vi "Doppler.vi"(0 "Choose Directory":path=path "F:/VectorFlowMice") -> ()   [LabVIEW 2022 SP3]
uses:
  <vilib>/Math Plots/3D Math Plots/3D Surface/3D Surface XCtrl/3D Surface.xctl
  -planewaveSubs/DopplerParams.ctl
  -planewaveSubs/DopThresholds.ctl
  ViewData/-ReadEye/Header.ctl
  <vilib>/Analysis/baseanly.llb/Mean (DBL).vi
  <vilib>/Analysis/baseanly.llb/Quick Scale 1D.vi
  <vilib>/Analysis/2dsp.llb/2D Cross Correlation (DBL).vi
  <vilib>/Analysis/2dsp.llb/FFT.vi
  <vilib>/Analysis/2dsp.llb/Complex FFT.vi
  <vilib>/Analysis/8numeric.llb/Numeric Integration.vi
  <vilib>/Analysis/8numeric.llb/1D Numeric Integration.vi
  <vilib>/Analysis/4window.llb/Hamming Window.vi
  <vilib>/Analysis/4window.llb/Hamming Window (CDB).vi
  -planewaveSubs/LagOneAutoCorr.vi
  <vilib>/Analysis/4window.llb/AllCosWindow (CDB).vi
  <vilib>/Analysis/1siggen.llb/Ramp Pattern by Delta.vi
  <vilib>/Analysis/3filter.llb/Butterworth Filter.vi
  <vilib>/Analysis/3filter.llb/Butterworth Filter (CDB).vi
  <vilib>/Analysis/3filter.llb/Equi-Ripple HighPass.vi
  <vilib>/Analysis/3filter.llb/Equi-Ripple HighPass (CDB).vi
  <vilib>/picture/picture.llb/Draw True-Color Pixmap.vi
  <vilib>/Utility/file.llb/Write Delimited Spreadsheet (DBL).vi
  <vilib>/Utility/file.llb/Write Delimited Spreadsheet (string).vi
  <vilib>/Math Plots/3D Math Plots/3D Surface/3D Surface Datatype/Public/Plot Helper (Matrix).vi
  <vilib>/Analysis/NI_AALBase.lvlib
  <vilib>/Analysis/NI_AALPro.lvlib
  <vilib>/Analysis/NI_AAL_SigProc.lvlib
  <vilib>/Math Plots/3D Math Plots/3D Surface/3D Surface Datatype/3D Surface Datatype.lvclass
panel:
  out "PowerRaw":sgl[][](array[numeric])
  out "Original Fc":sgl
  in  "True Center Freq":dbl=15.5
  in  "file ext search":string="*_HeaderInfoRcv.txt"
  in  "Header Out":T1={"header info"={"Header"="", "Head length"=0}, "A/D info"={"# rf points per line"=0, "# lines per scan"=0, "sample rate MHz"=0, "# A/D bits"=0, "# bytes per A/D"=0, "TGC Flag"=0, "A/D Type"=""}, "Tranducer Info"={"bandwidth"=0.0, "center freq"=0.0, "start freq"=0.0, "ID"=0}, "Scan Info"={"delay"=0.0, "pivot distance"=0.0, "sector scan angle"=0.0, "operator"="", "Scan Mode"="", "location"=""}, "Time/Date Info"={"date"="", "time"=""}, "RF Info"={"RF file name"="", "RF file att"="", "RF cal file name"="", "RF cal file att"=""}, "Patient Info"={"ID"="", "extended ID"="", "age"=0, "sex"="", "previously\nscanned"="", "PSA"=0.0, "LOS"=1, "Ethnicty 2"=3, "Race"=3}, "Tissue Type"={"organ"=0, "disease type"=0, "disease location"=0, "IQ_pts"=0, "RcvBuffer"=0, "RcvFrame"=0, "IQBuff"=0, "IQFrame"=0, "IQPage"=0}, "Votage scaling"={"Digitizer (dB)"=0.0, "Gain (dB)"=0.0, "Atten (dB)"=0.0}, "Comment"="", "Misc Info"={"avg num"=0, "c speed"=0, "Div By or SF zones"=0, "XMIT CHS"=0, "RCV CHS"=0, "Xmit angle"=0.0}, "Therapy Parameters"={"Theraputic Freq (MHz)"=0.0, "Time on (s)"=0.0, "Therapy amplitude (mV)"=0.0, "Lines Before"=0, "Lines After"=0}, "Scan Settings"={"Energy (uJ or V)"=0, "Damp (Ohm) or Fc"=0, "HP Filt (KHz)"=0, "LP Filt (MHz)"=0, "Gain (db)"=0, "prf (kHz)"=0.0, "Distance between\nscan lines (um)"=0, "Distance between\nscan planes (um)"=0, "Scan line gap (um)"=0.0, "Scan plane gap (um)"=0.0}, "Compression Parameters"={"F1 (MHz)"=0.0, "F2 (MHz)"=0.0, "% taper"=0.0, "duration"=0.0}, "Patient Info Xtra"={"First Name"="", "Last Name"="", "Notes"=""}, "ROI Box"=[0, 0, 0, 0]} {"Compression Parameters"."% taper" min=50 max=1000 format="%.2f"; "Compression Parameters"."F2 (MHz)" format="%.3f"; "Compression Parameters"."F1 (MHz)" format="%.3f"; "Scan Settings"."prf (kHz)" format="%.2f"; "Therapy Parameters"."Therapy amplitude (mV)" min=50 max=1000 format="%.2f"; "Therapy Parameters"."Time on (s)" format="%.3f"; "Therapy Parameters"."Theraputic Freq (MHz)" format="%.3f"; "Patient Info"."Race" items=["Am Ind or Alaska", "Asian", "Hawaiian, Pac Isl", "Black or Afr Amer", "White", "more than one race", "unknown"]; "Patient Info"."Ethnicty 2" items=["Hispanic", "Non-Hispanic", "unknown"]; "Patient Info"."LOS" items=["1", "2", "3", "4", "5"]; "Patient Info"."PSA" format="%.1f"; "Scan Info"."delay" format="%.2f"; "Scan Info"."pivot distance" format="%.2f"; "Scan Info"."sector scan angle" format="%.2f"; "Tranducer Info"."bandwidth" format="%.2f"; "Tranducer Info"."center freq" format="%.2f"; "Tranducer Info"."start freq" format="%.2f"}
  in  "Use Selected Files":bool
  in  "File Select":i32[](listbox)
  out "max value":sgl
  in  "RF Average Window":i32=3
  out "max doppler\nV cm/s":dbl
  out "Slow time\nsampling":sgl
  in  "image to display":i32
  in  "start":i32
  in  "Doppler Params":T2={"Dopp Filter Order"=133, "Window length"=64, "Window Increment"=8, "Start f"=0.05, "lDoppler cutouff"=0.1, "FFT Length"=128, "SlowTime (Hz)"=100.0} {"Start f" format="%0.3f"; "SlowTime (Hz)" format="%0.1f"; "lDoppler cutouff" format="%0.3f"}
  out "Total Files":i32
  in  "# of files":i32=1000
  out "Raw data":dbl[][](graph)
  in  "Tab Control":T3(tab)
  in  "Alias Correct":bool
  in  "Save Vels":bool
  in  "SaveSpectrogram":bool
  in  "phase scale":dbl=1.0
  out "phase":dbl[][](graph)
  out "Spectrum":dbl[](graph)
  out "Velocity":dbl[](graph)
  in  "Thresholds":T4={"Spec Ratio Threshold"=0.2999999999999998, "V Threshold"=-25.0, "Power Threshold"=0.0, "RF Threshold"=25000.0}
  out "Total Power":sgl[](graph)
  out "Spec ratio":sgl[](graph)
  out "Row Cropped data":dbl[][](graph)
  out "Slow time of red line":dbl[][](graph)
  out "Doppler Signal":dbl[][](graph)
  out "Dop Spec":dbl[][](graph)
  in  "SVD zeros":i32
  in  "SVD?":bool
  in  "maxPRF?":bool
  in  "Log RF?":bool=TRUE
  out "bandwidths":sgl[](graph)
  out "error":i32
  in  "Clip":i32
  out "Vel Mean":dbl format="%0.2f"
  out "Sum Power":sgl
  in  "Lag Overlay off?":bool
  out "BPM":i32
  in  "Cycles":i32=1
  in  "width":i32=25 min=3
  in  "threshold":dbl=0.35 format="%0.2f"
  in  "Batch BPM":bool
  out "# found":i32[](array[numeric])
  out "BPM auto":i32[](array[numeric])
  in  "Freeze BPM":bool
  out "BPS":sgl
  in  "Note":string
  out "LagOne":dbl
  in  "Save Single SpGram":bool
  in  "Save Animation":bool
  out "Slow time mean":dbl[](graph)
  out "Spectrogram at marker":sgl[][](graph)
  out "Slow Time V values at Red cursor":dbl[](graph)
  in  "Scale Type":enum32{"Max/Min", "Max/Zero", "Min/Zero"}(radio)
  out "Peak V":dbl[][](graph)
  in  "animate":bool
  in  "ms between frames":u32=10
  in  "Calc Spec Peaks":bool
  out "AVG of all windows":dbl[][](graph)
  in  "Doppler Angle":dbl
  in  "AVG Thresh":dbl=20.0
  out "V mean":dbl format="%0.2f"
  out "V SD":dbl format="%0.2f"
  in  "Z Scale":dbl(slide) scale=0.0..50.0
  in  "Queue processing":bool
  out "Overlay":i16[][](graph)
  in  "dB Max":dbl=50.0
  in  "Med Size":i32=3
  in  "Spectrogram average":i32=3
  out "Dop Spectrum":sgl[](graph)
  in  "dB width pt":dbl
  in  "ST AV depth":i32=10
  out "Sets":i32
  out "Current":i32
  out "Raw uncropped image":dbl[][](graph)
  out "Waveform Graph":i32[](graph)
  out "2D corr":dbl[][](graph)
  out "Mean Power":sgl[][](graph)
  out "Slow Time V values at Red cursor Mean Power":dbl[](graph)
  out "Simple Motion Tracker":cluster{"2D Corr":dbl[], "2D Corr":dbl[]}(graph)
  in  "#x lines":i32=10
  in  "#y rf":i32=25
  in  "Ref Place for 2S":i32
  in  "2D threshold":sgl
  in  "Save Motion":bool
  out "M-mode x":dbl[][](graph)
  in  "Save M-mode":bool
  in  "Divide down":i32=50 min=1
  out "Avergae V Profile All":dbl[](graph)
  out "Avergae V Profile (Tube)":dbl[](graph)
  in  "index":i32
  in  "length":i32
  out "3D Surface":refnum<class "3D Plot Datatype.lvclass">[](xcontrol)
  out "High pass Filtered log":sgl[][](graph)
  in  "CFiltered data":bool
  in  "C Corr":bool
  out "Cross Correlate":sgl[][](graph)
  out "Cross Correlate":sgl[][][](array[numeric])
  out "HIgh pass Filtered X":sgl[][][](array[numeric])
  out "Raw High pass filtered":sgl[][](graph)
  out "Row Cropped data save":dbl[][](graph)
  out "Doppler Spec For Save":dbl[][](graph)
  out "Smoothed Data":dbl[][][](array[numeric])
  out "Raw Complex output array":csg[][][](array[numeric])
  out "Overlay 3D":i16[][][](array[numeric])
  out "AVG Vel":dbl[][][](array[numeric])
  in  "save spectorgrams":bool
  out "Paths to process":path[](array[path])=[path "\\\\Vantage-n-wk\\h/process bundle/VectorFlow Mouse Day 1 2017-07-14/2017-07-14 9412_WT/sTx7_41_0C_9412_WT_Lx_HV_07A_10D_04286Hz_16MHz_0933mS_00_EYE", path "\\\\Vantage-n-wk\\h/process bundle/VectorFlow Mouse Day 1 2017-07-14/2017-07-14 9415_KO/sTX3_37C_9415_KO_Lx_03A_10D_10000Hz_16MHz_1000mS_00_EYE", path "\\\\Vantage-n-wk\\h/process bundle/VectorFlow Mouse Day 1 2017-07-14/2017-07-14 9415_KO/sTX3_37C_9415_KO_Lx_HV_03A_10D_10000Hz_16MHz_1000mS_00_EYE", path "\\\\Vantage-n-wk\\h/process bundle/VectorFlow Mouse Day 1 2017-07-14/2017-07-14 9415_KO/sTX3_37C_9415_KO_Lx_HV_2_03A_10D_10000Hz_16MHz_0520mS_00_EYE", path "\\\\Vantage-n-wk\\h/process bundle/VectorFlow Mouse Day 1 2017-07-14/2017-07-14 9415_KO/sTX3_37C_9415_KO_Lx_HV_2_03A_10D_10000Hz_16MHz_1000mS_00_EYE", path "\\\\Vantage-n-wk\\h/process bundle/VectorFlow Mouse Day 1 2017-07-14/2017-07-14 9415_KO/sTx3_41_7C_9415_KO_Lx_HV_03A_10D_10000Hz_16MHz_1000mS_00_EYE", path "\\\\Vantage-n-wk\\h/process bundle/VectorFlow Mouse Day 1 2017-07-14/2017-07-14 9415_KO/sTX7_37C_9415_KO_Lx_HV_07A_10D_04286Hz_16MHz_0933mS_00_EYE", path "\\\\Vantage-n-wk\\h/process bundle/VectorFlow Mouse Day 1 2017-07-14/2017-07-14 9415_KO/sTx7_37C_9415_KO_Lx_HV_2_07A_10D_04286Hz_16MHz_0933mS_00_EYE", path "\\\\Vantage-n-wk\\h/process bundle/VectorFlow Mouse Day 1 2017-07-14/2017-07-14 9415_KO/sTx7_39_5C_9415_KO_Lx_HV_07A_10D_04286Hz_16MHz_0933mS_00_EYE", path "\\\\Vantage-n-wk\\h/process bundle/VectorFlow Mouse Day 1 2017-07-14/2017-07-14 9415_KO/sTx7_40_5C_9415_KO_Lx_HV_07A_10D_04286Hz_16MHz_0933mS_00_EYE", path "\\\\Vantage-n-wk\\h/process bundle/VectorFlow Mouse Day 1 2017-07-14/2017-07-14 9415_KO/sTx7_41_2C_9415_KO_Lx_HV_07A_10D_04286Hz_16MHz_0933mS_00_EYE", path "\\\\Vantage-n-wk\\h/process bundle/VectorFlow Mouse Day 1 2017-07-14/2017-07-14 9415_KO/sTx7_41_7C_9415_KO_Lx_HV_07A_10D_04286Hz_16MHz_0933mS_00_EYE", path "\\\\Vantage-n-wk\\h/process bundle/VectorFlow Mouse Day 1 2017-07-14/2017-07-14 9415_KO/sTx7_42_0C_9415_KO_Lx_HV_07A_10D_04286Hz_16MHz_0933mS_00_EYE", path "\\\\Vantage-n-wk\\h/process bundle/VectorFlow Mouse Day 1 2017-07-14/2017-07-14 9416_KO/sTx3_37_3C_9416_KO_Lx_HV_03A_10D_10000Hz_16MHz_1000mS_00_EYE", path "\\\\Vantage-n-wk\\h/process bundle/VectorFlow Mouse Day 1 2017-07-14/2017-07-14 9416_KO/sTx3_37_6C_9416_KO_Lx_HV_03A_10D_10000Hz_16MHz_1000mS_00_EYE", path "\\\\Vantage-n-wk\\h/process bundle/VectorFlow Mouse Day 1 2017-07-14/2017-07-14 9416_KO/sTx3_38_1C_9416_KO_Lx_HV_03A_10D_10000Hz_16MHz_1000mS_00_EYE", path "\\\\Vantage-n-wk\\h/process bundle/VectorFlow Mouse Day 1 2017-07-14/2017-07-14 9416_KO/sTx3_39_0C_9416_KO_Lx_HV_03A_10D_10000Hz_16MHz_1000mS_00_EYE", path "\\\\Vantage-n-wk\\h/process bundle/VectorFlow Mouse Day 1 2017-07-14/2017-07-14 9416_KO/sTx3_40_0C_9416_KO_Lx_HV_03A_10D_10000Hz_16MHz_1000mS_00_EYE", path "\\\\Vantage-n-wk\\h/process bundle/VectorFlow Mouse Day 1 2017-07-14/2017-07-14 9416_KO/sTx3_40_5C_9416_KO_Lx_HV_03A_10D_10000Hz_16MHz_1000mS_00_EYE", path "\\\\Vantage-n-wk\\h/process bundle/VectorFlow Mouse Day 1 2017-07-14/2017-07-14 9416_KO/sTx3_41_0C_9416_KO_Lx_HV_03A_10D_10000Hz_16MHz_1000mS_00_EYE", path "\\\\Vantage-n-wk\\h/process bundle/VectorFlow Mouse Day 1 2017-07-14/2017-07-14 9416_KO/sTx3_41_3C_9416_KO_Lx_HV_03A_10D_10000Hz_16MHz_1000mS_00_EYE", path "\\\\Vantage-n-wk\\h/process bundle/VectorFlow Mouse Day 1 2017-07-14/2017-07-14 9416_KO/sTx7_36_6C_9416_KO_Lx_HV_07A_10D_04286Hz_16MHz_0933mS_00_EYE", path "\\\\Vantage-n-wk\\h/process bundle/VectorFlow Mouse Day 1 2017-07-14/2017-07-14 9416_KO/sTx7_37_5C_9416_KO_Lx_HV_07A_10D_04286Hz_16MHz_0933mS_00_EYE", path "\\\\Vantage-n-wk\\h/process bundle/VectorFlow Mouse Day 1 2017-07-14/2017-07-14 9416_KO/sTx7_38_2C_9416_KO_Lx_HV_07A_10D_04286Hz_16MHz_0933mS_00_EYE", path "\\\\Vantage-n-wk\\h/process bundle/VectorFlow Mouse Day 1 2017-07-14/2017-07-14 9416_KO/sTx7_41_0C_9416_KO_Lx_HV_07A_10D_04286Hz_16MHz_0933mS_00_EYE", path "\\\\Vantage-n-wk\\h/process bundle/VectorFlow Mouse Day 2 2018-01-25/2018-01-25 KO 10129/10129_35p5C_KO_Lx_HV_sTx03A_20D_10000Hz_18MHz_1000mS_00_EYE", path "\\\\Vantage-n-wk\\h/process bundle/VectorFlow Mouse Day 2 2018-01-25/2018-01-25 KO 10129/10129_35p7C_KO_Lx_HV_sTx03A_20D_10000Hz_18MHz_1000mS_00_EYE", path "\\\\Vantage-n-wk\\h/process bundle/VectorFlow Mouse Day 2 2018-01-25/2018-01-25 KO 10129/10129_36p5C_KO_Lx_HV_sTx03A_20D_10000Hz_18MHz_1000mS_00_EYE", path "\\\\Vantage-n-wk\\h/process bundle/VectorFlow Mouse Day 2 2018-01-25/2018-01-25 KO 10129/10129_37p0C_KO_Lx_HV_sTx03A_20D_10000Hz_18MHz_1000mS_00_EYE", path "\\\\Vantage-n-wk\\h/process bundle/VectorFlow Mouse Day 2 2018-01-25/2018-01-25 KO 10129/10129_37p0C_KO_Lx_HV_sTx03A_20D_10000Hz_18MHz_1000mS_01_EYE", path "\\\\Vantage-n-wk\\h/process bundle/VectorFlow Mouse Day 2 2018-01-25/2018-01-25 KO 10129/10129_37p5C_KO_Lx_HV_sTx03A_20D_10000Hz_18MHz_1000mS_01_EYE", path "\\\\Vantage-n-wk\\h/process bundle/VectorFlow Mouse Day 2 2018-01-25/2018-01-25 KO 10129/10129_38p0C_KO_Lx_HV_sTx03A_20D_10000Hz_18MHz_1000mS_00_EYE", path "\\\\Vantage-n-wk\\h/process bundle/VectorFlow Mouse Day 2 2018-01-25/2018-01-25 KO 10129/10129_38p5C_KO_Lx_HV_sTx03A_20D_10000Hz_18MHz_1000mS_00_EYE", path "\\\\Vantage-n-wk\\h/process bundle/VectorFlow Mouse Day 2 2018-01-25/2018-01-25 KO 10129/10129_38p5C_KO_Lx_HV_sTx03A_20D_10000Hz_18MHz_1000mS_01_EYE", path "\\\\Vantage-n-wk\\h/process bundle/VectorFlow Mouse Day 2 2018-01-25/2018-01-25 KO 10129/10129_39p5C_KO_Lx_HV_sTx03A_20D_10000Hz_18MHz_1000mS_00_EYE", path "\\\\Vantage-n-wk\\h/process bundle/VectorFlow Mouse Day 2 2018-01-25/2018-01-25 KO 10129/10129_40p0C_KO_Lx_HV_sTx03A_20D_10000Hz_18MHz_1000mS_00_EYE", path "\\\\Vantage-n-wk\\h/process bundle/VectorFlow Mouse Day 2 2018-01-25/2018-01-25 KO 10129/10129_40p0C_KO_Lx_HV_sTx03A_20D_10000Hz_18MHz_1000mS_01_EYE", path "\\\\Vantage-n-wk\\h/process bundle/VectorFlow Mouse Day 2 2018-01-25/2018-01-25 KO 10129/10129_40p5C_KO_Lx_HV_sTx03A_20D_10000Hz_18MHz_1000mS_00_EYE", path "\\\\Vantage-n-wk\\h/process bundle/VectorFlow Mouse Day 2 2018-01-25/2018-01-25 KO 10129/10129_41p0C_KO_Lx_HV_sTx03A_20D_10000Hz_18MHz_1000mS_00_EYE", path "\\\\Vantage-n-wk\\h/process bundle/VectorFlow Mouse Day 2 2018-01-25/2018-01-25 KO 10129/10129_41p0C_KO_Lx_HV_sTx03A_20D_10000Hz_18MHz_1000mS_01_EYE", path "\\\\Vantage-n-wk\\h/process bundle/VectorFlow Mouse Day 2 2018-01-25/2018-01-25 KO 10176/10176_36p5C_KO_Lx_HV_sTx03A_20D_10000Hz_18MHz_1000mS_00_EYE", path "\\\\Vantage-n-wk\\h/process bundle/VectorFlow Mouse Day 2 2018-01-25/2018-01-25 KO 10176/10176_37C_KO_Lx_HV_sTx03A_20D_10000Hz_18MHz_1000mS_00_EYE", path "\\\\Vantage-n-wk\\h/process bundle/VectorFlow Mouse Day 2 2018-01-25/2018-01-25 KO 10176/10176_37C_KO_Lx_HV_sTx03A_20D_10000Hz_18MHz_1000mS_01_EYE", path "\\\\Vantage-n-wk\\h/process bundle/VectorFlow Mouse Day 2 2018-01-25/2018-01-25 KO 10176/10176_37C_KO_Lx_HV_sTx03A_20D_10000Hz_18MHz_1000mS_02_EYE", path "\\\\Vantage-n-wk\\h/process bundle/VectorFlow Mouse Day 2 2018-01-25/2018-01-25 KO 10176/10176_37C_KO_Lx_HV_sTx03A_20D_10000Hz_18MHz_1000mS_03_EYE", path "\\\\Vantage-n-wk\\h/process bundle/VectorFlow Mouse Day 2 2018-01-25/2018-01-25 KO 10176/10176_37C_KO_Lx_HV_sTx03A_20D_10000Hz_18MHz_1000mS_04_EYE", path "\\\\Vantage-n-wk\\h/process bundle/VectorFlow Mouse Day 2 2018-01-25/2018-01-25 KO 10176/10176_37p0C_KO_Lx_HV_sTx03A_20D_10000Hz_18MHz_1000mS_00_EYE", path "\\\\Vantage-n-wk\\h/process bundle/VectorFlow Mouse Day 2 2018-01-25/2018-01-25 KO 10176/10176_37p5C_KO_Lx_HV_sTx03A_20D_10000Hz_18MHz_1000mS_00_EYE", path "\\\\Vantage-n-wk\\h/process bundle/VectorFlow Mouse Day 2 2018-01-25/2018-01-25 KO 10176/10176_38C_KO_Lx_HV_sTx03A_20D_10000Hz_18MHz_1000mS_00_EYE", path "\\\\Vantage-n-wk\\h/process bundle/VectorFlow Mouse Day 2 2018-01-25/2018-01-25 KO 10176/10176_38p0C_KO_Lx_HV_sTx03A_20D_10000Hz_18MHz_1000mS_00_EYE", path "\\\\Vantage-n-wk\\h/process bundle/VectorFlow Mouse Day 2 2018-01-25/2018-01-25 KO 10176/10176_38p5C_KO_Lx_HV_sTx03A_20D_10000Hz_18MHz_1000mS_00_EYE", path "\\\\Vantage-n-wk\\h/process bundle/VectorFlow Mouse Day 2 2018-01-25/2018-01-25 KO 10176/10176_39C_KO_Lx_HV_sTx03A_20D_10000Hz_18MHz_1000mS_00_EYE", path "\\\\Vantage-n-wk\\h/process bundle/VectorFlow Mouse Day 2 2018-01-25/2018-01-25 KO 10176/10176_39C_KO_Lx_HV_sTx03A_20D_10000Hz_18MHz_1000mS_01_EYE", path "\\\\Vantage-n-wk\\h/process bundle/VectorFlow Mouse Day 2 2018-01-25/2018-01-25 KO 10176/10176_39C_KO_Lx_HV_sTx03A_20D_10000Hz_18MHz_1000mS_02_EYE", path "\\\\Vantage-n-wk\\h/process bundle/VectorFlow Mouse Day 2 2018-01-25/2018-01-25 KO 10176/10176_39p0C_KO_Lx_HV_sTx03A_20D_10000Hz_18MHz_1000mS_00_EYE", path "\\\\Vantage-n-wk\\h/process bundle/VectorFlow Mouse Day 2 2018-01-25/2018-01-25 KO 10176/10176_39p5C_KO_Lx_HV_sTx03A_20D_10000Hz_18MHz_1000mS_00_EYE", path "\\\\Vantage-n-wk\\h/process bundle/VectorFlow Mouse Day 2 2018-01-25/2018-01-25 KO 10176/10176_39p5C_KO_Lx_HV_sTx03A_20D_10000Hz_18MHz_1000mS_01_EYE", path "\\\\Vantage-n-wk\\h/process bundle/VectorFlow Mouse Day 2 2018-01-25/2018-01-25 KO 10177/10177_35p5C_KO_Lx_HV_sTx03A_20D_20000Hz_18MHz_1000mS_00_EYE", path "\\\\Vantage-n-wk\\h/process bundle/VectorFlow Mouse Day 2 2018-01-25/2018-01-25 KO 10177/10177_35p5C_KO_Lx_HV_sTx03A_20D_20000Hz_18MHz_1000mS_01_EYE", path "\\\\Vantage-n-wk\\h/process bundle/VectorFlow Mouse Day 2 2018-01-25/2018-01-25 KO 10177/10177_35p5C_KO_Lx_HV_sTx03A_20D_20000Hz_18MHz_1000mS_02_EYE", path "\\\\Vantage-n-wk\\h/process bundle/VectorFlow Mouse Day 2 2018-01-25/2018-01-25 KO 10177/10177_35p5C_KO_Lx_HV_sTx03A_20D_20000Hz_18MHz_1000mS_03_EYE", path "\\\\Vantage-n-wk\\h/process bundle/VectorFlow Mouse Day 2 2018-01-25/2018-01-25 KO 10177/10177_36p0C_KO_Lx_HV_sTx03A_20D_20000Hz_18MHz_1000mS_00_EYE", path "\\\\Vantage-n-wk\\h/process bundle/VectorFlow Mouse Day 2 2018-01-25/2018-01-25 KO 10177/10177_36p5C_KO_Lx_HV_sTx03A_20D_20000Hz_18MHz_1000mS_00_EYE", path "\\\\Vantage-n-wk\\h/process bundle/VectorFlow Mouse Day 2 2018-01-25/2018-01-25 KO 10177/10177_37p0C_KO_Lx_HV_sTx03A_20D_20000Hz_18MHz_1000mS_00_EYE", path "\\\\Vantage-n-wk\\h/process bundle/VectorFlow Mouse Day 2 2018-01-25/2018-01-25 KO 10177/10177_37p0C_KO_Lx_HV_sTx03A_20D_20000Hz_18MHz_1000mS_01_EYE", path "\\\\Vantage-n-wk\\h/process bundle/VectorFlow Mouse Day 2 2018-01-25/2018-01-25 KO 10177/10177_37p5C_KO_Lx_HV_sTx03A_20D_20000Hz_18MHz_1000mS_00_EYE", path "\\\\Vantage-n-wk\\h/process bundle/VectorFlow Mouse Day 2 2018-01-25/2018-01-25 KO 10177/10177_38p0C_KO_Lx_HV_sTx03A_20D_20000Hz_18MHz_1000mS_00_EYE", path "\\\\Vantage-n-wk\\h/process bundle/VectorFlow Mouse Day 2 2018-01-25/2018-01-25 KO 10177/10177_38p0C_KO_Lx_HV_sTx03A_20D_20000Hz_18MHz_1000mS_01_EYE", path "\\\\Vantage-n-wk\\h/process bundle/VectorFlow Mouse Day 2 2018-01-25/2018-01-25 KO 10177/10177_38p5C_KO_Lx_HV_sTx03A_20D_20000Hz_18MHz_1000mS_00_EYE", path "\\\\Vantage-n-wk\\h/process bundle/VectorFlow Mouse Day 2 2018-01-25/2018-01-25 KO 10177/10177_39p0C_KO_Lx_HV_sTx03A_20D_20000Hz_18MHz_1000mS_00_EYE", path "\\\\Vantage-n-wk\\h/process bundle/VectorFlow Mouse Day 2 2018-01-25/2018-01-25 KO 10177/10177_39p0C_KO_Lx_HV_sTx03A_20D_20000Hz_18MHz_1000mS_01_EYE", path "\\\\Vantage-n-wk\\h/process bundle/VectorFlow Mouse Day 2 2018-01-25/2018-01-25 KO 10177/10177_39p5C_KO_Lx_HV_sTx03A_20D_20000Hz_18MHz_1000mS_00_EYE", path "\\\\Vantage-n-wk\\h/process bundle/VectorFlow Mouse Day 2 2018-01-25/2018-01-25 KO 10177/10177_39p5C_KO_Lx_HV_sTx03A_20D_20000Hz_18MHz_1000mS_01_EYE", path "\\\\Vantage-n-wk\\h/process bundle/VectorFlow Mouse Day 2 2018-01-25/2018-01-25 KO 10177/10177_40p0C_KO_Lx_HV_sTx03A_20D_20000Hz_18MHz_1000mS_00_EYE", path "\\\\Vantage-n-wk\\h/process bundle/VectorFlow Mouse Day 2 2018-01-25/2018-01-25 KO 10177/10177_40p0C_KO_Lx_HV_sTx03A_20D_20000Hz_18MHz_1000mS_01_EYE", path "\\\\Vantage-n-wk\\h/process bundle/VectorFlow Mouse Day 2 2018-01-25/2018-01-25 KO 10177/10177_40p5C_KO_Lx_HV_sTx03A_20D_20000Hz_18MHz_1000mS_00_EYE", path "\\\\Vantage-n-wk\\h/process bundle/VectorFlow Mouse Day 2 2018-01-25/2018-01-25 KO 10177/10177_40p5C_KO_Lx_HV_sTx03A_20D_20000Hz_18MHz_1000mS_01_EYE", path "\\\\Vantage-n-wk\\h/process bundle/VectorFlow Mouse Day 2 2018-01-25/2018-01-25 KO 10177/10177_41p0C_KO_Lx_HV_sTx03A_20D_20000Hz_18MHz_1000mS_00_EYE", path "\\\\Vantage-n-wk\\h/process bundle/VectorFlow Mouse Day 2 2018-01-25/2018-01-25 KO 10177/10177_41p0C_KO_Lx_HV_sTx03A_20D_20000Hz_18MHz_1000mS_01_EYE", path "\\\\Vantage-n-wk\\h/process bundle/VectorFlow Mouse Day 2 2018-01-25/2018-01-25 KO 10177/10177_41p0C_KO_Lx_HV_sTx03A_20D_20000Hz_18MHz_1000mS_02_EYE", path "\\\\Vantage-n-wk\\h/process bundle/VectorFlow Mouse Day 2 2018-01-25/2018-01-25 KO 10177/10177_41p0C_KO_Lx_HV_sTx03A_20D_20000Hz_18MHz_1000mS_03_EYE", path "\\\\Vantage-n-wk\\h/process bundle/VectorFlow Mouse Day 2 2018-01-25/2018-01-25 KO 10178/10178_34p0C_KO_Lx_HV_sTx03A_20D_20000Hz_18MHz_1000mS_00_EYE", path "\\\\Vantage-n-wk\\h/process bundle/VectorFlow Mouse Day 2 2018-01-25/2018-01-25 KO 10178/10178_34p5C_KO_Lx_HV_sTx03A_20D_20000Hz_18MHz_1000mS_00_EYE", path "\\\\Vantage-n-wk\\h/process bundle/VectorFlow Mouse Day 2 2018-01-25/2018-01-25 KO 10178/10178_35p0C_KO_Lx_HV_sTx03A_20D_20000Hz_18MHz_1000mS_00_EYE", path "\\\\Vantage-n-wk\\h/process bundle/VectorFlow Mouse Day 2 2018-01-25/2018-01-25 KO 10178/10178_35p5C_KO_Lx_HV_sTx03A_20D_20000Hz_18MHz_1000mS_00_EYE", path "\\\\Vantage-n-wk\\h/process bundle/VectorFlow Mouse Day 2 2018-01-25/2018-01-25 KO 10178/10178_35p5C_KO_Lx_HV_sTx03A_20D_20000Hz_18MHz_1000mS_01_EYE", path "\\\\Vantage-n-wk\\h/process bundle/VectorFlow Mouse Day 2 2018-01-25/2018-01-25 KO 10178/10178_36p0C_KO_Lx_HV_sTx03A_20D_20000Hz_18MHz_1000mS_00_EYE", path "\\\\Vantage-n-wk\\h/process bundle/VectorFlow Mouse Day 2 2018-01-25/2018-01-25 KO 10178/10178_36p5C_KO_Lx_HV_sTx03A_20D_20000Hz_18MHz_1000mS_00_EYE", path "\\\\Vantage-n-wk\\h/process bundle/VectorFlow Mouse Day 2 2018-01-25/2018-01-25 KO 10178/10178_37p0C_KO_Lx_HV_sTx03A_20D_20000Hz_18MHz_1000mS_00_EYE", path "\\\\Vantage-n-wk\\h/process bundle/VectorFlow Mouse Day 2 2018-01-25/2018-01-25 KO 10178/10178_37p5C_KO_Lx_HV_sTx03A_20D_20000Hz_18MHz_1000mS_00_EYE", path "\\\\Vantage-n-wk\\h/process bundle/VectorFlow Mouse Day 2 2018-01-25/2018-01-25 KO 10178/10178_37p5C_KO_Lx_HV_sTx03A_20D_20000Hz_18MHz_1000mS_01_EYE", path "\\\\Vantage-n-wk\\h/process bundle/VectorFlow Mouse Day 2 2018-01-25/2018-01-25 KO 10178/10178_37p5C_KO_Lx_HV_sTx03A_20D_20000Hz_18MHz_1000mS_02_EYE", path "\\\\Vantage-n-wk\\h/process bundle/VectorFlow Mouse Day 2 2018-01-25/2018-01-25 KO 10178/10178_37p5C_KO_Lx_HV_sTx03A_20D_20000Hz_18MHz_1000mS_03_EYE", path "\\\\Vantage-n-wk\\h/process bundle/VectorFlow Mouse Day 2 2018-01-25/2018-01-25 KO 10178/10178_38p0C_KO_Lx_HV_sTx03A_20D_20000Hz_18MHz_1000mS_00_EYE", path "\\\\Vantage-n-wk\\h/process bundle/VectorFlow Mouse Day 2 2018-01-25/2018-01-25 KO 10178/10178_39p0C_KO_Lx_HV_sTx03A_20D_20000Hz_18MHz_1000mS_00_EYE", path "\\\\Vantage-n-wk\\h/process bundle/VectorFlow Mouse Day 2 2018-01-25/2018-01-25 KO 10178/10178_39p5C_KO_Lx_HV_sTx03A_20D_20000Hz_18MHz_1000mS_00_EYE", path "\\\\Vantage-n-wk\\h/process bundle/VectorFlow Mouse Day 2 2018-01-25/2018-01-25 KO 10178/10178_39p5C_KO_Lx_HV_sTx03A_20D_20000Hz_18MHz_1000mS_01_EYE", path "\\\\Vantage-n-wk\\h/process bundle/VectorFlow Mouse Day 2 2018-01-25/2018-01-25 KO 10178/10178_40p0C_KO_Lx_HV_sTx03A_20D_20000Hz_18MHz_1000mS_00_EYE", path "\\\\Vantage-n-wk\\h/process bundle/VectorFlow Mouse Day 2 2018-01-25/2018-01-25 KO 10178/10178_40p5C_KO_Lx_HV_sTx03A_20D_20000Hz_18MHz_1000mS_00_EYE", path "\\\\Vantage-n-wk\\h/process bundle/VectorFlow Mouse Day 2 2018-01-25/2018-01-25 WT 10130/10130_36p5C_WT_Lx_HV_sTx03A_20D_10000Hz_18MHz_1000mS_00_EYE", path "\\\\Vantage-n-wk\\h/process bundle/VectorFlow Mouse Day 2 2018-01-25/2018-01-25 WT 10130/10130_36p5C_WT_Lx_HV_sTx03A_20D_10000Hz_18MHz_1000mS_01_EYE", path "\\\\Vantage-n-wk\\h/process bundle/VectorFlow Mouse Day 2 2018-01-25/2018-01-25 WT 10130/10130_36p5C_WT_Lx_HV_sTx03A_20D_10000Hz_18MHz_1000mS_02_EYE", path "\\\\Vantage-n-wk\\h/process bundle/VectorFlow Mouse Day 2 2018-01-25/2018-01-25 WT 10130/10130_37p0C_WT_Lx_HV_sTx03A_20D_10000Hz_18MHz_1000mS_00_EYE", path "\\\\Vantage-n-wk\\h/process bundle/VectorFlow Mouse Day 2 2018-01-25/2018-01-25 WT 10130/10130_37p5C_WT_Lx_HV_sTx03A_20D_10000Hz_18MHz_1000mS_00_EYE", path "\\\\Vantage-n-wk\\h/process bundle/VectorFlow Mouse Day 2 2018-01-25/2018-01-25 WT 10130/10130_38p0C_WT_Lx_HV_sTx03A_20D_10000Hz_18MHz_1000mS_00_EYE", path "\\\\Vantage-n-wk\\h/process bundle/VectorFlow Mouse Day 2 2018-01-25/2018-01-25 WT 10130/10130_38p0C_WT_Lx_HV_sTx03A_20D_10000Hz_18MHz_1000mS_01_EYE", path "\\\\Vantage-n-wk\\h/process bundle/VectorFlow Mouse Day 2 2018-01-25/2018-01-25 WT 10130/10130_39p0C_WT_Lx_HV_sTx03A_20D_10000Hz_18MHz_1000mS_00_EYE", path "\\\\Vantage-n-wk\\h/process bundle/VectorFlow Mouse Day 2 2018-01-25/2018-01-25 WT 10130/10130_40p0C_WT_Lx_HV_sTx03A_20D_10000Hz_18MHz_1000mS_00_EYE", path "\\\\Vantage-n-wk\\h/process bundle/VectorFlow Mouse Day 2 2018-01-25/2018-01-25 WT 10130/10130_40p5C_WT_Lx_HV_sTx03A_20D_10000Hz_18MHz_1000mS_00_EYE", path "\\\\Vantage-n-wk\\h/process bundle/VectorFlow Mouse Day 2 2018-01-25/2018-01-25 WT 10130/10130_40p5C_WT_Lx_HV_sTx03A_20D_10000Hz_18MHz_1000mS_01_EYE", path "\\\\Vantage-n-wk\\h/process bundle/VectorFlow Mouse Day 2 2018-01-25/2018-01-25 WT 10130/10130_40p5C_WT_Lx_HV_sTx03A_20D_10000Hz_18MHz_1000mS_02_EYE", path "\\\\Vantage-n-wk\\h/process bundle/VectorFlow Mouse Day 2 2018-01-25/2018-01-25 WT 10130/10130_41p0C_WT_Lx_HV_sTx03A_20D_10000Hz_18MHz_1000mS_00_EYE", path "\\\\Vantage-n-wk\\h/process bundle/VectorFlow Mouse Day 3 2018-02-09/2018-02-09 KO 10129/10129_37p0C_NO_sTx03A_20D_10000Hz_18MHz_0500mS_01_EYE", path "\\\\Vantage-n-wk\\h/process bundle/VectorFlow Mouse Day 3 2018-02-09/2018-02-09 KO 10129/10129_38p5C_NO_sTx03A_20D_10000Hz_18MHz_0500mS_00_EYE", path "\\\\Vantage-n-wk\\h/process bundle/VectorFlow Mouse Day 3 2018-02-09/2018-02-09 KO 10129/10129_39p0C_NO_sTx03A_20D_10000Hz_18MHz_0500mS_00_EYE", path "\\\\Vantage-n-wk\\h/process bundle/VectorFlow Mouse Day 3 2018-02-09/2018-02-09 KO 10129/10129_39p5C_NO_sTx03A_20D_10000Hz_18MHz_0500mS_00_EYE", path "\\\\Vantage-n-wk\\h/process bundle/VectorFlow Mouse Day 3 2018-02-09/2018-02-09 KO 10129/10129_40p0C_NO_sTx03A_20D_10000Hz_18MHz_0500mS_00_EYE", path "\\\\Vantage-n-wk\\h/process bundle/VectorFlow Mouse Day 3 2018-02-09/2018-02-09 KO 10129/10129_40p0C_NO_sTx03A_20D_10000Hz_18MHz_0500mS_01_EYE", path "\\\\Vantage-n-wk\\h/process bundle/VectorFlow Mouse Day 3 2018-02-09/2018-02-09 KO 10129/10129_40p5C_NO_sTx03A_20D_10000Hz_18MHz_0500mS_00_EYE", path "\\\\Vantage-n-wk\\h/process bundle/VectorFlow Mouse Day 3 2018-02-09/2018-02-09 KO 10129/10129_41p0C_NO_sTx03A_20D_10000Hz_18MHz_0500mS_00_EYE", path "\\\\Vantage-n-wk\\h/process bundle/VectorFlow Mouse Day 3 2018-02-09/2018-02-09 KO 10129/10129_41p2C_NO_USD_sTx03A_20D_10000Hz_18MHz_0500mS_00_EYE", path "\\\\Vantage-n-wk\\h/process bundle/VectorFlow Mouse Day 3 2018-02-09/2018-02-09 KOPF 10135/10135_34p0C_KOPF_sTx03A_10D_10000Hz_18MHz_1000mS_00_EYE", path "\\\\Vantage-n-wk\\h/process bundle/VectorFlow Mouse Day 3 2018-02-09/2018-02-09 KOPF 10135/10135_34p0C_KOPF_sTx03A_20D_10000Hz_18MHz_1000mS_00_EYE", path "\\\\Vantage-n-wk\\h/process bundle/VectorFlow Mouse Day 3 2018-02-09/2018-02-09 KOPF 10135/10135_34p0C_KOPF_sTx03A_20D_10000Hz_18MHz_1000mS_01_EYE", path "\\\\Vantage-n-wk\\h/process bundle/VectorFlow Mouse Day 3 2018-02-09/2018-02-09 KOPF 10135/10135_34p0C_KOPF_sTx03A_20D_10000Hz_18MHz_1000mS_02_EYE", path "\\\\Vantage-n-wk\\h/process bundle/VectorFlow Mouse Day 3 2018-02-09/2018-02-09 KOPF 10135/10135_34p0C_KOPF_sTx05A_10D_06000Hz_18MHz_1000mS_00_EYE", path "\\\\Vantage-n-wk\\h/process bundle/VectorFlow Mouse Day 3 2018-02-09/2018-02-09 KOPF 10135/10135_34p0C_KOPF_sTx05A_10D_06000Hz_18MHz_1000mS_01_EYE", path "\\\\Vantage-n-wk\\h/process bundle/VectorFlow Mouse Day 3 2018-02-09/2018-02-09 KOPF 10135/10135_34p0C_KOPF_sTx05A_20D_06000Hz_18MHz_1000mS_00_EYE", path "\\\\Vantage-n-wk\\h/process bundle/VectorFlow Mouse Day 3 2018-02-09/2018-02-09 KOPF 10135/10135_37p0C_KOPF_sTx03A_10D_10000Hz_18MHz_1000mS_00_EYE", path "\\\\Vantage-n-wk\\h/process bundle/VectorFlow Mouse Day 3 2018-02-09/2018-02-09 KOPF 10135/10135_37p5C_KOPF_sTx03A_10D_10000Hz_18MHz_1000mS_00_EYE", path "\\\\Vantage-n-wk\\h/process bundle/VectorFlow Mouse Day 3 2018-02-09/2018-02-09 KOPF 10135/10135_37p5C_KOPF_sTx03A_10D_10000Hz_18MHz_1000mS_01_EYE", path "\\\\Vantage-n-wk\\h/process bundle/VectorFlow Mouse Day 3 2018-02-09/2018-02-09 WT 10128/10128_37p0C_WT_sTx03A_20D_10000Hz_18MHz_0500mS_00_EYE", path "\\\\Vantage-n-wk\\h/process bundle/VectorFlow Mouse Day 3 2018-02-09/2018-02-09 WT 10128/10128_38p0C_WT_sTx03A_20D_10000Hz_18MHz_0500mS_00_EYE", path "\\\\Vantage-n-wk\\h/process bundle/VectorFlow Mouse Day 3 2018-02-09/2018-02-09 WT 10128/10128_38p0C_WT_sTx03A_20D_10000Hz_18MHz_0500mS_01_EYE", path "\\\\Vantage-n-wk\\h/process bundle/VectorFlow Mouse Day 3 2018-02-09/2018-02-09 WT 10128/10128_39p0C_WT_sTx03A_20D_10000Hz_18MHz_0500mS_00_EYE", path "\\\\Vantage-n-wk\\h/process bundle/VectorFlow Mouse Day 3 2018-02-09/2018-02-09 WT 10128/10128_39p5C_WT_sTx03A_20D_10000Hz_18MHz_0500mS_00_EYE", path "\\\\Vantage-n-wk\\h/process bundle/VectorFlow Mouse Day 3 2018-02-09/2018-02-09 WT 10128/10128_40p0C_WT_sTx03A_20D_10000Hz_18MHz_0500mS_00_EYE", path "\\\\Vantage-n-wk\\h/process bundle/VectorFlow Mouse Day 3 2018-02-09/2018-02-09 WT 10128/10128_40p0C_WT_sTx03A_20D_10000Hz_18MHz_0500mS_01_EYE", path "\\\\Vantage-n-wk\\h/process bundle/VectorFlow Mouse Day 3 2018-02-09/2018-02-09 WT 10128/10128_40p5C_WT_sTx03A_20D_10000Hz_18MHz_0500mS_00_EYE", path "\\\\Vantage-n-wk\\h/process bundle/VectorFlow Mouse Day 3 2018-02-09/2018-02-09 WT 10130/10130_35p0C_WT_sTx03A_20D_10000Hz_18MHz_0500mS_00_EYE", path "\\\\Vantage-n-wk\\h/process bundle/VectorFlow Mouse Day 3 2018-02-09/2018-02-09 WT 10130/10130_35p5C_WT_sTx03A_20D_10000Hz_25MHz_0500mS_00_EYE", path "\\\\Vantage-n-wk\\h/process bundle/VectorFlow Mouse Day 3 2018-02-09/2018-02-09 WT 10130/10130_36p0C_WT_sTx03A_20D_10000Hz_21MHz_0500mS_00_EYE", path "\\\\Vantage-n-wk\\h/process bundle/VectorFlow Mouse Day 3 2018-02-09/2018-02-09 WT 10130/10130_36p5C_WT_sTx03A_20D_10000Hz_18MHz_0500mS_00_EYE", path "\\\\Vantage-n-wk\\h/process bundle/VectorFlow Mouse Day 3 2018-02-09/2018-02-09 WT 10130/10130_36p5C_WT_sTx03A_20D_10000Hz_18MHz_0500mS_01_EYE", path "\\\\Vantage-n-wk\\h/process bundle/VectorFlow Mouse Day 3 2018-02-09/2018-02-09 WT 10130/10130_37p0C_WT_sTx03A_20D_10000Hz_18MHz_0500mS_00_EYE", path "\\\\Vantage-n-wk\\h/process bundle/VectorFlow Mouse Day 3 2018-02-09/2018-02-09 WT 10130/10130_37p5C_WT_sTx03A_20D_10000Hz_18MHz_0500mS_00_EYE", path "\\\\Vantage-n-wk\\h/process bundle/VectorFlow Mouse Day 3 2018-02-09/2018-02-09 WT 10130/10130_38p0C_WT_sTx03A_20D_10000Hz_18MHz_0500mS_00_EYE", path "\\\\Vantage-n-wk\\h/process bundle/VectorFlow Mouse Day 3 2018-02-09/2018-02-09 WT 10130/10130_39p0C_WT_sTx03A_20D_10000Hz_18MHz_0500mS_00_EYE", path "\\\\Vantage-n-wk\\h/process bundle/VectorFlow Mouse Day 3 2018-02-09/2018-02-09 WT 10130/10130_39p0C_WT_sTx03A_20D_10000Hz_18MHz_0500mS_01_EYE", path "\\\\Vantage-n-wk\\h/process bundle/VectorFlow Mouse Day 3 2018-02-09/2018-02-09 WT 10130/10130_40p0C_WT_sTx03A_20D_10000Hz_18MHz_0500mS_00_EYE", path "\\\\Vantage-n-wk\\h/process bundle/VectorFlow Mouse Day 3 2018-02-09/2018-02-09 WT 10130/10130_40p0C_WT_sTx03A_20D_10000Hz_18MHz_0500mS_01_EYE", path "\\\\Vantage-n-wk\\h/process bundle/VectorFlow Mouse Day 3 2018-02-09/2018-02-09 WT 10130/10130_41p0C_WT_sTx03A_20D_10000Hz_18MHz_0500mS_00_EYE", path "\\\\Vantage-n-wk\\h/process bundle/VectorFlow Mouse Day 3 2018-02-09/2018-02-09 WT 10132/10132_37p5C_WT_sTx03A_20D_10000Hz_18MHz_0500mS_00_EYE", path "\\\\Vantage-n-wk\\h/process bundle/VectorFlow Mouse Day 3 2018-02-09/2018-02-09 WT 10132/10132_38p0C_WT_sTx03A_20D_10000Hz_18MHz_0500mS_00_EYE", path "\\\\Vantage-n-wk\\h/process bundle/VectorFlow Mouse Day 3 2018-02-09/2018-02-09 WT 10132/10132_38p0C_WT_sTx03A_20D_10000Hz_18MHz_0500mS_01_EYE", path "\\\\Vantage-n-wk\\h/process bundle/VectorFlow Mouse Day 3 2018-02-09/2018-02-09 WT 10132/10132_38p0C_WT_sTx03A_20D_10000Hz_18MHz_0500mS_02_EYE", path "\\\\Vantage-n-wk\\h/process bundle/VectorFlow Mouse Day 3 2018-02-09/2018-02-09 WT 10132/10132_38p0C_WT_sTx03A_20D_10000Hz_18MHz_0500mS_03_EYE", path "\\\\Vantage-n-wk\\h/process bundle/VectorFlow Mouse Day 3 2018-02-09/2018-02-09 WT 10132/10132_38p0C_WT_sTx03A_20D_10000Hz_18MHz_0500mS_04_EYE", path "\\\\Vantage-n-wk\\h/process bundle/VectorFlow Mouse Day 3 2018-02-09/2018-02-09 WT 10132/10132_38p5C_WT_sTx03A_20D_10000Hz_18MHz_0500mS_00_EYE", path "\\\\Vantage-n-wk\\h/process bundle/VectorFlow Mouse Day 3 2018-02-09/2018-02-09 WT 10132/10132_39p0C_WT_sTx03A_20D_10000Hz_18MHz_0500mS_00_EYE", path "\\\\Vantage-n-wk\\h/process bundle/VectorFlow Mouse Day 3 2018-02-09/2018-02-09 WT 10132/10132_39p0C_WT_sTx03A_20D_10000Hz_18MHz_0500mS_01_EYE", path "\\\\Vantage-n-wk\\h/process bundle/VectorFlow Mouse Day 3 2018-02-09/2018-02-09 WT 10132/10132_39p5C_WT_sTx03A_20D_10000Hz_18MHz_0500mS_00_EYE", path "\\\\Vantage-n-wk\\h/process bundle/VectorFlow Mouse Day 3 2018-02-09/2018-02-09 WT 10132/10132_40p0C_WT_sTx03A_20D_10000Hz_18MHz_0500mS_00_EYE", path "\\\\Vantage-n-wk\\h/process bundle/VectorFlow Mouse Day 3 2018-02-09/2018-02-09 WT 10132/10132_40p5C_WT_sTx03A_20D_10000Hz_18MHz_0500mS_00_EYE", path "\\\\Vantage-n-wk\\h/process bundle/VectorFlow Mouse Day 3 2018-02-09/2018-02-09 WT 10132/10132_41p0C_WT_sTx03A_20D_10000Hz_18MHz_0500mS_00_EYE", path "\\\\Vantage-n-wk\\h/process bundle/VectorFlow Mouse Day 3 2018-02-09/2018-02-09 WT 10132/10132_41p0C_WT_sTx03A_20D_10000Hz_18MHz_0500mS_01_EYE"]
  in  "Choose Top level folder":path=path "\\\\Vantage-n-wk\\h/process bundle"
  in  "Batch Spectorgram":bool
  in  "Save Tiled":bool
  in  "Skip X":i32=5
  in  "Skip Y":i32=5
  in  "Use VPI crop?":bool
  in  "Split files?":bool=TRUE
  in  "Only Real of Sum?":bool
  in  "Choose Crop File?":bool
  in  "Crop file":path
  in  "Type of Read 2":T5(ring)=enum."Save IQSum"
  in  "Lock scale":bool
  in  "Only Buff 3?":bool
  in  "read?":bool=TRUE
  in  "stop":bool
  # "old search extension."
  # "*_HeaderInfoIQSum*"
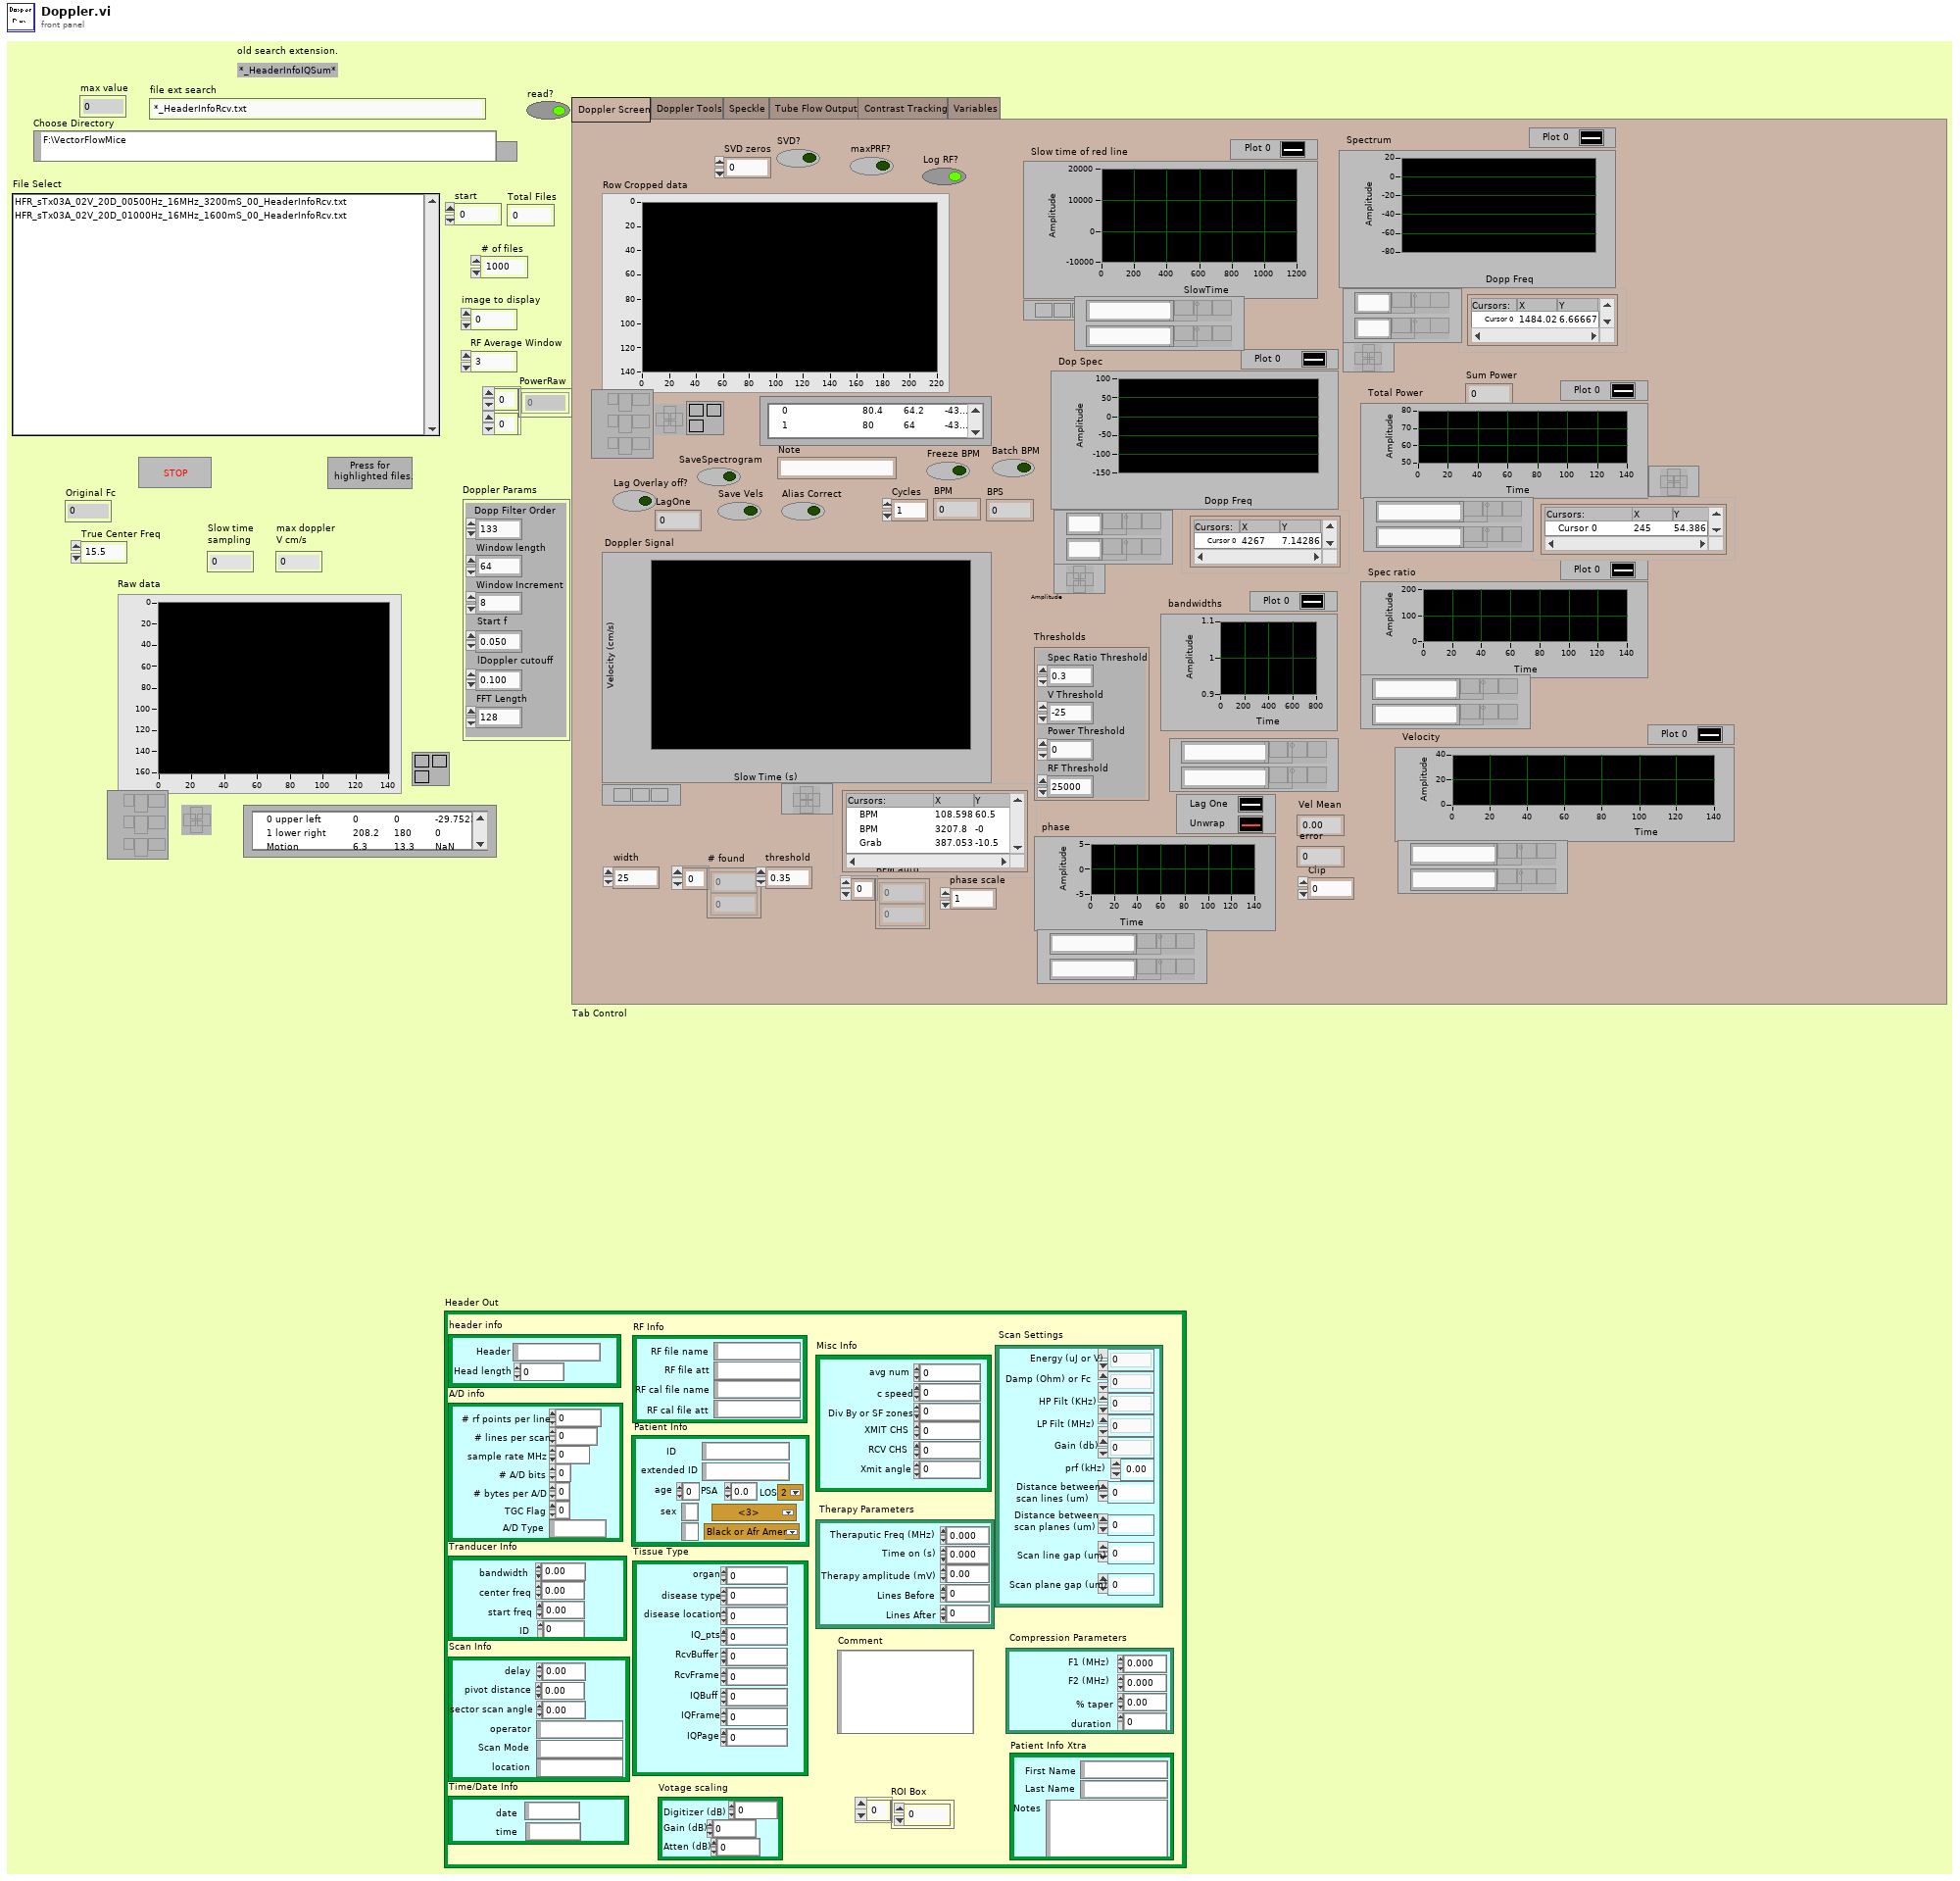
[diagram p1: front panel]
types:
  T1 = typedef "Header.ctl" = cluster{"header info":cluster{"Header":string, "Head length":i16}, "A/D info":cluster{"# rf points per line":u16, "# lines per scan":u16, "sample rate MHz":u16, "# A/D bits":i16, "# bytes per A/D":u16, "TGC Flag":u16, "A/D Type":string}, "Tranducer Info":cluster{"bandwidth":sgl, "center freq":sgl, "start freq":sgl, "ID":i32}, "Scan Info":cluster{"delay":sgl, "pivot distance":sgl, "sector scan angle":sgl, "operator":string, "Scan Mode":string, "location":string}, "Time/Date Info":cluster{"date":string, "time":string}, "RF Info":cluster{"RF file name":string, "RF file att":string, "RF cal file name":string, "RF cal file att":string}, "Patient Info":cluster{"ID":string, "extended ID":string, "age":u16, "sex":string, "previously\nscanned":string, "PSA":sgl, "LOS":u8, "Ethnicty 2":u8, "Race":u8}, "Tissue Type":cluster{"organ":i16, "disease type":i16, "disease location":i16, "IQ_pts":u16, "RcvBuffer":u8, "RcvFrame":u16, "IQBuff":u8, "IQFrame":u16, "IQPage":u8}, "Votage scaling":cluster{"Digitizer (dB)":sgl, "Gain (dB)":sgl, "Atten (dB)":sgl}, "Comment":string, "Misc Info":cluster{"avg num":u16, "c speed":i16, "Div By or SF zones":i16, "XMIT CHS":u8, "RCV CHS":u8, "Xmit angle":sgl}, "Therapy Parameters":cluster{"Theraputic Freq (MHz)":sgl, "Time on (s)":sgl, "Therapy amplitude (mV)":sgl, "Lines Before":u16, "Lines After":u16}, "Scan Settings":cluster{"Energy (uJ or V)":u8, "Damp (Ohm) or Fc":u8, "HP Filt (KHz)":u8, "LP Filt (MHz)":u8, "Gain (db)":u8, "prf (kHz)":sgl, "Distance between\nscan lines (um)":u16, "Distance between\nscan planes (um)":u16, "Scan line gap (um)":sgl, "Scan plane gap (um)":sgl}, "Compression Parameters":cluster{"F1 (MHz)":sgl, "F2 (MHz)":sgl, "% taper":sgl, "duration":sgl}, "Patient Info Xtra":cluster{"First Name":string, "Last Name":string, "Notes":string}, "ROI Box":u16[]}
  T2 = typedef "DopplerParams.ctl" = cluster{"Dopp Filter Order":i32, "Window length":i32, "Window Increment":i32, "Start f":dbl, "lDoppler cutouff":dbl, "FFT Length":i32, "SlowTime (Hz)":dbl}
  T3 = enum32{"Doppler Screen", "Doppler Tools", "Speckle", "Tube Flow Output", "Contrast Tracking", "Variables"}
  T4 = typedef "DopThresholds.ctl" = cluster{"Spec Ratio Threshold":dbl, "V Threshold":dbl, "Power Threshold":dbl, "RF Threshold":dbl}
  T5 = enum16{"None", "Raw RF + time stamp", "Save IQAll", "Save IQSum", "Save IQSumReal", "Save Img", "Time Stamps", "unused"}
  T6 = cluster{"subarray":i8[][][], "Slow Time Pt":i32, "Line#":i32}
  T7 = cluster{"Line start":dbl, "# of lines":dbl, "RF start":dbl, "# pts":dbl}
  T8 = cluster{"Line start":dbl, dbl, "RF start":dbl, dbl}
  T9 = cluster{cluster{dbl, u16}, dbl, dbl, "delay":sgl, "delay":sgl, dbl, dbl}
  T10 = cluster{"Y Scale Mult":dbl, "Y Scale offset":dbl, "X Scale Mult":dbl, "Dop F offset":dbl, "Dop interval":dbl}
  T11 = typedef "imagedata.ctl" = cluster{"image type":i32, "image depth":i32, "image":u8[], "mask":u8[], "colors":u32[], "Rectangle":cluster{"left":i16, "top":i16, "right":i16, "bottom":i16}}
  T12 = enum16{"User-specified Font", "Application Font", "System Font", "Dialog Font"}
  T13 = cluster{"Font Name:":string, "Size":i16, "Strikeout?":bool, "Italic?":bool, "Underline?":bool, "Outline?":bool, "Shadow?":bool, "Bold?":bool}
  T14 = typedef "LVPointDoubleTypeDef.ctl" = cluster{"Cursor X":dbl, "Cursor Y":dbl}
  T15 = cluster{i8[][][], "max queue size (-1, unlimited)":i32, i32}
  T16 = enum16{"big-endian, network order", "native, host order", "little-endian"}
  T17 = cluster{"max f":sgl, "max freq (dB)":sgl, "center freq":sgl, "lower band freq":sgl, "upper band freq":sgl, "bandwidth":sgl, "% BW":dbl}
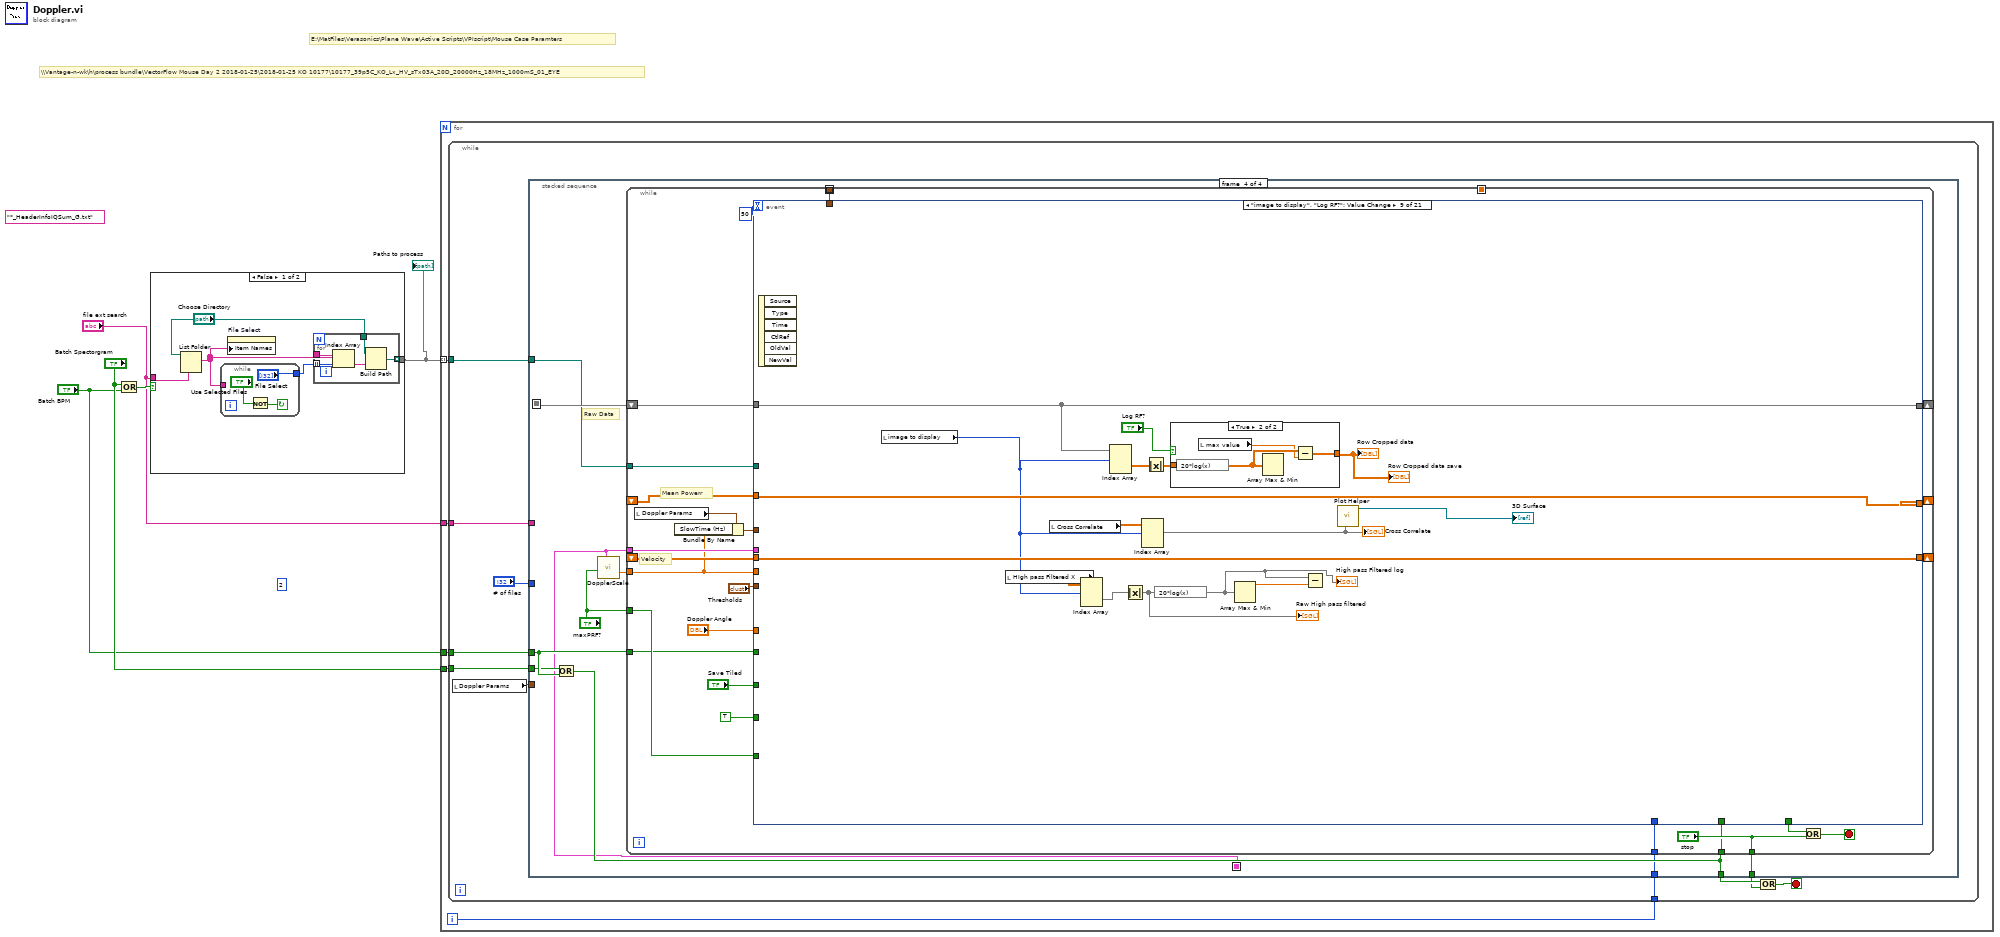
[diagram p0: block diagram]
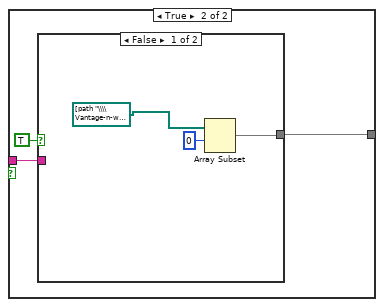
[diagram p2: hidden frame]
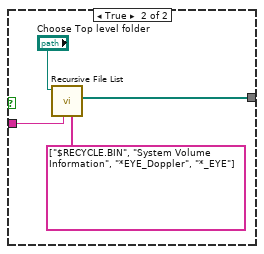
[diagram p3: hidden frame]
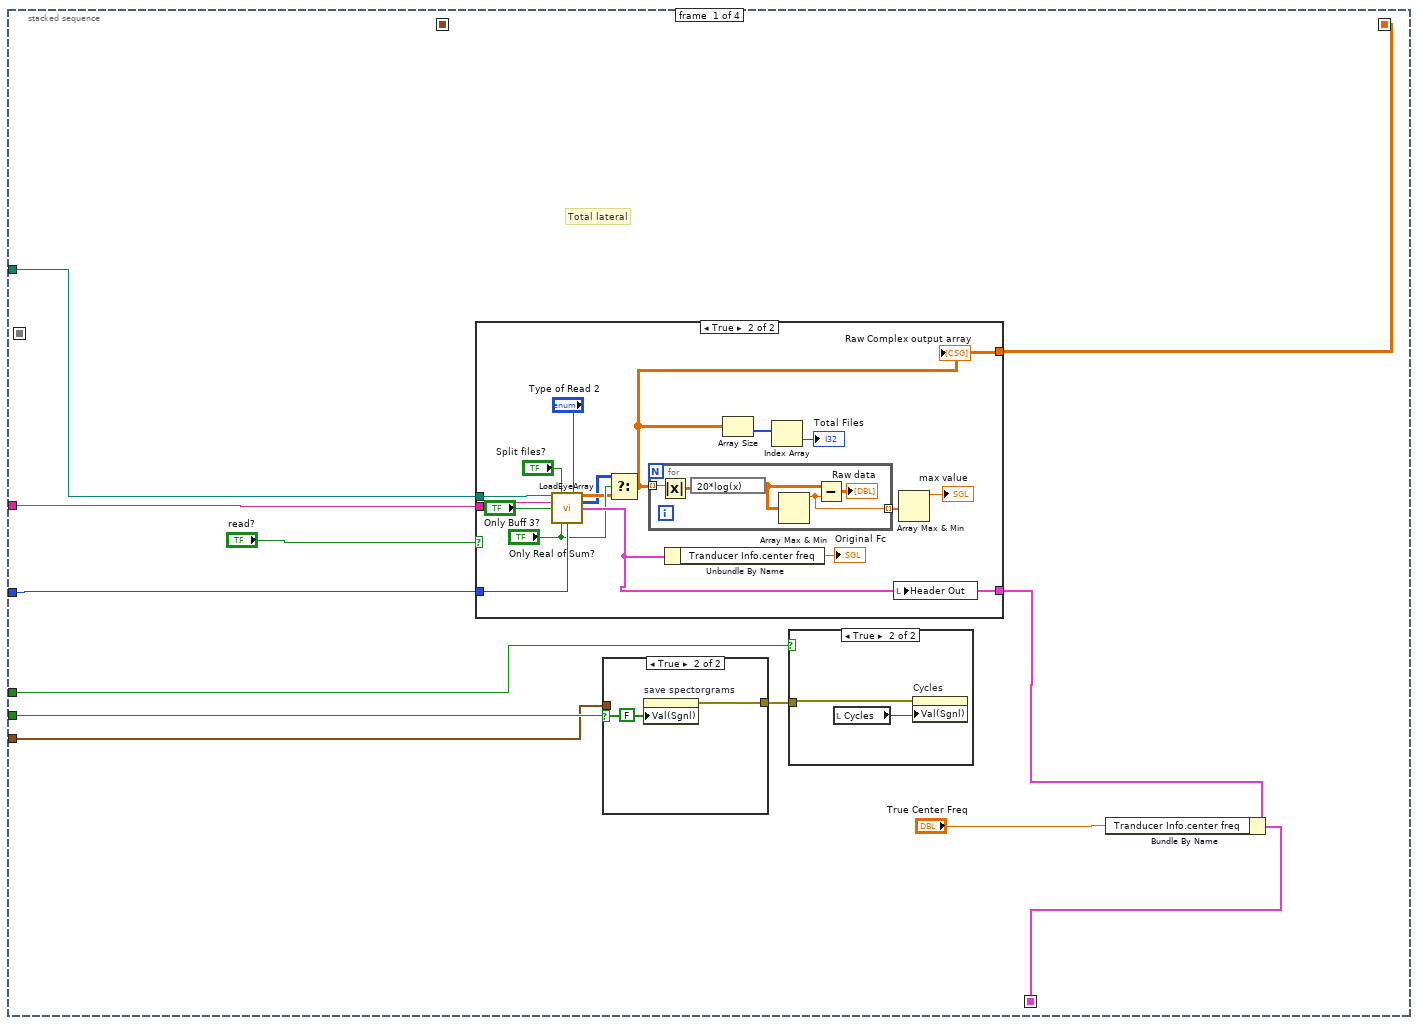
[diagram p4: hidden frame]
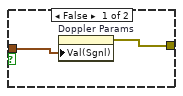
[diagram p6: hidden frame]
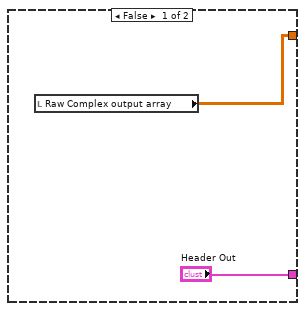
[diagram p7: hidden frame]
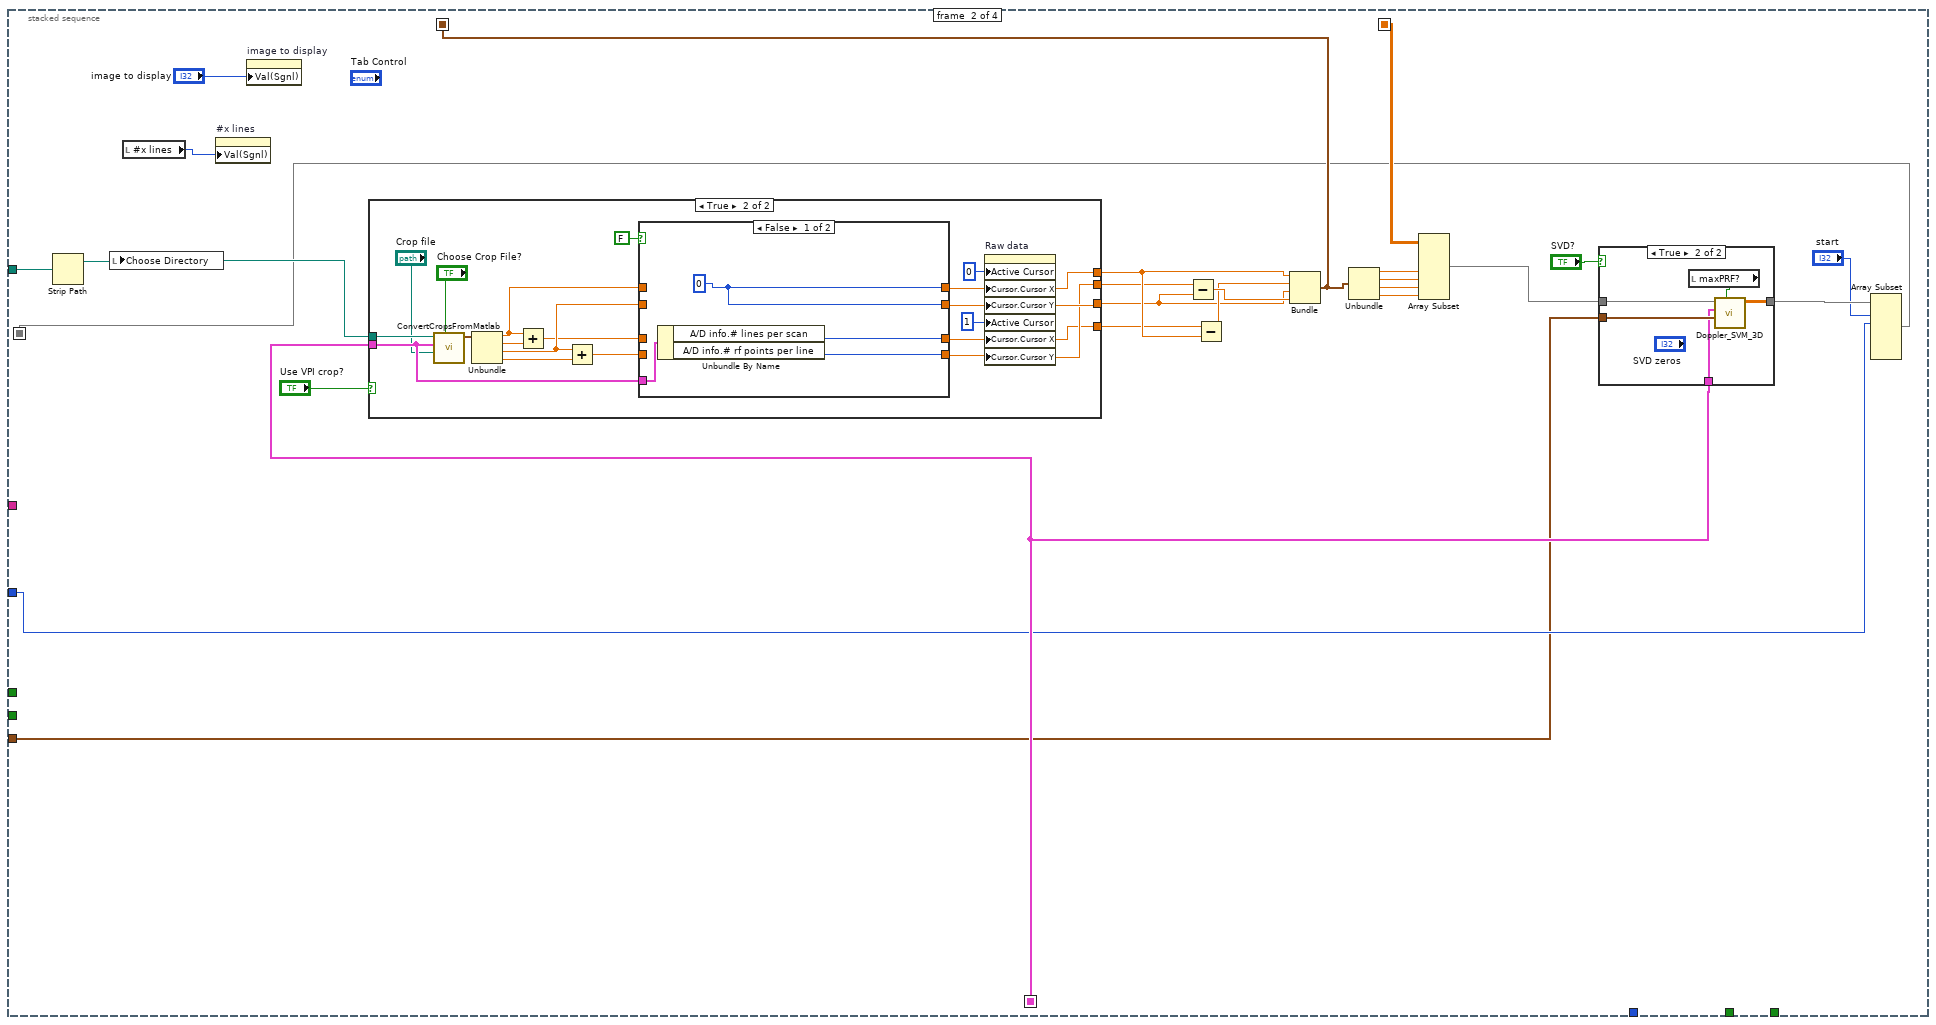
[diagram p8: hidden frame]
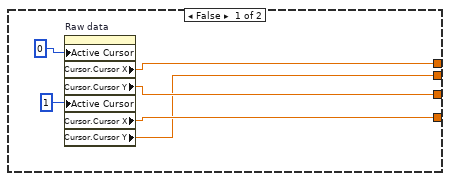
[diagram p10: hidden frame]
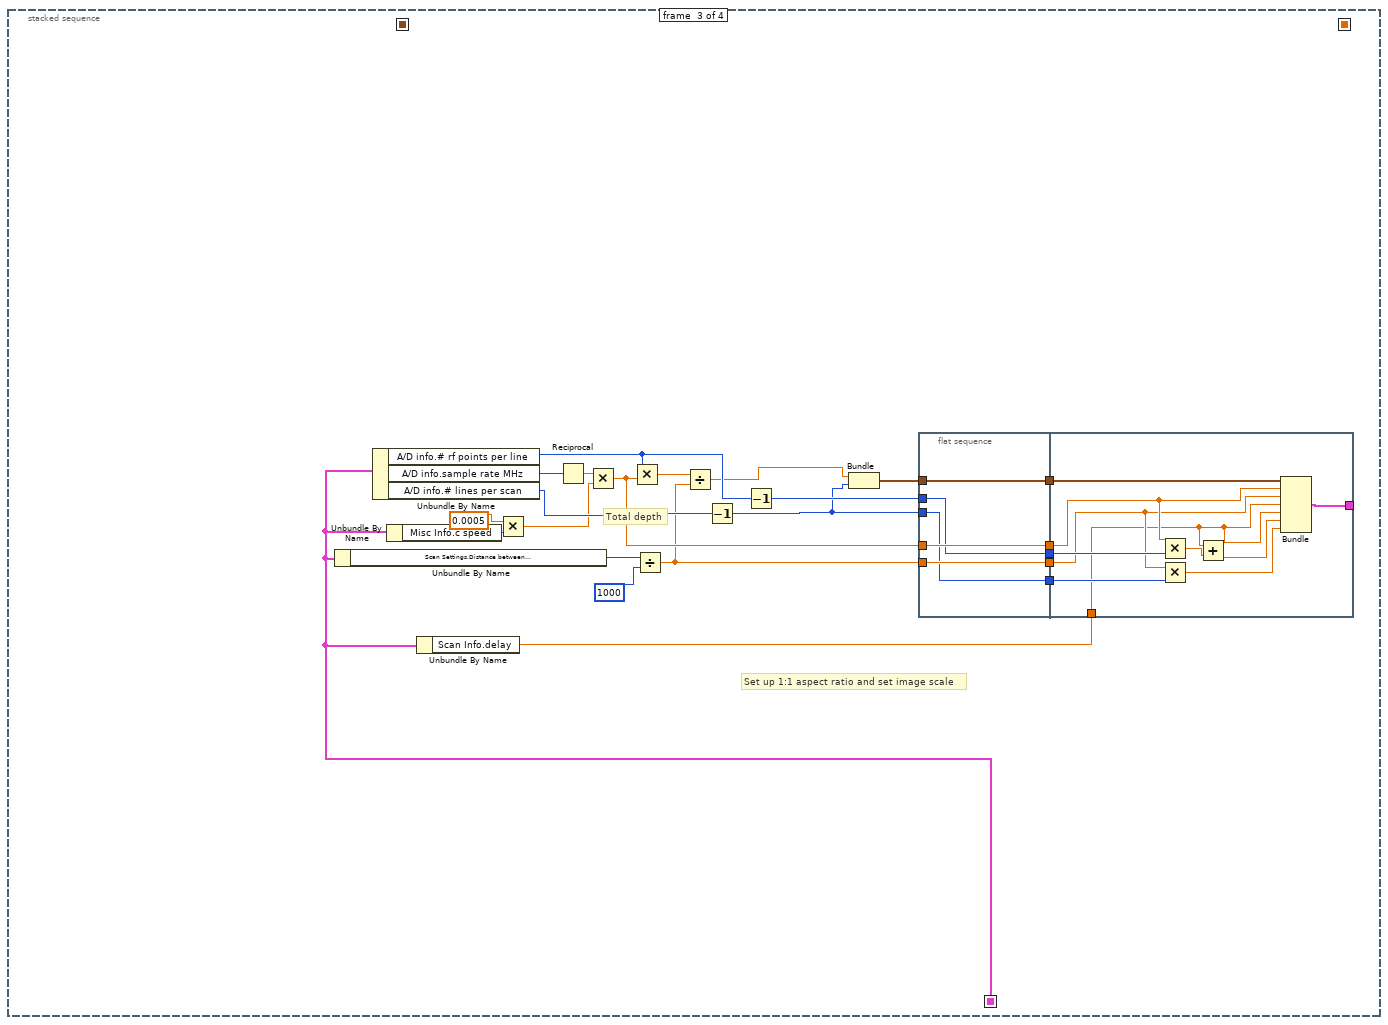
[diagram p12: hidden frame]
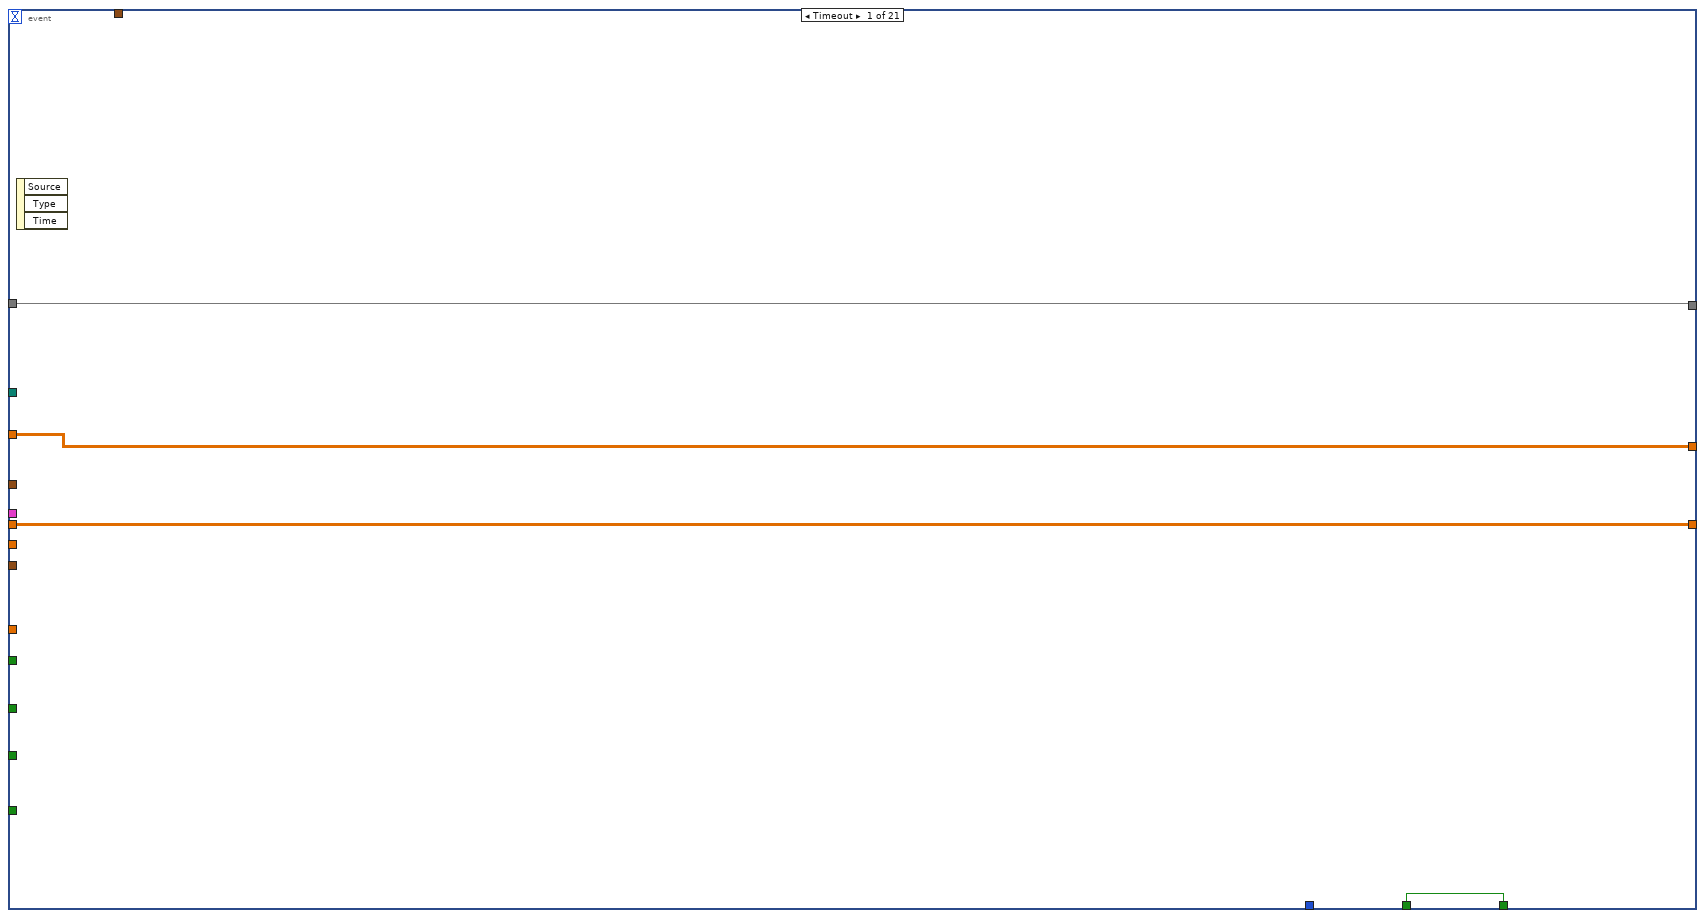
[diagram p13: hidden frame]
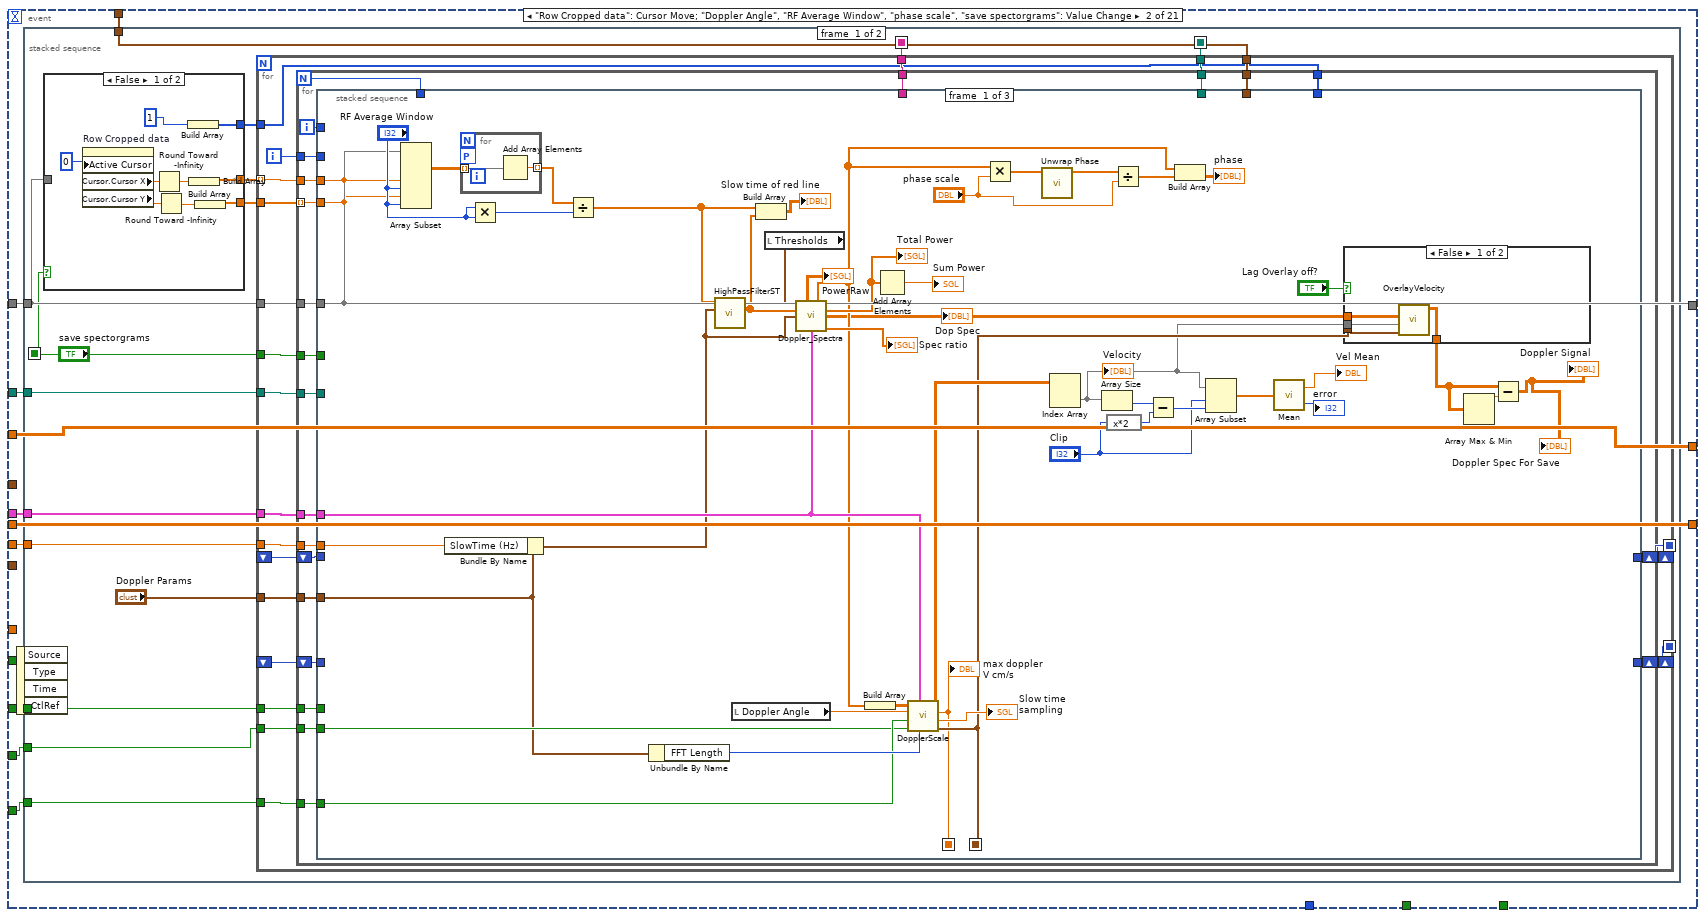
[diagram p14: hidden frame]
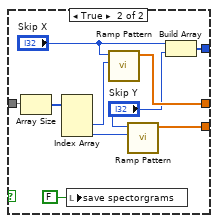
[diagram p15: hidden frame]
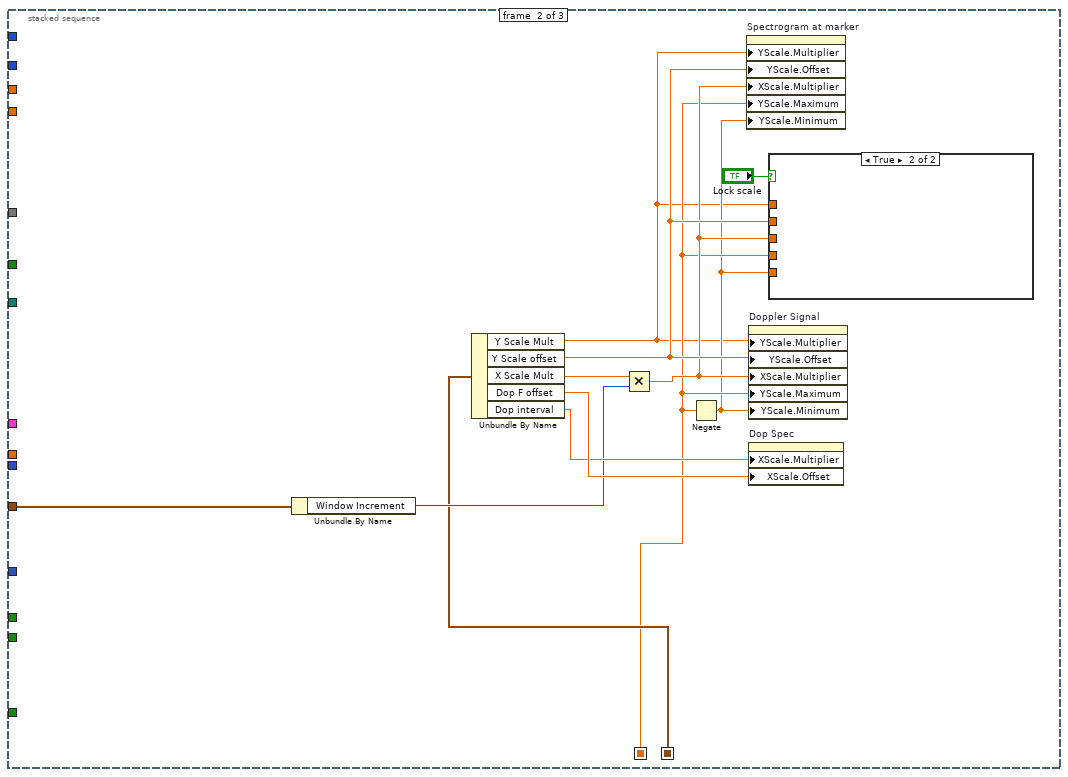
[diagram p17: hidden frame]
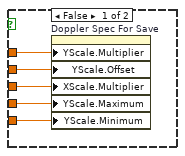
[diagram p18: hidden frame]
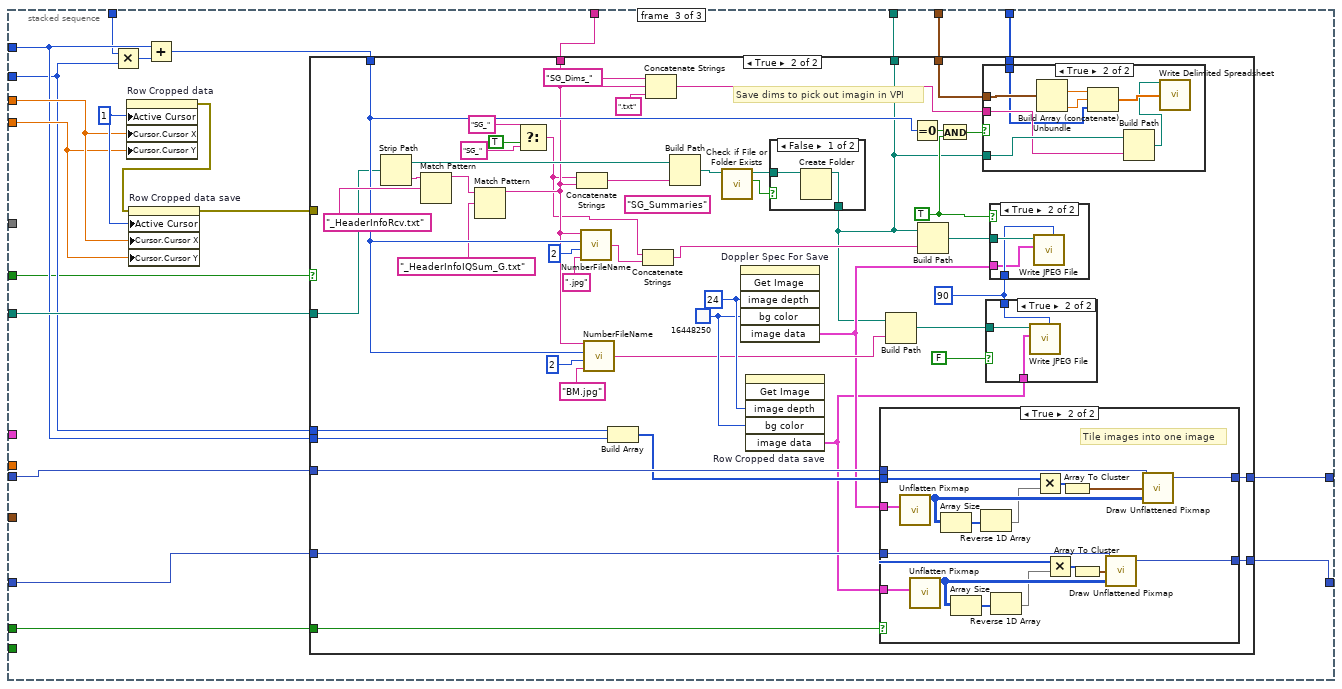
[diagram p19: hidden frame]
diagram:
  (unwired) u32 2 ("Active Cursor")
  (unwired) "*_HeaderInfoIQSum_G.txt" ("String")
  # "E:\\MatFiles\\Verasonics\\Plane Wave\\Active Scripts\\VPIscript\\Mouse Case Paramters"
  # "\\\\Vantage-n-wk\\h\\process bundle\\VectorFlow Mouse Day 2 2018-01-25\\2018-01-25 KO 10177\\10177_39p5C_KO_Lx_HV_sTx03A_20D_20000Hz_18MHz_1000mS_01_EYE"
  n1 = Or(x="Batch Spectorgram", y="Batch BPM") -> (x .or. y?=w5:bool)
  n2 = case shown="False" w5 {
    tunnel: [w7 w21] -> w2
    tunnel: "file ext search" -> [w6 w19]
    frame False {
      n3 = List Folder(path="Choose Directory", pattern=w6) -> (filenames=w9:string[])  [unwired: 1 in, 4 out]
      n4 = while {
        tunnel: ["File Select"] -> w10
        tunnel: w9 -> [_]
        stop <- w18 continue-if-true
        n5 = Not(x="Use Selected Files") -> (.not. x?=w18:bool)
      }
      n6 = property on="File Select" class="LstBox (strict)"("Item Names"=w9) -> ()  [unwired: 2 in, 2 out]
      n7 = for {
        tunnel: w10 -> [w14] mode=indexing
        tunnel: w9 -> [w15]
        tunnel: "Choose Directory" -> [w12]
        tunnel: [w11] -> w7 mode=indexing
        n8 = Index Array(array=w15, index=w14) -> (element=w13:string)
        n9 = Build Path(base path=w12, name or relative path=w13) -> (appended path=w11:path)
      }
    }
    frame True {
      n10 = case shown="False" TRUE {
        tunnel: [w22 w26] -> w21
        tunnel: w19 -> [_ w25]
        frame False {
          n11 = Array Subset(array=path[] [path "\\\\Vantage-n-wk\\h/process bundle/VectorFlow Mouse Day 1 2017-07-14/2017-07-14 9412_WT/sTx3_37_0C_9412_WT_Lx_HV_03A_10D_10000Hz_16MHz_1000mS_00_EYE", path "\\\\Vantage-n-wk\\h/process bundle/VectorFlow Mouse Day 1 2017-07-14/2017-07-14 9412_WT/sTx3_38_0C_9412_WT_Lx_HV_03A_10D_10000Hz_16MHz_1000mS_00_EYE", path "\\\\Vantage-n-wk\\h/process bundle/VectorFlow Mouse Day 1 2017-07-14/2017-07-14 9412_WT/sTx3_39_0C_9412_WT_Lx_HV_03A_10D_10000Hz_16MHz_1000mS_00_EYE", path "\\\\Vantage-n-wk\\h/process bundle/VectorFlow Mouse Day 1 2017-07-14/2017-07-14 9412_WT/sTx3_40_0C_9412_WT_Lx_HV_03A_10D_10000Hz_16MHz_1000mS_00_EYE", path "\\\\Vantage-n-wk\\h/process bundle/VectorFlow Mouse Day 1 2017-07-14/2017-07-14 9412_WT/sTx3_40_5C_9412_WT_Lx_HV_03A_10D_10000Hz_16MHz_1000mS_00_EYE", path "\\\\Vantage-n-wk\\h/process bundle/VectorFlow Mouse Day 1 2017-07-14/2017-07-14 9412_WT/sTx3_41_0C_9412_WT_Lx_HV_03A_10D_10000Hz_16MHz_1000mS_00_EYE", path "\\\\Vantage-n-wk\\h/process bundle/VectorFlow Mouse Day 1 2017-07-14/2017-07-14 9412_WT/sTx6_37_0C_9412_WT_Lx_HV_06A_10D_05000Hz_16MHz_1040mS_00_EYE", path "\\\\Vantage-n-wk\\h/process bundle/VectorFlow Mouse Day 1 2017-07-14/2017-07-14 9412_WT/sTx7_36_5C_9412_WT_Lx_HV_07A_10D_04286Hz_16MHz_0933mS_00_EYE", path "\\\\Vantage-n-wk\\h/process bundle/VectorFlow Mouse Day 1 2017-07-14/2017-07-14 9412_WT/sTx7_37_0C_9412_WT_Lx_HV_07A_10D_04286Hz_16MHz_0933mS_00_EYE", path "\\\\Vantage-n-wk\\h/process bundle/VectorFlow Mouse Day 1 2017-07-14/2017-07-14 9412_WT/sTx7_41_0C_9412_WT_Lx_HV_07A_10D_04286Hz_16MHz_0933mS_00_EYE", path "\\\\Vantage-n-wk\\h/process bundle/VectorFlow Mouse Day 1 2017-07-14/2017-07-14 9415_KO/sTX3_37C_9415_KO_Lx_03A_10D_10000Hz_16MHz_1000mS_00_EYE", path "\\\\Vantage-n-wk\\h/process bundle/VectorFlow Mouse Day 1 2017-07-14/2017-07-14 9415_KO/sTX3_37C_9415_KO_Lx_HV_03A_10D_10000Hz_16MHz_1000mS_00_EYE", path "\\\\Vantage-n-wk\\h/process bundle/VectorFlow Mouse Day 1 2017-07-14/2017-07-14 9415_KO/sTX3_37C_9415_KO_Lx_HV_2_03A_10D_10000Hz_16MHz_0520mS_00_EYE", path "\\\\Vantage-n-wk\\h/process bundle/VectorFlow Mouse Day 1 2017-07-14/2017-07-14 9415_KO/sTX3_37C_9415_KO_Lx_HV_2_03A_10D_10000Hz_16MHz_1000mS_00_EYE", path "\\\\Vantage-n-wk\\h/process bundle/VectorFlow Mouse Day 1 2017-07-14/2017-07-14 9415_KO/sTx3_41_7C_9415_KO_Lx_HV_03A_10D_10000Hz_16MHz_1000mS_00_EYE", path "\\\\Vantage-n-wk\\h/process bundle/VectorFlow Mouse Day 1 2017-07-14/2017-07-14 9415_KO/sTX7_37C_9415_KO_Lx_HV_07A_10D_04286Hz_16MHz_0933mS_00_EYE", path "\\\\Vantage-n-wk\\h/process bundle/VectorFlow Mouse Day 1 2017-07-14/2017-07-14 9415_KO/sTx7_37C_9415_KO_Lx_HV_2_07A_10D_04286Hz_16MHz_0933mS_00_EYE", path "\\\\Vantage-n-wk\\h/process bundle/VectorFlow Mouse Day 1 2017-07-14/2017-07-14 9415_KO/sTx7_39_5C_9415_KO_Lx_HV_07A_10D_04286Hz_16MHz_0933mS_00_EYE", path "\\\\Vantage-n-wk\\h/process bundle/VectorFlow Mouse Day 1 2017-07-14/2017-07-14 9415_KO/sTx7_40_5C_9415_KO_Lx_HV_07A_10D_04286Hz_16MHz_0933mS_00_EYE", path "\\\\Vantage-n-wk\\h/process bundle/VectorFlow Mouse Day 1 2017-07-14/2017-07-14 9415_KO/sTx7_41_2C_9415_KO_Lx_HV_07A_10D_04286Hz_16MHz_0933mS_00_EYE", path "\\\\Vantage-n-wk\\h/process bundle/VectorFlow Mouse Day 1 2017-07-14/2017-07-14 9415_KO/sTx7_41_7C_9415_KO_Lx_HV_07A_10D_04286Hz_16MHz_0933mS_00_EYE", path "\\\\Vantage-n-wk\\h/process bundle/VectorFlow Mouse Day 1 2017-07-14/2017-07-14 9415_KO/sTx7_42_0C_9415_KO_Lx_HV_07A_10D_04286Hz_16MHz_0933mS_00_EYE", path "\\\\Vantage-n-wk\\h/process bundle/VectorFlow Mouse Day 1 2017-07-14/2017-07-14 9416_KO/sTx3_37_3C_9416_KO_Lx_HV_03A_10D_10000Hz_16MHz_1000mS_00_EYE", path "\\\\Vantage-n-wk\\h/process bundle/VectorFlow Mouse Day 1 2017-07-14/2017-07-14 9416_KO/sTx3_37_6C_9416_KO_Lx_HV_03A_10D_10000Hz_16MHz_1000mS_00_EYE", path "\\\\Vantage-n-wk\\h/process bundle/VectorFlow Mouse Day 1 2017-07-14/2017-07-14 9416_KO/sTx3_38_1C_9416_KO_Lx_HV_03A_10D_10000Hz_16MHz_1000mS_00_EYE", path "\\\\Vantage-n-wk\\h/process bundle/VectorFlow Mouse Day 1 2017-07-14/2017-07-14 9416_KO/sTx3_39_0C_9416_KO_Lx_HV_03A_10D_10000Hz_16MHz_1000mS_00_EYE", path "\\\\Vantage-n-wk\\h/process bundle/VectorFlow Mouse Day 1 2017-07-14/2017-07-14 9416_KO/sTx3_40_0C_9416_KO_Lx_HV_03A_10D_10000Hz_16MHz_1000mS_00_EYE", path "\\\\Vantage-n-wk\\h/process bundle/VectorFlow Mouse Day 1 2017-07-14/2017-07-14 9416_KO/sTx3_40_5C_9416_KO_Lx_HV_03A_10D_10000Hz_16MHz_1000mS_00_EYE", path "\\\\Vantage-n-wk\\h/process bundle/VectorFlow Mouse Day 1 2017-07-14/2017-07-14 9416_KO/sTx3_41_0C_9416_KO_Lx_HV_03A_10D_10000Hz_16MHz_1000mS_00_EYE", path "\\\\Vantage-n-wk\\h/process bundle/VectorFlow Mouse Day 1 2017-07-14/2017-07-14 9416_KO/sTx3_41_3C_9416_KO_Lx_HV_03A_10D_10000Hz_16MHz_1000mS_00_EYE", path "\\\\Vantage-n-wk\\h/process bundle/VectorFlow Mouse Day 1 2017-07-14/2017-07-14 9416_KO/sTx7_36_6C_9416_KO_Lx_HV_07A_10D_04286Hz_16MHz_0933mS_00_EYE", path "\\\\Vantage-n-wk\\h/process bundle/VectorFlow Mouse Day 1 2017-07-14/2017-07-14 9416_KO/sTx7_37_5C_9416_KO_Lx_HV_07A_10D_04286Hz_16MHz_0933mS_00_EYE", path "\\\\Vantage-n-wk\\h/process bundle/VectorFlow Mouse Day 1 2017-07-14/2017-07-14 9416_KO/sTx7_38_2C_9416_KO_Lx_HV_07A_10D_04286Hz_16MHz_0933mS_00_EYE", path "\\\\Vantage-n-wk\\h/process bundle/VectorFlow Mouse Day 1 2017-07-14/2017-07-14 9416_KO/sTx7_41_0C_9416_KO_Lx_HV_07A_10D_04286Hz_16MHz_0933mS_00_EYE", path "\\\\Vantage-n-wk\\h/process bundle/VectorFlow Mouse Day 2 2018-01-25/2018-01-25 KO 10129/10129_35p5C_KO_Lx_HV_sTx03A_20D_10000Hz_18MHz_1000mS_00_EYE", path "\\\\Vantage-n-wk\\h/process bundle/VectorFlow Mouse Day 2 2018-01-25/2018-01-25 KO 10129/10129_35p7C_KO_Lx_HV_sTx03A_20D_10000Hz_18MHz_1000mS_00_EYE", path "\\\\Vantage-n-wk\\h/process bundle/VectorFlow Mouse Day 2 2018-01-25/2018-01-25 KO 10129/10129_36p5C_KO_Lx_HV_sTx03A_20D_10000Hz_18MHz_1000mS_00_EYE", path "\\\\Vantage-n-wk\\h/process bundle/VectorFlow Mouse Day 2 2018-01-25/2018-01-25 KO 10129/10129_37p0C_KO_Lx_HV_sTx03A_20D_10000Hz_18MHz_1000mS_00_EYE", path "\\\\Vantage-n-wk\\h/process bundle/VectorFlow Mouse Day 2 2018-01-25/2018-01-25 KO 10129/10129_37p0C_KO_Lx_HV_sTx03A_20D_10000Hz_18MHz_1000mS_01_EYE", path "\\\\Vantage-n-wk\\h/process bundle/VectorFlow Mouse Day 2 2018-01-25/2018-01-25 KO 10129/10129_37p5C_KO_Lx_HV_sTx03A_20D_10000Hz_18MHz_1000mS_01_EYE", path "\\\\Vantage-n-wk\\h/process bundle/VectorFlow Mouse Day 2 2018-01-25/2018-01-25 KO 10129/10129_38p0C_KO_Lx_HV_sTx03A_20D_10000Hz_18MHz_1000mS_00_EYE", path "\\\\Vantage-n-wk\\h/process bundle/VectorFlow Mouse Day 2 2018-01-25/2018-01-25 KO 10129/10129_38p5C_KO_Lx_HV_sTx03A_20D_10000Hz_18MHz_1000mS_00_EYE", path "\\\\Vantage-n-wk\\h/process bundle/VectorFlow Mouse Day 2 2018-01-25/2018-01-25 KO 10129/10129_38p5C_KO_Lx_HV_sTx03A_20D_10000Hz_18MHz_1000mS_01_EYE", path "\\\\Vantage-n-wk\\h/process bundle/VectorFlow Mouse Day 2 2018-01-25/2018-01-25 KO 10129/10129_39p5C_KO_Lx_HV_sTx03A_20D_10000Hz_18MHz_1000mS_00_EYE", path "\\\\Vantage-n-wk\\h/process bundle/VectorFlow Mouse Day 2 2018-01-25/2018-01-25 KO 10129/10129_40p0C_KO_Lx_HV_sTx03A_20D_10000Hz_18MHz_1000mS_00_EYE", path "\\\\Vantage-n-wk\\h/process bundle/VectorFlow Mouse Day 2 2018-01-25/2018-01-25 KO 10129/10129_40p0C_KO_Lx_HV_sTx03A_20D_10000Hz_18MHz_1000mS_01_EYE", path "\\\\Vantage-n-wk\\h/process bundle/VectorFlow Mouse Day 2 2018-01-25/2018-01-25 KO 10129/10129_40p5C_KO_Lx_HV_sTx03A_20D_10000Hz_18MHz_1000mS_00_EYE", path "\\\\Vantage-n-wk\\h/process bundle/VectorFlow Mouse Day 2 2018-01-25/2018-01-25 KO 10129/10129_41p0C_KO_Lx_HV_sTx03A_20D_10000Hz_18MHz_1000mS_00_EYE", path "\\\\Vantage-n-wk\\h/process bundle/VectorFlow Mouse Day 2 2018-01-25/2018-01-25 KO 10129/10129_41p0C_KO_Lx_HV_sTx03A_20D_10000Hz_18MHz_1000mS_01_EYE", path "\\\\Vantage-n-wk\\h/process bundle/VectorFlow Mouse Day 2 2018-01-25/2018-01-25 KO 10176/10176_36p5C_KO_Lx_HV_sTx03A_20D_10000Hz_18MHz_1000mS_00_EYE", path "\\\\Vantage-n-wk\\h/process bundle/VectorFlow Mouse Day 2 2018-01-25/2018-01-25 KO 10176/10176_37C_KO_Lx_HV_sTx03A_20D_10000Hz_18MHz_1000mS_00_EYE", path "\\\\Vantage-n-wk\\h/process bundle/VectorFlow Mouse Day 2 2018-01-25/2018-01-25 KO 10176/10176_37C_KO_Lx_HV_sTx03A_20D_10000Hz_18MHz_1000mS_01_EYE", path "\\\\Vantage-n-wk\\h/process bundle/VectorFlow Mouse Day 2 2018-01-25/2018-01-25 KO 10176/10176_37C_KO_Lx_HV_sTx03A_20D_10000Hz_18MHz_1000mS_02_EYE", path "\\\\Vantage-n-wk\\h/process bundle/VectorFlow Mouse Day 2 2018-01-25/2018-01-25 KO 10176/10176_37C_KO_Lx_HV_sTx03A_20D_10000Hz_18MHz_1000mS_03_EYE", path "\\\\Vantage-n-wk\\h/process bundle/VectorFlow Mouse Day 2 2018-01-25/2018-01-25 KO 10176/10176_37C_KO_Lx_HV_sTx03A_20D_10000Hz_18MHz_1000mS_04_EYE", path "\\\\Vantage-n-wk\\h/process bundle/VectorFlow Mouse Day 2 2018-01-25/2018-01-25 KO 10176/10176_37p0C_KO_Lx_HV_sTx03A_20D_10000Hz_18MHz_1000mS_00_EYE", path "\\\\Vantage-n-wk\\h/process bundle/VectorFlow Mouse Day 2 2018-01-25/2018-01-25 KO 10176/10176_37p5C_KO_Lx_HV_sTx03A_20D_10000Hz_18MHz_1000mS_00_EYE", path "\\\\Vantage-n-wk\\h/process bundle/VectorFlow Mouse Day 2 2018-01-25/2018-01-25 KO 10176/10176_38C_KO_Lx_HV_sTx03A_20D_10000Hz_18MHz_1000mS_00_EYE", path "\\\\Vantage-n-wk\\h/process bundle/VectorFlow Mouse Day 2 2018-01-25/2018-01-25 KO 10176/10176_38p0C_KO_Lx_HV_sTx03A_20D_10000Hz_18MHz_1000mS_00_EYE", path "\\\\Vantage-n-wk\\h/process bundle/VectorFlow Mouse Day 2 2018-01-25/2018-01-25 KO 10176/10176_38p5C_KO_Lx_HV_sTx03A_20D_10000Hz_18MHz_1000mS_00_EYE", path "\\\\Vantage-n-wk\\h/process bundle/VectorFlow Mouse Day 2 2018-01-25/2018-01-25 KO 10176/10176_39C_KO_Lx_HV_sTx03A_20D_10000Hz_18MHz_1000mS_00_EYE", path "\\\\Vantage-n-wk\\h/process bundle/VectorFlow Mouse Day 2 2018-01-25/2018-01-25 KO 10176/10176_39C_KO_Lx_HV_sTx03A_20D_10000Hz_18MHz_1000mS_01_EYE", path "\\\\Vantage-n-wk\\h/process bundle/VectorFlow Mouse Day 2 2018-01-25/2018-01-25 KO 10176/10176_39C_KO_Lx_HV_sTx03A_20D_10000Hz_18MHz_1000mS_02_EYE", path "\\\\Vantage-n-wk\\h/process bundle/VectorFlow Mouse Day 2 2018-01-25/2018-01-25 KO 10176/10176_39p0C_KO_Lx_HV_sTx03A_20D_10000Hz_18MHz_1000mS_00_EYE", path "\\\\Vantage-n-wk\\h/process bundle/VectorFlow Mouse Day 2 2018-01-25/2018-01-25 KO 10176/10176_39p5C_KO_Lx_HV_sTx03A_20D_10000Hz_18MHz_1000mS_00_EYE", path "\\\\Vantage-n-wk\\h/process bundle/VectorFlow Mouse Day 2 2018-01-25/2018-01-25 KO 10176/10176_39p5C_KO_Lx_HV_sTx03A_20D_10000Hz_18MHz_1000mS_01_EYE", path "\\\\Vantage-n-wk\\h/process bundle/VectorFlow Mouse Day 2 2018-01-25/2018-01-25 KO 10177/10177_35p5C_KO_Lx_HV_sTx03A_20D_20000Hz_18MHz_1000mS_00_EYE", path "\\\\Vantage-n-wk\\h/process bundle/VectorFlow Mouse Day 2 2018-01-25/2018-01-25 KO 10177/10177_35p5C_KO_Lx_HV_sTx03A_20D_20000Hz_18MHz_1000mS_01_EYE", path "\\\\Vantage-n-wk\\h/process bundle/VectorFlow Mouse Day 2 2018-01-25/2018-01-25 KO 10177/10177_35p5C_KO_Lx_HV_sTx03A_20D_20000Hz_18MHz_1000mS_02_EYE", path "\\\\Vantage-n-wk\\h/process bundle/VectorFlow Mouse Day 2 2018-01-25/2018-01-25 KO 10177/10177_35p5C_KO_Lx_HV_sTx03A_20D_20000Hz_18MHz_1000mS_03_EYE", path "\\\\Vantage-n-wk\\h/process bundle/VectorFlow Mouse Day 2 2018-01-25/2018-01-25 KO 10177/10177_36p0C_KO_Lx_HV_sTx03A_20D_20000Hz_18MHz_1000mS_00_EYE", path "\\\\Vantage-n-wk\\h/process bundle/VectorFlow Mouse Day 2 2018-01-25/2018-01-25 KO 10177/10177_36p5C_KO_Lx_HV_sTx03A_20D_20000Hz_18MHz_1000mS_00_EYE", path "\\\\Vantage-n-wk\\h/process bundle/VectorFlow Mouse Day 2 2018-01-25/2018-01-25 KO 10177/10177_37p0C_KO_Lx_HV_sTx03A_20D_20000Hz_18MHz_1000mS_00_EYE", path "\\\\Vantage-n-wk\\h/process bundle/VectorFlow Mouse Day 2 2018-01-25/2018-01-25 KO 10177/10177_37p0C_KO_Lx_HV_sTx03A_20D_20000Hz_18MHz_1000mS_01_EYE", path "\\\\Vantage-n-wk\\h/process bundle/VectorFlow Mouse Day 2 2018-01-25/2018-01-25 KO 10177/10177_37p5C_KO_Lx_HV_sTx03A_20D_20000Hz_18MHz_1000mS_00_EYE", path "\\\\Vantage-n-wk\\h/process bundle/VectorFlow Mouse Day 2 2018-01-25/2018-01-25 KO 10177/10177_38p0C_KO_Lx_HV_sTx03A_20D_20000Hz_18MHz_1000mS_00_EYE", path "\\\\Vantage-n-wk\\h/process bundle/VectorFlow Mouse Day 2 2018-01-25/2018-01-25 KO 10177/10177_38p0C_KO_Lx_HV_sTx03A_20D_20000Hz_18MHz_1000mS_01_EYE", path "\\\\Vantage-n-wk\\h/process bundle/VectorFlow Mouse Day 2 2018-01-25/2018-01-25 KO 10177/10177_38p5C_KO_Lx_HV_sTx03A_20D_20000Hz_18MHz_1000mS_00_EYE", path "\\\\Vantage-n-wk\\h/process bundle/VectorFlow Mouse Day 2 2018-01-25/2018-01-25 KO 10177/10177_39p0C_KO_Lx_HV_sTx03A_20D_20000Hz_18MHz_1000mS_00_EYE", path "\\\\Vantage-n-wk\\h/process bundle/VectorFlow Mouse Day 2 2018-01-25/2018-01-25 KO 10177/10177_39p0C_KO_Lx_HV_sTx03A_20D_20000Hz_18MHz_1000mS_01_EYE", path "\\\\Vantage-n-wk\\h/process bundle/VectorFlow Mouse Day 2 2018-01-25/2018-01-25 KO 10177/10177_39p5C_KO_Lx_HV_sTx03A_20D_20000Hz_18MHz_1000mS_00_EYE", path "\\\\Vantage-n-wk\\h/process bundle/VectorFlow Mouse Day 2 2018-01-25/2018-01-25 KO 10177/10177_39p5C_KO_Lx_HV_sTx03A_20D_20000Hz_18MHz_1000mS_01_EYE", path "\\\\Vantage-n-wk\\h/process bundle/VectorFlow Mouse Day 2 2018-01-25/2018-01-25 KO 10177/10177_40p0C_KO_Lx_HV_sTx03A_20D_20000Hz_18MHz_1000mS_00_EYE", path "\\\\Vantage-n-wk\\h/process bundle/VectorFlow Mouse Day 2 2018-01-25/2018-01-25 KO 10177/10177_40p0C_KO_Lx_HV_sTx03A_20D_20000Hz_18MHz_1000mS_01_EYE", path "\\\\Vantage-n-wk\\h/process bundle/VectorFlow Mouse Day 2 2018-01-25/2018-01-25 KO 10177/10177_40p5C_KO_Lx_HV_sTx03A_20D_20000Hz_18MHz_1000mS_00_EYE", path "\\\\Vantage-n-wk\\h/process bundle/VectorFlow Mouse Day 2 2018-01-25/2018-01-25 KO 10177/10177_40p5C_KO_Lx_HV_sTx03A_20D_20000Hz_18MHz_1000mS_01_EYE", path "\\\\Vantage-n-wk\\h/process bundle/VectorFlow Mouse Day 2 2018-01-25/2018-01-25 KO 10177/10177_41p0C_KO_Lx_HV_sTx03A_20D_20000Hz_18MHz_1000mS_00_EYE", path "\\\\Vantage-n-wk\\h/process bundle/VectorFlow Mouse Day 2 2018-01-25/2018-01-25 KO 10177/10177_41p0C_KO_Lx_HV_sTx03A_20D_20000Hz_18MHz_1000mS_01_EYE", path "\\\\Vantage-n-wk\\h/process bundle/VectorFlow Mouse Day 2 2018-01-25/2018-01-25 KO 10177/10177_41p0C_KO_Lx_HV_sTx03A_20D_20000Hz_18MHz_1000mS_02_EYE", path "\\\\Vantage-n-wk\\h/process bundle/VectorFlow Mouse Day 2 2018-01-25/2018-01-25 KO 10177/10177_41p0C_KO_Lx_HV_sTx03A_20D_20000Hz_18MHz_1000mS_03_EYE", path "\\\\Vantage-n-wk\\h/process bundle/VectorFlow Mouse Day 2 2018-01-25/2018-01-25 KO 10178/10178_34p0C_KO_Lx_HV_sTx03A_20D_20000Hz_18MHz_1000mS_00_EYE", path "\\\\Vantage-n-wk\\h/process bundle/VectorFlow Mouse Day 2 2018-01-25/2018-01-25 KO 10178/10178_34p5C_KO_Lx_HV_sTx03A_20D_20000Hz_18MHz_1000mS_00_EYE", path "\\\\Vantage-n-wk\\h/process bundle/VectorFlow Mouse Day 2 2018-01-25/2018-01-25 KO 10178/10178_35p0C_KO_Lx_HV_sTx03A_20D_20000Hz_18MHz_1000mS_00_EYE", path "\\\\Vantage-n-wk\\h/process bundle/VectorFlow Mouse Day 2 2018-01-25/2018-01-25 KO 10178/10178_35p5C_KO_Lx_HV_sTx03A_20D_20000Hz_18MHz_1000mS_00_EYE", path "\\\\Vantage-n-wk\\h/process bundle/VectorFlow Mouse Day 2 2018-01-25/2018-01-25 KO 10178/10178_35p5C_KO_Lx_HV_sTx03A_20D_20000Hz_18MHz_1000mS_01_EYE", path "\\\\Vantage-n-wk\\h/process bundle/VectorFlow Mouse Day 2 2018-01-25/2018-01-25 KO 10178/10178_36p0C_KO_Lx_HV_sTx03A_20D_20000Hz_18MHz_1000mS_00_EYE", path "\\\\Vantage-n-wk\\h/process bundle/VectorFlow Mouse Day 2 2018-01-25/2018-01-25 KO 10178/10178_36p5C_KO_Lx_HV_sTx03A_20D_20000Hz_18MHz_1000mS_00_EYE", path "\\\\Vantage-n-wk\\h/process bundle/VectorFlow Mouse Day 2 2018-01-25/2018-01-25 KO 10178/10178_37p0C_KO_Lx_HV_sTx03A_20D_20000Hz_18MHz_1000mS_00_EYE", path "\\\\Vantage-n-wk\\h/process bundle/VectorFlow Mouse Day 2 2018-01-25/2018-01-25 KO 10178/10178_37p5C_KO_Lx_HV_sTx03A_20D_20000Hz_18MHz_1000mS_00_EYE", path "\\\\Vantage-n-wk\\h/process bundle/VectorFlow Mouse Day 2 2018-01-25/2018-01-25 KO 10178/10178_37p5C_KO_Lx_HV_sTx03A_20D_20000Hz_18MHz_1000mS_01_EYE", path "\\\\Vantage-n-wk\\h/process bundle/VectorFlow Mouse Day 2 2018-01-25/2018-01-25 KO 10178/10178_37p5C_KO_Lx_HV_sTx03A_20D_20000Hz_18MHz_1000mS_02_EYE", path "\\\\Vantage-n-wk\\h/process bundle/VectorFlow Mouse Day 2 2018-01-25/2018-01-25 KO 10178/10178_37p5C_KO_Lx_HV_sTx03A_20D_20000Hz_18MHz_1000mS_03_EYE", path "\\\\Vantage-n-wk\\h/process bundle/VectorFlow Mouse Day 2 2018-01-25/2018-01-25 KO 10178/10178_38p0C_KO_Lx_HV_sTx03A_20D_20000Hz_18MHz_1000mS_00_EYE", path "\\\\Vantage-n-wk\\h/process bundle/VectorFlow Mouse Day 2 2018-01-25/2018-01-25 KO 10178/10178_39p0C_KO_Lx_HV_sTx03A_20D_20000Hz_18MHz_1000mS_00_EYE", path "\\\\Vantage-n-wk\\h/process bundle/VectorFlow Mouse Day 2 2018-01-25/2018-01-25 KO 10178/10178_39p5C_KO_Lx_HV_sTx03A_20D_20000Hz_18MHz_1000mS_00_EYE", path "\\\\Vantage-n-wk\\h/process bundle/VectorFlow Mouse Day 2 2018-01-25/2018-01-25 KO 10178/10178_39p5C_KO_Lx_HV_sTx03A_20D_20000Hz_18MHz_1000mS_01_EYE", path "\\\\Vantage-n-wk\\h/process bundle/VectorFlow Mouse Day 2 2018-01-25/2018-01-25 KO 10178/10178_40p0C_KO_Lx_HV_sTx03A_20D_20000Hz_18MHz_1000mS_00_EYE", path "\\\\Vantage-n-wk\\h/process bundle/VectorFlow Mouse Day 2 2018-01-25/2018-01-25 KO 10178/10178_40p5C_KO_Lx_HV_sTx03A_20D_20000Hz_18MHz_1000mS_00_EYE", path "\\\\Vantage-n-wk\\h/process bundle/VectorFlow Mouse Day 2 2018-01-25/2018-01-25 WT 10130/10130_36p5C_WT_Lx_HV_sTx03A_20D_10000Hz_18MHz_1000mS_00_EYE", path "\\\\Vantage-n-wk\\h/process bundle/VectorFlow Mouse Day 2 2018-01-25/2018-01-25 WT 10130/10130_36p5C_WT_Lx_HV_sTx03A_20D_10000Hz_18MHz_1000mS_01_EYE", path "\\\\Vantage-n-wk\\h/process bundle/VectorFlow Mouse Day 2 2018-01-25/2018-01-25 WT 10130/10130_36p5C_WT_Lx_HV_sTx03A_20D_10000Hz_18MHz_1000mS_02_EYE", path "\\\\Vantage-n-wk\\h/process bundle/VectorFlow Mouse Day 2 2018-01-25/2018-01-25 WT 10130/10130_37p0C_WT_Lx_HV_sTx03A_20D_10000Hz_18MHz_1000mS_00_EYE", path "\\\\Vantage-n-wk\\h/process bundle/VectorFlow Mouse Day 2 2018-01-25/2018-01-25 WT 10130/10130_37p5C_WT_Lx_HV_sTx03A_20D_10000Hz_18MHz_1000mS_00_EYE", path "\\\\Vantage-n-wk\\h/process bundle/VectorFlow Mouse Day 2 2018-01-25/2018-01-25 WT 10130/10130_38p0C_WT_Lx_HV_sTx03A_20D_10000Hz_18MHz_1000mS_00_EYE", path "\\\\Vantage-n-wk\\h/process bundle/VectorFlow Mouse Day 2 2018-01-25/2018-01-25 WT 10130/10130_38p0C_WT_Lx_HV_sTx03A_20D_10000Hz_18MHz_1000mS_01_EYE", path "\\\\Vantage-n-wk\\h/process bundle/VectorFlow Mouse Day 2 2018-01-25/2018-01-25 WT 10130/10130_39p0C_WT_Lx_HV_sTx03A_20D_10000Hz_18MHz_1000mS_00_EYE", path "\\\\Vantage-n-wk\\h/process bundle/VectorFlow Mouse Day 2 2018-01-25/2018-01-25 WT 10130/10130_40p0C_WT_Lx_HV_sTx03A_20D_10000Hz_18MHz_1000mS_00_EYE", path "\\\\Vantage-n-wk\\h/process bundle/VectorFlow Mouse Day 2 2018-01-25/2018-01-25 WT 10130/10130_40p5C_WT_Lx_HV_sTx03A_20D_10000Hz_18MHz_1000mS_00_EYE", path "\\\\Vantage-n-wk\\h/process bundle/VectorFlow Mouse Day 2 2018-01-25/2018-01-25 WT 10130/10130_40p5C_WT_Lx_HV_sTx03A_20D_10000Hz_18MHz_1000mS_01_EYE", path "\\\\Vantage-n-wk\\h/process bundle/VectorFlow Mouse Day 2 2018-01-25/2018-01-25 WT 10130/10130_40p5C_WT_Lx_HV_sTx03A_20D_10000Hz_18MHz_1000mS_02_EYE", path "\\\\Vantage-n-wk\\h/process bundle/VectorFlow Mouse Day 2 2018-01-25/2018-01-25 WT 10130/10130_41p0C_WT_Lx_HV_sTx03A_20D_10000Hz_18MHz_1000mS_00_EYE", path "\\\\Vantage-n-wk\\h/process bundle/VectorFlow Mouse Day 3 2018-02-09/2018-02-09 KO 10129/10129_37p0C_NO_sTx03A_20D_10000Hz_18MHz_0500mS_01_EYE", path "\\\\Vantage-n-wk\\h/process bundle/VectorFlow Mouse Day 3 2018-02-09/2018-02-09 KO 10129/10129_38p5C_NO_sTx03A_20D_10000Hz_18MHz_0500mS_00_EYE", path "\\\\Vantage-n-wk\\h/process bundle/VectorFlow Mouse Day 3 2018-02-09/2018-02-09 KO 10129/10129_39p0C_NO_sTx03A_20D_10000Hz_18MHz_0500mS_00_EYE", path "\\\\Vantage-n-wk\\h/process bundle/VectorFlow Mouse Day 3 2018-02-09/2018-02-09 KO 10129/10129_39p5C_NO_sTx03A_20D_10000Hz_18MHz_0500mS_00_EYE", path "\\\\Vantage-n-wk\\h/process bundle/VectorFlow Mouse Day 3 2018-02-09/2018-02-09 KO 10129/10129_40p0C_NO_sTx03A_20D_10000Hz_18MHz_0500mS_00_EYE", path "\\\\Vantage-n-wk\\h/process bundle/VectorFlow Mouse Day 3 2018-02-09/2018-02-09 KO 10129/10129_40p0C_NO_sTx03A_20D_10000Hz_18MHz_0500mS_01_EYE", path "\\\\Vantage-n-wk\\h/process bundle/VectorFlow Mouse Day 3 2018-02-09/2018-02-09 KO 10129/10129_40p5C_NO_sTx03A_20D_10000Hz_18MHz_0500mS_00_EYE", path "\\\\Vantage-n-wk\\h/process bundle/VectorFlow Mouse Day 3 2018-02-09/2018-02-09 KO 10129/10129_41p0C_NO_sTx03A_20D_10000Hz_18MHz_0500mS_00_EYE", path "\\\\Vantage-n-wk\\h/process bundle/VectorFlow Mouse Day 3 2018-02-09/2018-02-09 KO 10129/10129_41p2C_NO_USD_sTx03A_20D_10000Hz_18MHz_0500mS_00_EYE", path "\\\\Vantage-n-wk\\h/process bundle/VectorFlow Mouse Day 3 2018-02-09/2018-02-09 KOPF 10135/10135_34p0C_KOPF_sTx03A_10D_10000Hz_18MHz_1000mS_00_EYE", path "\\\\Vantage-n-wk\\h/process bundle/VectorFlow Mouse Day 3 2018-02-09/2018-02-09 KOPF 10135/10135_34p0C_KOPF_sTx03A_20D_10000Hz_18MHz_1000mS_00_EYE", path "\\\\Vantage-n-wk\\h/process bundle/VectorFlow Mouse Day 3 2018-02-09/2018-02-09 KOPF 10135/10135_34p0C_KOPF_sTx03A_20D_10000Hz_18MHz_1000mS_01_EYE", path "\\\\Vantage-n-wk\\h/process bundle/VectorFlow Mouse Day 3 2018-02-09/2018-02-09 KOPF 10135/10135_34p0C_KOPF_sTx03A_20D_10000Hz_18MHz_1000mS_02_EYE", path "\\\\Vantage-n-wk\\h/process bundle/VectorFlow Mouse Day 3 2018-02-09/2018-02-09 KOPF 10135/10135_34p0C_KOPF_sTx05A_10D_06000Hz_18MHz_1000mS_00_EYE", path "\\\\Vantage-n-wk\\h/process bundle/VectorFlow Mouse Day 3 2018-02-09/2018-02-09 KOPF 10135/10135_34p0C_KOPF_sTx05A_10D_06000Hz_18MHz_1000mS_01_EYE", path "\\\\Vantage-n-wk\\h/process bundle/VectorFlow Mouse Day 3 2018-02-09/2018-02-09 KOPF 10135/10135_34p0C_KOPF_sTx05A_20D_06000Hz_18MHz_1000mS_00_EYE", path "\\\\Vantage-n-wk\\h/process bundle/VectorFlow Mouse Day 3 2018-02-09/2018-02-09 KOPF 10135/10135_37p0C_KOPF_sTx03A_10D_10000Hz_18MHz_1000mS_00_EYE", path "\\\\Vantage-n-wk\\h/process bundle/VectorFlow Mouse Day 3 2018-02-09/2018-02-09 KOPF 10135/10135_37p5C_KOPF_sTx03A_10D_10000Hz_18MHz_1000mS_00_EYE", path "\\\\Vantage-n-wk\\h/process bundle/VectorFlow Mouse Day 3 2018-02-09/2018-02-09 KOPF 10135/10135_37p5C_KOPF_sTx03A_10D_10000Hz_18MHz_1000mS_01_EYE", path "\\\\Vantage-n-wk\\h/process bundle/VectorFlow Mouse Day 3 2018-02-09/2018-02-09 WT 10128/10128_37p0C_WT_sTx03A_20D_10000Hz_18MHz_0500mS_00_EYE", path "\\\\Vantage-n-wk\\h/process bundle/VectorFlow Mouse Day 3 2018-02-09/2018-02-09 WT 10128/10128_38p0C_WT_sTx03A_20D_10000Hz_18MHz_0500mS_00_EYE", path "\\\\Vantage-n-wk\\h/process bundle/VectorFlow Mouse Day 3 2018-02-09/2018-02-09 WT 10128/10128_38p0C_WT_sTx03A_20D_10000Hz_18MHz_0500mS_01_EYE", path "\\\\Vantage-n-wk\\h/process bundle/VectorFlow Mouse Day 3 2018-02-09/2018-02-09 WT 10128/10128_39p0C_WT_sTx03A_20D_10000Hz_18MHz_0500mS_00_EYE", path "\\\\Vantage-n-wk\\h/process bundle/VectorFlow Mouse Day 3 2018-02-09/2018-02-09 WT 10128/10128_39p5C_WT_sTx03A_20D_10000Hz_18MHz_0500mS_00_EYE", path "\\\\Vantage-n-wk\\h/process bundle/VectorFlow Mouse Day 3 2018-02-09/2018-02-09 WT 10128/10128_40p0C_WT_sTx03A_20D_10000Hz_18MHz_0500mS_00_EYE", path "\\\\Vantage-n-wk\\h/process bundle/VectorFlow Mouse Day 3 2018-02-09/2018-02-09 WT 10128/10128_40p0C_WT_sTx03A_20D_10000Hz_18MHz_0500mS_01_EYE", path "\\\\Vantage-n-wk\\h/process bundle/VectorFlow Mouse Day 3 2018-02-09/2018-02-09 WT 10128/10128_40p5C_WT_sTx03A_20D_10000Hz_18MHz_0500mS_00_EYE", path "\\\\Vantage-n-wk\\h/process bundle/VectorFlow Mouse Day 3 2018-02-09/2018-02-09 WT 10130/10130_35p0C_WT_sTx03A_20D_10000Hz_18MHz_0500mS_00_EYE", path "\\\\Vantage-n-wk\\h/process bundle/VectorFlow Mouse Day 3 2018-02-09/2018-02-09 WT 10130/10130_35p5C_WT_sTx03A_20D_10000Hz_25MHz_0500mS_00_EYE", path "\\\\Vantage-n-wk\\h/process bundle/VectorFlow Mouse Day 3 2018-02-09/2018-02-09 WT 10130/10130_36p0C_WT_sTx03A_20D_10000Hz_21MHz_0500mS_00_EYE", path "\\\\Vantage-n-wk\\h/process bundle/VectorFlow Mouse Day 3 2018-02-09/2018-02-09 WT 10130/10130_36p5C_WT_sTx03A_20D_10000Hz_18MHz_0500mS_00_EYE", path "\\\\Vantage-n-wk\\h/process bundle/VectorFlow Mouse Day 3 2018-02-09/2018-02-09 WT 10130/10130_36p5C_WT_sTx03A_20D_10000Hz_18MHz_0500mS_01_EYE", path "\\\\Vantage-n-wk\\h/process bundle/VectorFlow Mouse Day 3 2018-02-09/2018-02-09 WT 10130/10130_37p0C_WT_sTx03A_20D_10000Hz_18MHz_0500mS_00_EYE", path "\\\\Vantage-n-wk\\h/process bundle/VectorFlow Mouse Day 3 2018-02-09/2018-02-09 WT 10130/10130_37p5C_WT_sTx03A_20D_10000Hz_18MHz_0500mS_00_EYE", path "\\\\Vantage-n-wk\\h/process bundle/VectorFlow Mouse Day 3 2018-02-09/2018-02-09 WT 10130/10130_38p0C_WT_sTx03A_20D_10000Hz_18MHz_0500mS_00_EYE", path "\\\\Vantage-n-wk\\h/process bundle/VectorFlow Mouse Day 3 2018-02-09/2018-02-09 WT 10130/10130_39p0C_WT_sTx03A_20D_10000Hz_18MHz_0500mS_00_EYE", path "\\\\Vantage-n-wk\\h/process bundle/VectorFlow Mouse Day 3 2018-02-09/2018-02-09 WT 10130/10130_39p0C_WT_sTx03A_20D_10000Hz_18MHz_0500mS_01_EYE", path "\\\\Vantage-n-wk\\h/process bundle/VectorFlow Mouse Day 3 2018-02-09/2018-02-09 WT 10130/10130_40p0C_WT_sTx03A_20D_10000Hz_18MHz_0500mS_00_EYE", path "\\\\Vantage-n-wk\\h/process bundle/VectorFlow Mouse Day 3 2018-02-09/2018-02-09 WT 10130/10130_40p0C_WT_sTx03A_20D_10000Hz_18MHz_0500mS_01_EYE", path "\\\\Vantage-n-wk\\h/process bundle/VectorFlow Mouse Day 3 2018-02-09/2018-02-09 WT 10130/10130_41p0C_WT_sTx03A_20D_10000Hz_18MHz_0500mS_00_EYE", path "\\\\Vantage-n-wk\\h/process bundle/VectorFlow Mouse Day 3 2018-02-09/2018-02-09 WT 10132/10132_37p5C_WT_sTx03A_20D_10000Hz_18MHz_0500mS_00_EYE", path "\\\\Vantage-n-wk\\h/process bundle/VectorFlow Mouse Day 3 2018-02-09/2018-02-09 WT 10132/10132_38p0C_WT_sTx03A_20D_10000Hz_18MHz_0500mS_00_EYE", path "\\\\Vantage-n-wk\\h/process bundle/VectorFlow Mouse Day 3 2018-02-09/2018-02-09 WT 10132/10132_38p0C_WT_sTx03A_20D_10000Hz_18MHz_0500mS_01_EYE", path "\\\\Vantage-n-wk\\h/process bundle/VectorFlow Mouse Day 3 2018-02-09/2018-02-09 WT 10132/10132_38p0C_WT_sTx03A_20D_10000Hz_18MHz_0500mS_02_EYE", path "\\\\Vantage-n-wk\\h/process bundle/VectorFlow Mouse Day 3 2018-02-09/2018-02-09 WT 10132/10132_38p0C_WT_sTx03A_20D_10000Hz_18MHz_0500mS_03_EYE", path "\\\\Vantage-n-wk\\h/process bundle/VectorFlow Mouse Day 3 2018-02-09/2018-02-09 WT 10132/10132_38p0C_WT_sTx03A_20D_10000Hz_18MHz_0500mS_04_EYE", path "\\\\Vantage-n-wk\\h/process bundle/VectorFlow Mouse Day 3 2018-02-09/2018-02-09 WT 10132/10132_38p5C_WT_sTx03A_20D_10000Hz_18MHz_0500mS_00_EYE", path "\\\\Vantage-n-wk\\h/process bundle/VectorFlow Mouse Day 3 2018-02-09/2018-02-09 WT 10132/10132_39p0C_WT_sTx03A_20D_10000Hz_18MHz_0500mS_00_EYE", path "\\\\Vantage-n-wk\\h/process bundle/VectorFlow Mouse Day 3 2018-02-09/2018-02-09 WT 10132/10132_39p0C_WT_sTx03A_20D_10000Hz_18MHz_0500mS_01_EYE", path "\\\\Vantage-n-wk\\h/process bundle/VectorFlow Mouse Day 3 2018-02-09/2018-02-09 WT 10132/10132_39p5C_WT_sTx03A_20D_10000Hz_18MHz_0500mS_00_EYE", path "\\\\Vantage-n-wk\\h/process bundle/VectorFlow Mouse Day 3 2018-02-09/2018-02-09 WT 10132/10132_40p0C_WT_sTx03A_20D_10000Hz_18MHz_0500mS_00_EYE", path "\\\\Vantage-n-wk\\h/process bundle/VectorFlow Mouse Day 3 2018-02-09/2018-02-09 WT 10132/10132_40p5C_WT_sTx03A_20D_10000Hz_18MHz_0500mS_00_EYE", path "\\\\Vantage-n-wk\\h/process bundle/VectorFlow Mouse Day 3 2018-02-09/2018-02-09 WT 10132/10132_41p0C_WT_sTx03A_20D_10000Hz_18MHz_0500mS_00_EYE", path "\\\\Vantage-n-wk\\h/process bundle/VectorFlow Mouse Day 3 2018-02-09/2018-02-09 WT 10132/10132_41p0C_WT_sTx03A_20D_10000Hz_18MHz_0500mS_01_EYE"] ("Paths to process"), index=0) -> (w22:path[])  [unwired: 1 in]
        }
        frame True {
          n12 = call <vilib>:"Recursive File List.vi"("Folders to Exclude"=string[] ["$RECYCLE.BIN", "System Volume Information", "*EYE_Doppler", "*_EYE"], "pattern"=w25, "Folder Path"="Choose Top level folder") -> ("All Files in Dir"=w26:path[])  [unwired: 4 in, 4 out]
        }
      }
    }
  }
  "Paths to process" <- w2
  n13 = for {
    tunnel: w2 -> [w33] mode=indexing
    tunnel: "Batch Spectorgram" -> [w32]
    tunnel: "Batch BPM" -> [w31]
    tunnel: "file ext search" -> [w30]
    i -> [w29]
    n14 = while {
      tunnel: w33 -> [w38]
      tunnel: w32 -> [w40]
      tunnel: w31 -> [w39]
      tunnel: w30 -> [w37]
      tunnel: w29 -> [w34]
      stop <- w41 stop-if-true
      n15 = local read "Doppler Params"() -> (w36:T2)
      n16 = stacked-sequence {
        seq-local: [_ w87 _ _] -> [_ _ _ w195]
        seq-local: [_ w95 _ _] -> [_ _ _ w194]
        seq-local: [w45 _ _ _] -> [_ w91 w148 w187]
        seq-local: [w49 _ _ _] -> [_ w96 _ _]
        tunnel: [_ _ _ w196] -> w42
        tunnel: [_ _ _ w189] -> w43
        tunnel: w40 -> [w54 _ _ w190]
        tunnel: w39 -> [w53 _ _ w191]
        tunnel: w38 -> [w51 w107 _ w188]
        tunnel: w37 -> [w50 _ _ _]
        tunnel: w36 -> [w48 w88 _ _]
        tunnel: "# of files" -> [w47 w90 _ _]
        tunnel: w34 -> [_ _ _ w186]
        frame #0 {
          # "Total lateral"
          n17 = case shown="True" "read?" {
            tunnel: w51 -> [_ w76]
            tunnel: ["Header Out" w70] -> w44
            tunnel: w47 -> [_ w73]
            tunnel: w50 -> [_ w72]
            tunnel: [w62 w65] -> w49
            frame False {
              n18 = local read "Raw Complex output array"() -> (w62:csg[][][])
            }
            frame True {
              n19 = call "LoadEyeArray.vi"("directory path of data and header file"=w76, "Split files?"="Split files?", "Type of Read"="Type of Read 2", "String"=w72, "Only Buff 3?"="Only Buff 3?", "Only Real of Sum?"="Only Real of Sum?", "Cut off"=w73) -> ("RcvBuff 3"=w67:cdb[][][], "output array"=w66:i32[][][], "Header Out"=w70:T1)  [unwired: 4 in, 2 out]
              n20 = Select(t=w66, s="Only Real of Sum?", f=w67) -> (s? t:f=w65:cdb[][][])
              "Raw Complex output array" <- w65
              n21 = for {
                tunnel: w65 -> [w82] mode=indexing
                tunnel: [w81] -> w78 mode=indexing
                n22 = Absolute Value(x=w82) -> (abs(x)=w83:dbl[][])
                n23 = expression code="20*log(x)"(w83) -> (w84:dbl[][])
                n24 = Array Max & Min(array=w84) -> (max value=w81:dbl)  [unwired: 3 out]
                n25 = Subtract(x=w84, y=w81) -> (x-y=→"Raw data":dbl[][])
              }
              n26 = Unbundle By Name(w70) -> ("Tranducer Info.center freq"=→"Original Fc":sgl)
              n27 = Array Size(array=w65) -> (size(s)=w75:i32[])
              n28 = Index Array(array=w75) -> (element=→"Total Files":i32)  [unwired: 1 in]
              n29 = local write "Header Out"(w70) -> ()
              n30 = Array Max & Min(array=w78) -> (max value=→"max value":dbl)  [unwired: 3 out]
            }
          }
          n31 = case shown="True" w54 {
            tunnel: w48 -> [w59 _]
            tunnel: [w58 w61] -> w52
            frame False {
              n32 = property on="Doppler Params" class="Clust (strict)"("Val(Sgnl)"=w59) -> (error out=w58:errorcluster)  [unwired: 2 in, 1 out]
            }
            frame True {
              n33 = property on="save spectorgrams" class="Bool (strict)"("Val(Sgnl)"=FALSE ("Value (Signaling)")) -> (error out=w61:errorcluster)  [unwired: 2 in, 1 out]
            }
          }
          n34 = case shown="True" w53 {
            tunnel: w52 -> [_ w56]
            frame False {
            }
            frame True {
              n35 = local read "Cycles"() -> (w57:i32)
              n36 = property on="Cycles" class="DigNum (strict)"(error in=w56, "Val(Sgnl)"=w57) -> ()  [unwired: 1 in, 2 out]
            }
          }
          n37 = Bundle By Name(cluster=w44, "Tranducer Info.center freq"="True Center Freq") -> (w45:T1)
        }
        frame #1 {
          n38 = Strip Path(path=w107) -> (stripped path=w109:path)  [unwired: 1 out]
          n39 = local write "Choose Directory"(w109) -> ()
          n40 = local read "#x lines"() -> (w85:i32)
          n41 = property on="#x lines" class="DigNum (strict)"("Val(Sgnl)"=w85) -> ()  [unwired: 2 in, 2 out]
          n42 = property on="image to display" class="DigNum (strict)"("Val(Sgnl)"="image to display") -> ()  [unwired: 2 in, 2 out]
          n43 = case shown="True" "Use VPI crop?" {
            tunnel: w91 -> [_ w129]
            tunnel: w109 -> [_ w128]
            tunnel: [w119 w125] -> w104
            tunnel: [w118 w124] -> w102
            tunnel: [w117 w122] -> w103
            tunnel: [w116 w123] -> w101
            frame False {
              n44 = property on="Raw data" class="IntGraph (strict)"("Active Cursor"=u32 0, "Active Cursor"=u32 1) -> ("Cursor.Cursor X"=w119:dbl, "Cursor.Cursor Y"=w118:dbl, "Cursor.Cursor X"=w117:dbl, "Cursor.Cursor Y"=w116:dbl)  [unwired: 2 in, 2 out]
            }
            frame True {
              n45 = call "ConvertCropsFromMatlab.vi"("Choose Crop File?"="Choose Crop File?", "Crop file"="Crop file", "Header In"=w129, "Directory"=w128) -> ("crop marks"=w137:T7)  [unwired: 7 in]
              n46 = Unbundle(w137) -> ("Line start"=w134:dbl, "# of lines"=w136:dbl, "RF start"=w133:dbl, "# pts"=w135:dbl)
              n47 = Add(x=w134, y=w136) -> (x+y=w132:dbl)
              n48 = Add(x=w133, y=w135) -> (x+y=w131:dbl)
              n49 = case shown="False" FALSE {
                tunnel: w134 -> [_ w147]
                tunnel: w133 -> [_ w146]
                tunnel: w132 -> [_ w145]
                tunnel: w131 -> [_ w144]
                tunnel: [w143 w147] -> w125
                tunnel: [w143 w146] -> w124
                tunnel: [w140 w145] -> w122
                tunnel: [w141 w144] -> w123
                tunnel: w129 -> [w142 _]
                frame False {
                  w143 = u32 0 ("Active Cursor")
                  n50 = Unbundle By Name(w142) -> ("A/D info.# lines per scan"=w140:u16, "A/D info.# rf points per line"=w141:u16)
                }
                frame True {
                }
              }
              n51 = property on="Raw data" class="IntGraph (strict)"("Active Cursor"=u32 0, "Cursor.Cursor X"=w125, "Cursor.Cursor Y"=w124, "Active Cursor"=u32 1, "Cursor.Cursor X"=w122, "Cursor.Cursor Y"=w123) -> ()  [unwired: 2 in, 2 out]
            }
          }
          n52 = Subtract(x=w101, y=w102) -> (x-y=w106:dbl)
          n53 = Subtract(x=w103, y=w104) -> (x-y=w105:dbl)
          n54 = Bundle("Line start"=w104, w105, "RF start"=w102, w106) -> (w95:T8)  [unwired: 1 in]
          n55 = Unbundle(w95) -> ("Line start"=w100:dbl, w99:dbl, "RF start"=w98:dbl, w97:dbl)
          n56 = Array Subset(array=w96, index (dim 1)=w100, length (dim 1)=w99, index (dim 2)=w98, length (dim 2)=w97) -> (w89:cdb[][][])  [unwired: 2 in]
          n57 = case shown="True" "SVD?" {
            tunnel: [w110 w115] -> w93
            tunnel: w89 -> [w110 w114]
            tunnel: w88 -> [_ w113]
            tunnel: w91 -> [_ w111]
            frame False {
            }
            frame True {
              n58 = local read "maxPRF?"() -> (w112:bool)
              n59 = call "Doppler_SVM_3D.vi"("PRF1/2"=w112, "Doppler Params"=w113, "Header In"=w111, "Complex output array"=w114) -> ("Filtered Out"=w115:csg[][][])  [unwired: 7 in]
            }
          }
          n60 = Array Subset(array=w93, index (dim 0)="start", length (dim 0)=w90) -> (w87:cdb[][][])  [unwired: 4 in]
        }
        frame #2 {
          # "Set up 1:1 aspect ratio and set image scale"
          # "Total depth"
          n61 = Unbundle By Name(w148) -> ("Scan Settings.Distance between\nscan lines (um)"=w158:u16)
          n62 = Unbundle By Name(w148) -> ("A/D info.# rf points per line"=w161:u16, "A/D info.sample rate MHz"=w163:u16, "A/D info.# lines per scan"=w160:u16)
          n63 = Unbundle By Name(w148) -> ("Misc Info.c speed"=w157:i16)
          n64 = Unbundle By Name(w148) -> ("Scan Info.delay"=w153:sgl)
          n65 = Multiply(x=0.0005, y=w157) -> (x*y=w155:dbl)
          n66 = Reciprocal(x=w163) -> (1/x=w164:dbl)
          n67 = Multiply(x=w164, y=w155) -> (x*y=w154:dbl)
          n68 = Multiply(x=w161, y=w154) -> (x*y=w162:dbl)
          n69 = Divide(x=w158, y=1000) -> (x/y=w152:dbl)
          n70 = Divide(x=w162, y=w152) -> (x/y=w150:dbl)
          n71 = Decrement(x=w160) -> (x-1=w149:u16)
          n72 = Decrement(x=w161) -> (x-1=w159:u16)
          n73 = Bundle(w150, w149) -> (w151:cluster{dbl, u16})  [unwired: 1 out]
          n74 = flat-sequence {
            tunnel: w159 -> [w172]
            tunnel: w149 -> [w173]
            tunnel: w151 -> [w171]
            tunnel: [w175] -> w170
            tunnel: w154 -> [w175]
            tunnel: [w174] -> w169
            tunnel: w152 -> [w174]
            tunnel: [w173] -> w168
            tunnel: [w172] -> w167
            tunnel: [w171] -> w166
            tunnel: w170 -> [w181]
            tunnel: w153 -> [w179]
            tunnel: w169 -> [w180]
            tunnel: w168 -> [w185]
            tunnel: w167 -> [w184]
            tunnel: w166 -> [w182]
            tunnel: [w176] -> _
            frame #0 {
            }
            frame #1 {
              n75 = Multiply(x=w181, y=w184) -> (x*y=w183:dbl)
              n76 = Multiply(x=w180, y=w185) -> (x*y=w177:dbl)
              n77 = Add(x=w179, y=w183) -> (x+y=w178:dbl)
              n78 = Bundle(w182, w181, w180, "delay"=w179, "delay"=w179, w178, w177) -> (w176:T9)  [unwired: 1 out]
            }
          }
        }
        frame #3 {
          # "Raw Data"
          n79 = Or(x=w190, y=w191) -> (x .or. y?=w189:bool)
          n80 = call "DopplerScale.vi"("Header In"=w187, "PRF1/2"="maxPRF?") -> ("slow-time sampling"=w192:dbl)  [unwired: 6 in, 3 out]
          n81 = while {
            tunnel: w187 -> [w207]
            shift-right: [w219] -> _
            shift-left: w195 -> [w218]
            shift-right: [w217] -> _
            shift-left: _ -> [w216]
            tunnel: ["stop"] -> w196
            tunnel: w194 -> [w210]
            shift-right: [w209] -> _
            shift-left: _ -> [w208]
            tunnel: "maxPRF?" -> [w205]
            tunnel: w192 -> [w203]
            tunnel: w188 -> [w201]
            tunnel: w189 -> [w200]
            tunnel: w191 -> [w199]
            tunnel: w186 -> [w197]
            stop <- w213 stop-if-true
            # "Velocity"
            # "Mean Powerr"
            n82 = local read "Doppler Params"() -> (w204:T2)
            n83 = Bundle By Name(cluster=w204, "SlowTime (Hz)"=w203) -> (w202:T2)
            n84 = event shown="[8] \"image to display\", \"Log RF?\": Value Change" {
              selector: _ -> [_ _ _ _ _ _ _ _ _ _ _ _ _ _ _ _ _ _ _ _ _]
              dyn-events: _ -> [_ _ _ _ _ _ _ _ _ _ _ _ _ _ _ _ _ _ _ _ _]
              timeout: 50 -> [_ _ _ _ _ _ _ _ _ _ _ _ _ _ _ _ _ _ _ _ _]
              tunnel: w207 -> [_ w231 _ _ w621 _ _ _ _ w808 w1048 w1183 _ _ _ _ _ _ _ _ _]
              tunnel: [w224 w228 w521 w616 w624 w688 w734 w773 w788 w806 w1058 w1174 w1273 w1275 w1304 w1326 w1345 w1374 w1395 w1399 w1412] -> w219
              tunnel: w218 -> [w224 w228 w521 w616 w624 w688 w734 w773 w788 w806 w1058 w1174 w1273 w1275 w1304 w1326 w1345 w1374 w1395 w1399 w1412]
              tunnel: [w223 w234 w570 w615 w645 w687 w733 w772 w789 w809 w1062 w1177 w1272 w1295 w1303 w1319 w1357 w1367 w1390 w1398 w1411] -> w217
              tunnel: w216 -> [w223 w234 w570 w615 w645 w687 w733 w772 w789 _ w1062 w1177 w1272 w1295 w1303 w1319 w1357 w1367 w1390 w1398 w1411]
              tunnel: "Doppler Angle" -> [_ _ _ _ _ _ _ _ _ w805 _ w1179 _ _ _ _ _ _ _ _ _]
              tunnel: [w221 _ _ _ _ _ _ _ _ _ _ _ _ _ _ _ _ _ _ TRUE _] -> w212
              tunnel: TRUE ("timed out?") -> [_ w230 _ _ _ _ _ _ _ w804 w1042 w1181 _ _ _ _ _ _ _ _ _]
              tunnel: w210 -> [_ w225 _ _ _ _ _ _ _ w803 _ _ _ _ _ _ _ _ _ _ _]
              tunnel: [w222 w233 w569 w614 w634 w686 w732 w771 w778 w801 w1064 w1172 w1271 w1294 w1296 w1318 w1344 w1364 w1394 w1396 w1410] -> w209
              tunnel: w208 -> [w222 w233 w569 w614 w634 w686 w732 w771 w778 _ w1064 w1172 w1271 w1294 w1296 w1318 w1344 w1364 w1394 w1396 w1410]
              tunnel: w205 -> [_ w232 _ _ _ _ _ _ _ w800 w1043 w1182 _ _ _ _ _ _ _ _ _]
              tunnel: "Thresholds" -> [_ _ _ _ _ _ _ _ _ w798 w1057 _ _ _ _ _ _ _ _ _ _]
              tunnel: w203 -> [_ w229 _ _ _ _ _ _ _ _ _ _ _ _ _ _ _ _ _ _ _]
              tunnel: w202 -> [_ _ w562 _ _ w667 w706 _ _ w796 w1038 w1171 _ w1276 _ w1312 _ _ _ _ _]
              tunnel: w201 -> [_ w227 w555 w597 w641 w672 w719 _ _ _ _ _ _ _ _ _ _ _ _ _ _]
              tunnel: w200 -> [w221 _ _ _ _ _ _ _ _ _ _ _ _ _ _ _ _ _ _ _ _]
              tunnel: w199 -> [_ _ _ _ _ _ w718 _ _ _ _ _ _ _ _ _ _ _ _ _ _]
              tunnel: "Save Tiled" -> [_ w226 _ _ _ _ _ _ _ _ _ _ _ _ _ _ _ _ _ _ _]
              tunnel: w197 -> [_ _ w544 _ _ _ _ _ _ _ _ _ _ _ _ _ _ _ _ _ _]
              event Timeout {
                n85 = event-data() -> ()  [unwired: 1 in, 3 out]
              }
              event "Row Cropped data": Cursor Move; "Doppler Angle", "RF Average Window", "phase scale", "save spectorgrams": Value Change {
                n86 = event-data() -> ()  [unwired: 1 in, 4 out]
                n87 = stacked-sequence {
                  seq-local: [w243 _] -> [_ w493]
                  seq-local: ["save spectorgrams" _] -> [_ _]
                  seq-local: [w240 _] -> [_ w492]
                  seq-local: [w241 _] -> [_ w491]
                  seq-local: [w238 _] -> [_ w490]
                  tunnel: w232 -> [w251 _]
                  tunnel: w231 -> [w250 _]
                  tunnel: w230 -> [w249 _]
                  tunnel: w229 -> [w246 _]
                  tunnel: w228 -> [w245 _]
                  tunnel: w227 -> [w244 _]
                  tunnel: w226 -> [w237 w489]
                  tunnel: w225 -> [w236 _]
                  frame #0 {
                    n88 = case shown="False" "save spectorgrams" {
                      tunnel: [w254 w268] -> w248
                      tunnel: [w255 w270] -> w247
                      tunnel: w245 -> [_ w266]
                      tunnel: [w252 w264] -> w235
                      frame False {
                        n89 = property on="Row Cropped data" class="IntGraph (strict)"("Active Cursor"=0 ("Cursor.Cursor Index")) -> ("Cursor.Cursor X"=w259:dbl, "Cursor.Cursor Y"=w258:dbl)  [unwired: 2 in, 2 out]
                        n90 = Round Toward -Infinity(1:w259) -> (0:w256:dbl)
                        n91 = Round Toward -Infinity(1:w258) -> (0:w257:dbl)
                        n92 = Build Array(1) -> (w252:i32[])
                        n93 = Build Array(w256) -> (w255:dbl[])
                        n94 = Build Array(w257) -> (w254:dbl[])
                      }
                      frame True {
                        n95 = Array Size(array=w266) -> (size(s)=w265:i32[])
                        n96 = Index Array(array=w265) -> (element #2=w261:i32, element #3=w269:i32)  [unwired: 3 in, 1 out]
                        n97 = local write "save spectorgrams"(FALSE ("save spectorgrams")) -> ()
                        n98 = call-poly <vilib>:"Ramp Pattern.vi"("end"=w261, "delta"="Skip X") -> ("Ramp Pattern"=w270:dbl[])  [unwired: 7 in, 2 out]
                        n99 = call-poly <vilib>:"Ramp Pattern.vi"("end"=w269, "delta"="Skip Y") -> ("Ramp Pattern"=w268:dbl[])  [unwired: 7 in, 2 out]
                        n100 = Build Array("Skip X", "Skip Y") -> (w264:i32[])
                      }
                    }
                    n101 = for {
                      tunnel: w251 -> [w290]
                      tunnel: w250 -> [w289]
                      tunnel: w249 -> [w288]
                      tunnel: w245 -> [w287]
                      tunnel: w248 -> [w286]
                      tunnel: w247 -> [w285] mode=indexing
                      tunnel: w246 -> [w284]
                      tunnel: w244 -> [w282]
                      tunnel: "save spectorgrams" -> [w281]
                      shift-right: [w280] -> w243
                      shift-left: _ -> [w279]
                      tunnel: [w278] -> w241
                      tunnel: [w277] -> w240
                      tunnel: "Doppler Params" -> [w276]
                      shift-right: [w274] -> w238
                      shift-left: _ -> [w275]
                      tunnel: w237 -> [w273]
                      tunnel: w236 -> [w272]
                      tunnel: w235 -> [w271]
                      i -> [w283]
                      n102 = for {
                        N -> [w292]
                        tunnel: w290 -> [w312]
                        tunnel: w289 -> [w311]
                        tunnel: w288 -> [w310]
                        tunnel: w287 -> [w309]
                        tunnel: w286 -> [w308] mode=indexing
                        tunnel: w285 -> [w307]
                        tunnel: w284 -> [w306]
                        tunnel: w283 -> [w305]
                        tunnel: w282 -> [w303]
                        tunnel: w281 -> [w302]
                        shift-right: [w301] -> w280
                        shift-left: w279 -> [w300]
                        tunnel: [w299] -> w278
                        tunnel: [w298] -> w277
                        tunnel: w276 -> [w297]
                        shift-right: [w295] -> w274
                        shift-left: w275 -> [w296]
                        tunnel: w273 -> [w294]
                        tunnel: w272 -> [w293]
                        tunnel: w271 -> [w291]
                        i -> [w304]
                        n103 = stacked-sequence {
                          seq-local: [w323 _ _] -> [_ w373 _]
                          seq-local: [w322 _ _] -> [_ w370 _]
                          tunnel: w312 -> [w354 _ _]
                          tunnel: w311 -> [w353 _ _]
                          tunnel: w310 -> [w349 _ _]
                          tunnel: w309 -> [w315 _ _]
                          tunnel: w308 -> [w313 _ w396]
                          tunnel: w307 -> [w314 _ w397]
                          tunnel: w306 -> [w342 _ _]
                          tunnel: w305 -> [_ _ w394]
                          tunnel: w304 -> [_ _ w395]
                          tunnel: w303 -> [_ _ w403]
                          tunnel: w302 -> [_ _ w387]
                          tunnel: [_ _ w398] -> w301
                          tunnel: w300 -> [_ _ w393]
                          tunnel: [_ _ w392] -> w299
                          tunnel: [_ _ w391] -> w298
                          tunnel: w297 -> [w324 w374 _]
                          tunnel: w296 -> [_ _ w390]
                          tunnel: [_ _ w389] -> w295
                          tunnel: w294 -> [_ _ w388]
                          tunnel: w293 -> [_ _ w386]
                          tunnel: w292 -> [_ _ w385]
                          tunnel: w291 -> [_ _ w384]
                          tunnel: [w315 _ _] -> _
                          tunnel: [w314 _ _] -> _
                          tunnel: [w313 _ _] -> _
                          frame #0 {
                            n104 = Array Subset(array=w315, index (dim 1)=w314, length (dim 1)="RF Average Window", index (dim 2)=w313, length (dim 2)="RF Average Window") -> (w348:cdb[][][])  [unwired: 2 in]
                            n105 = Bundle By Name(cluster=w324, "SlowTime (Hz)"=w342) -> (w341:T2)
                            n106 = for {
                              tunnel: w348 -> [w366] mode=indexing
                              tunnel: [w365] -> w347 mode=indexing
                              workers-P: _ -> [_]
                              n107 = Add Array Elements(numeric array=w366) -> (sum=w365:cdb)
                            }
                            n108 = Multiply(x="RF Average Window", y="RF Average Window") -> (x*y=w346:i32)
                            n109 = Divide(x=w347, y=w346) -> (x/y=w345:cdb[])
                            n110 = Unbundle By Name(w324) -> ("FFT Length"=w356:i32)
                            n111 = call "HighPassFilterST.vi"("Doppler Params"=w341, "slow time"=w345) -> ("Filtered X"=w357:csg[])  [unwired: 7 in, 2 out]
                            n112 = local read "Doppler Angle"() -> (w351:dbl)
                            n113 = Build Array(w345, w357) -> (→"Slow time of red line":cdb[][])
                            n114 = local read "Thresholds"() -> (w343:T4)
                            n115 = call "Doppler_Spectra.vi"("Thresholds"=w343, "slow time"=w357, "Doppler Params"=w341, "Header In"=w353) -> ("PowerRaw"=→"PowerRaw":sgl[][], "phase (old Fd AC)"=w330:sgl[], "Total Power (dB)"=w333:sgl[], "Mag Dop Spec"=w317:dbl[][], "Spec P Ratio"=→"Spec ratio":sgl[])  [unwired: 2 in, 5 out]
                            "Dop Spec" <- w317
                            "Total Power" <- w333
                            n116 = Build Array(w330) -> (w352:sgl[][])
                            n117 = Add Array Elements(numeric array=w333) -> (sum=→"Sum Power":sgl)
                            n118 = call "DopplerScale.vi"("FFT Length"=w356, "Header In"=w353, "Index(F)/Fd"=w349, "PRF1/2"=w354, "Angle"=w351, "Velocity index in"=w352) -> ("output cluster"=w323:T10, "slow-time sampling"=→"Slow time\nsampling":dbl, "max doppler velocity cm/s"=w322:dbl, "Velocity Out"=w350:dbl[][])  [unwired: 2 in]
                            "max doppler\nV cm/s" <- w322
                            n119 = Multiply(x=w330, y="phase scale") -> (x*y=w329:dbl[])
                            n120 = call <vilib>:"Unwrap Phase.vi"("Phase"=w329) -> ("Unwrapped Phase"=w328:dbl[])  [unwired: 9 in, 1 out]
                            n121 = Index Array(array=w350) -> (element=w319:dbl[])  [unwired: 2 in]
                            "Velocity" <- w319
                            n122 = Array Size(array=w319) -> (size(s)=w340:i32)
                            n123 = expression code="x*2"("Clip") -> (w339:i32)
                            n124 = Divide(x=w328, y="phase scale") -> (x/y=w327:dbl[])
                            n125 = Subtract(x=w340, y=w339) -> (x-y=w338:i32)
                            n126 = Build Array(w330, w327) -> (→"phase":dbl[][])
                            n127 = Array Subset(array=w319, index="Clip", length=w338) -> (w337:dbl[])
                            n128 = call-poly <vilib>:"Mean.vi"("X"=w337) -> ("mean"=→"Vel Mean":dbl, "error"=→"error":i32)
                            n129 = case shown="False" "Lag Overlay off?" {
                              tunnel: w317 -> [w363 w364]
                              tunnel: w323 -> [w362 _]
                              tunnel: w319 -> [w361 _]
                              tunnel: [w360 w364] -> w320
                              frame False {
                                n130 = call "OverlayVelocity.vi"("output cluster"=w362, "Velocity Out"=w361, "Mag Dop Spec"=w363) -> ("Array"=w360:sgl[][])  [unwired: 8 in]
                              }
                              frame True {
                              }
                            }
                            n131 = Array Max & Min(array=w320) -> (max value=w321:dbl)  [unwired: 3 out]
                            n132 = Subtract(x=w320, y=w321) -> (x-y=→"Doppler Signal" →"Doppler Spec For Save":dbl[][])
                          }
                          frame #1 {
                            n133 = Unbundle By Name(w374) -> ("Window Increment"=w375:i32)
                            n134 = Unbundle By Name(w373) -> ("Y Scale Mult"=w368:dbl, "Y Scale offset"=w372:dbl, "X Scale Mult"=w376:dbl, "Dop F offset"=w378:dbl, "Dop interval"=w377:dbl)
                            n135 = Multiply(x=w376, y=w375) -> (x*y=w371:dbl)
                            n136 = Negate(x=w370) -> (-x=w369:dbl)
                            n137 = property on="Spectrogram at marker" class="IntGraph (strict)"("YScale.Multiplier"=w368, "YScale.Offset"=w372, "XScale.Multiplier"=w371, "YScale.Maximum"=w370, "YScale.Minimum"=w369) -> ()  [unwired: 2 in, 2 out]
                            n138 = property on="Doppler Signal" class="IntGraph (strict)"("YScale.Multiplier"=w368, "YScale.Offset"=w372, "XScale.Multiplier"=w371, "YScale.Maximum"=w370, "YScale.Minimum"=w369) -> ()  [unwired: 2 in, 2 out]
                            n139 = property on="Dop Spec" class="WFGraph (strict)"("XScale.Multiplier"=w377, "XScale.Offset"=w378) -> ()  [unwired: 2 in, 2 out]
                            n140 = case shown="True" "Lock scale" {
                              tunnel: w372 -> [w383 _]
                              tunnel: w371 -> [w382 _]
                              tunnel: w370 -> [w381 _]
                              tunnel: w369 -> [w380 _]
                              tunnel: w368 -> [w379 _]
                              frame False {
                                n141 = property on="Doppler Spec For Save" class="IntGraph (strict)"("YScale.Multiplier"=w379, "YScale.Offset"=w383, "XScale.Multiplier"=w382, "YScale.Maximum"=w381, "YScale.Minimum"=w380) -> ()  [unwired: 2 in, 2 out]
                              }
                              frame True {
                              }
                            }
                          }
                          frame #2 {
                            w401 = u32 1 ("Active Cursor")
                            n142 = Multiply(x=w385, y=w394) -> (x*y=w404:i32)
                            n143 = property on="Row Cropped data" class="IntGraph (strict)"("Active Cursor"=w401, "Cursor.Cursor X"=w397, "Cursor.Cursor Y"=w396) -> (error out=w400:errorcluster)  [unwired: 2 in, 1 out]
                            n144 = property on="Row Cropped data save" class="IntGraph (strict)"(error in=w400, "Active Cursor"=w401, "Cursor.Cursor X"=w397, "Cursor.Cursor Y"=w396) -> (error out=w399:errorcluster)  [unwired: 1 in, 1 out]
                            n145 = Add(x=w395, y=w404) -> (x+y=w402:i32)
                            n146 = case shown="True" w387 {
                              tunnel: w403 -> [_ w413]
                              tunnel: w402 -> [_ w423]
                              tunnel: w399 -> [_ _]
                              tunnel: [_ w439] -> w398
                              tunnel: w395 -> [_ w435]
                              tunnel: w394 -> [_ w436]
                              tunnel: w393 -> [_ w438]
                              tunnel: [_ w418] -> w391
                              tunnel: [_ w409] -> w392
                              tunnel: w390 -> [_ w433]
                              tunnel: [_ w432] -> w389
                              tunnel: w388 -> [_ w427]
                              tunnel: w386 -> [_ w419]
                              tunnel: w384 -> [_ w414]
                              frame False {
                              }
                              frame True {
                                w420 = TRUE
                                w430 = 90
                                (unwired) "SG_Summaries" ("string")
                                w444 = u32 16448250
                                w445 = 24 ("Image Depth")
                                # "Save dims to pick out imagin in VPI"
                                n147 = Strip Path(path=w413) -> (stripped path=w412:path, name=w452:string)
                                n148 = Match Pattern(string=w452, regular expression="_HeaderInfoRcv.txt" ("search string")) -> (before substring=w411:string)  [unwired: 1 in, 3 out]
                                n149 = Match Pattern(string=w411, regular expression="_HeaderInfoIQSum_G.txt" ("search string")) -> (before substring=w409:string)  [unwired: 1 in, 3 out]
                                n150 = Select(t="SG_" ("string"), s=TRUE, f="SG_" ("string")) -> (s? t:f=w405:string)
                                n151 = Concatenate Strings(w405, w409) -> (w426:string)
                                n152 = call "NumberFileName.vi"("String"=".jpg" ("string"), "Digits"=2, "File number"=w423, "file name"=w409) -> ("Numbered File"=w425:string)
                                n153 = call "NumberFileName.vi"("String"="BM.jpg" ("string"), "Digits"=2, "File number"=w423, "file name"=w409) -> ("Numbered File"=w441:string)
                                n154 = Build Array(w436, w435) -> (w434:i32[])
                                n155 = Concatenate Strings(w405, w425) -> (w424:string)
                                n156 = Concatenate Strings("SG_Dims_" ("string"), w409, ".txt" ("string")) -> (w415:string)
                                n157 = Build Path(base path=w412, name or relative path=w426) -> (appended path=w450:path)
                                n158 = call <vilib>:"Check if File or Folder Exists.vi"("path"=w450) -> ("file or folder exists?"=w446:bool, "dup path"=w449:path)  [unwired: 8 in, 1 out]
                                n159 = invoke on="Doppler Spec For Save" class="IntGraph (strict)" method="Get Image"("image depth"=w445, "bg color"=w444) -> ("image data"=w431:T11)  [unwired: 4 in, 5 out]
                                n160 = invoke on="Row Cropped data save" class="IntGraph (strict)" method="Get Image"("image depth"=w445, "bg color"=w444) -> ("image data"=w428:T11)  [unwired: 4 in, 5 out]
                                n161 = case shown="False" w446 {
                                tunnel: w449 -> [w487 w488]
                                tunnel: [w486 w488] -> w418
                                frame False {
                                n162 = Create Folder(path (use dialog)=w487) -> (created path=w486:path)  [unwired: 2 in, 2 out]
                                }
                                frame True {
                                }
                                }
                                n163 = case shown="True" w427 {
                                tunnel: [w462 w479] -> w439
                                tunnel: w438 -> [w462 w474]
                                tunnel: w434 -> [_ w467]
                                tunnel: w433 -> [w461 w466]
                                tunnel: [w461 w465] -> w432
                                tunnel: w431 -> [_ w464]
                                tunnel: w428 -> [_ w463]
                                frame False {
                                }
                                frame True {
                                # "Tile images into one image"
                                n164 = call <vilib>:"Unflatten Pixmap.vi"("image data"=w464) -> ("24-bit pixmap"=w478:u32[][])  [unwired: 4 in, 6 out]
                                n165 = call <vilib>:"Unflatten Pixmap.vi"("image data"=w463) -> ("24-bit pixmap"=w472:u32[][])  [unwired: 4 in, 6 out]
                                n166 = Array Size(array=w478) -> (size(s)=w477:i32[])
                                n167 = Array Size(array=w472) -> (size(s)=w471:i32[])
                                n168 = Reverse 1D Array(array=w477) -> (reversed array=w473:i32[])
                                n169 = Reverse 1D Array(array=w471) -> (reversed array=w468:i32[])
                                n170 = Multiply(x=w467, y=w473) -> (x*y=w476:i32[])
                                n171 = Multiply(x=w467, y=w468) -> (x*y=w470:i32[])
                                n172 = Array To Cluster(array=w476) -> (cluster=w475:cluster{"[0]":i32, "[1]":i32})
                                n173 = Array To Cluster(array=w470) -> (cluster=w469:cluster{"[0]":i32, "[1]":i32})
                                n174 = call-poly <vilib>:"Draw Unflattened Pixmap.vi"("picture"=w466, "top left point(0, 0)"=w469, "data (RGB format)"=w472) -> ("new picture"=w465:picture)  [unwired: 6 in]
                                n175 = call-poly <vilib>:"Draw Unflattened Pixmap.vi"("picture"=w474, "top left point(0, 0)"=w475, "data (RGB format)"=w478) -> ("new picture"=w479:picture)  [unwired: 6 in]
                                }
                                }
                                n176 = Build Path(base path=w418, name or relative path=w441) -> (appended path=w440:path)
                                n177 = Equal To 0?(x=w423) -> (x = 0?=w422:bool)
                                n178 = Build Path(base path=w418, name or relative path=w424) -> (appended path=w437:path)
                                n179 = And(x=w422, y=w420) -> (x .and. y?=w421:bool)
                                n180 = case shown="True" w421 {
                                tunnel: w419 -> [_ w460]
                                tunnel: w418 -> [_ w456]
                                tunnel: w415 -> [_ w455]
                                tunnel: w414 -> [_ w453]
                                frame False {
                                }
                                frame True {
                                n181 = Unbundle(w460) -> (w459:dbl, w458:dbl)  [unwired: 2 out]
                                n182 = Build Array (concatenate)(w459, w458, w453) -> (w457:dbl[])
                                n183 = Build Path(base path=w456, name or relative path=w455) -> (appended path=w454:path)
                                n184 = call-poly <vilib>:"Write Delimited Spreadsheet.vi"("file path (dialog if empty)"=w454, "1D data"=w457) -> ()  [unwired: 12 in, 2 out]
                                }
                                }
                                n185 = case shown="True" FALSE {
                                tunnel: w440 -> [_ w485]
                                tunnel: w428 -> [_ w484]
                                tunnel: w430 -> [_ w483]
                                frame False {
                                }
                                frame True {
                                n186 = call <vilib>:"Write JPEG File.vi"("quality (80)"=w483, "image data"=w484, "path to JPEG file"=w485) -> ()  [unwired: 7 in, 2 out]
                                }
                                }
                                n187 = case shown="True" w420 {
                                tunnel: w437 -> [_ w482]
                                tunnel: w431 -> [_ w480]
                                tunnel: w430 -> [_ w481]
                                frame False {
                                }
                                frame True {
                                n188 = call <vilib>:"Write JPEG File.vi"("quality (80)"=w481, "image data"=w480, "path to JPEG file"=w482) -> ()  [unwired: 7 in, 2 out]
                                }
                                }
                              }
                            }
                          }
                        }
                      }
                    }
                  }
                  frame #1 {
                    n189 = case shown="True" w489 {
                      tunnel: w493 -> [_ w505]
                      tunnel: w492 -> [_ w507]
                      tunnel: w491 -> [_ w494]
                      tunnel: w490 -> [_ w498]
                      frame False {
                      }
                      frame True {
                        w495 = cluster{"x":i16, "y":i16} {"x"=300, "y"=0} ("origin")
                        w496 = T12."User-specified Font" ("desired font(Application)")
                        w497 = T13 {"Font Name:"="Arial", "Size"=30, "Strikeout?"=FALSE, "Italic?"=FALSE, "Underline?"=FALSE, "Outline?"=FALSE, "Shadow?"=FALSE, "Bold?"=TRUE} ("[user-specified font]")
                        w506 = 90 ("quality (80)")
                        n190 = call <vilib>:"Draw Text at Point.vi"("BG color(transparent)"=u32 16448250, "[user-specified font]"=w497, "text color(black)"=u32 0, "desired font(Application)"=w496, "text"=w494, "origin"=w495, "picture"=w505) -> ("new picture"=w504:picture)  [unwired: 3 in, 1 out]
                        n191 = call <vilib>:"Draw Text at Point.vi"("BG color(transparent)"=u32 16448250, "[user-specified font]"=w497, "text color(black)"=u32 0, "desired font(Application)"=w496, "text"=w494, "origin"=w495, "picture"=w498) -> ("new picture"=w499:picture)  [unwired: 3 in, 1 out]
                        n192 = Concatenate Strings(w494, "SGAll.jpg" ("string")) -> (w515:string)
                        n193 = Concatenate Strings(w494, "BMAll.jpg" ("string")) -> (w509:string)
                        n194 = call <vilib>:"Picture to Pixmap.vi"("Background Color"=u32 16777215, "depth"=24, "picture"=w504) -> ("image data"=w519:T11)  [unwired: 7 in, 1 out]
                        n195 = Build Path(base path=w507, name or relative path=w515) -> (appended path=w514:path)
                        n196 = Build Path(base path=w507, name or relative path=w509) -> (appended path=w508:path)
                        n197 = call <vilib>:"Picture to Pixmap.vi"("Background Color"=u32 16777215, "depth"=24, "picture"=w499) -> ("image data"=w513:T11)  [unwired: 7 in, 1 out]
                        n198 = call <vilib>:"Write JPEG File.vi"("quality (80)"=w506, "image data"=w519, "path to JPEG file"=w514) -> ()  [unwired: 7 in, 2 out]
                        n199 = call <vilib>:"Write JPEG File.vi"("quality (80)"=w506, "image data"=w513, "path to JPEG file"=w508) -> ()  [unwired: 7 in, 2 out]
                      }
                    }
                  }
                }
              }
              event "Raw data": Cursor Release; "#y rf", "#x lines", "2D threshold", "Ref Place for 2S", "Save Motion": Value Change {
                # "This slows things down"
                n200 = event-data() -> ()  [unwired: 1 in, 4 out]
                n201 = property on="Raw data" class="IntGraph (strict)"("Active Cursor"=u32 2) -> ("Cursor.Cursor Position"=w533:T14)  [unwired: 2 in, 2 out]
                n202 = Unbundle By Name(w533) -> ("Cursor X"=w532:dbl, "Cursor Y"=w531:dbl)
                n203 = Unbundle By Name(w562) -> ("SlowTime (Hz)"=w561:dbl)
                n204 = Round Toward -Infinity(1:w532) -> (0:w526:dbl)
                n205 = Round Toward -Infinity(1:w531) -> ()  [unwired: 1 out]
                n206 = expression code="1/x"(w561) -> (w560:dbl)
                n207 = for {
                  tunnel: w521 -> [w573] mode=indexing
                  tunnel: [w571] -> w520 mode=indexing
                  n208 = Absolute Value(x=w573) -> (abs(x)=w572:dbl[][])
                  n209 = Array Max & Min(array=w572) -> (max index (indices)=w574:i32[])  [unwired: 3 out]
                  n210 = Index Array(array=w574) -> (element=w571:i32)  [unwired: 1 in]
                }
                "Waveform Graph" <- w520
                n211 = for {
                  tunnel: [w588] -> w522 mode=indexing if=w583
                  tunnel: w521 -> [w588] mode=indexing
                  tunnel: w560 -> [w586]
                  tunnel: "Divide down" -> [w585]
                  tunnel: [w584] -> w530 mode=indexing if=w583
                  i -> [w587]
                  n212 = Quotient & Remainder(x=w587, y=w585) -> (x-y*floor(x/y)=w589:i32)  [unwired: 1 out]
                  n213 = Compound Arithmetic op=MULTIPLY(w587, w586) -> (w584:dbl)
                  n214 = Equal To 0?(x=w589) -> (x = 0?=w583:bool)
                }
                n215 = Index Array(array=w521, index (dim 1)=w526) -> (element=w527:cdb[][])  [unwired: 2 in]
                n216 = Absolute Value(x=w527) -> (abs(x)=w529:dbl[][])
                n217 = expression code="20*log(x)"(w529) -> (w525:dbl[][])
                n218 = Array Max & Min(array=w525) -> (max value=w524:dbl)  [unwired: 3 out]
                n219 = Subtract(x=w525, y=w524) -> (x-y=→"M-mode x":dbl[][])
                n220 = Strip Path(path=w555) -> (name=w554:string)  [unwired: 1 out]
                n221 = Match Pattern(string=w554, regular expression="_" ("search string")) -> (before substring=w543:string, after substring=w552:string)  [unwired: 1 in, 2 out]
                n222 = Match Pattern(string=w552, regular expression="C" ("search string")) -> (before substring=w550:string, after substring=w538:string)  [unwired: 1 in, 2 out]
                n223 = Match Pattern(string=w538, regular expression="mS_" ("search string")) -> (after substring=w537:string)  [unwired: 1 in, 3 out]
                n224 = Search and Replace String(input string=w550, search string="p", replace string="." ("search string")) -> (result string=w548:string)  [unwired: 5 in, 3 out]
                n225 = Match Pattern(string=w537, regular expression="_He" ("search string")) -> (before substring=w535:string)  [unwired: 1 in, 3 out]
                n226 = Fract/Exp String To Number(string=w543) -> (number=w541:dbl)  [unwired: 3 in, 1 out]
                n227 = call "MotionTracker2DCorr.vi"("Ref frame for 2S"="Ref Place for 2S", "Cursor.Cursor Position"=w533, "#x lines"="#x lines", "#y rf"="#y rf", "RF In"=w522, "2D threshold"="2D threshold") -> ("Mean axial Disp"=w547:dbl[], "2D corr"=→"2D corr":dbl[][])  [unwired: 3 in, 1 out]
                n228 = Fract/Exp String To Number(string=w548) -> (number=w540:dbl)  [unwired: 3 in, 1 out]
                n229 = Fract/Exp String To Number(string=w535) -> (number=w534:dbl)  [unwired: 3 in, 1 out]
                n230 = Bundle(w530, "Mean axial Disp"=w547) -> (→"Simple Motion Tracker":cluster{dbl[], "Mean axial Disp":dbl[]})  [unwired: 1 in]
                n231 = Build Array (concatenate)(w540, w541, w534, w547) -> (w546:dbl[])
                n232 = Build Array (concatenate)(w540, w541, w534, w530) -> (w545:dbl[])
                n233 = case shown="0" w544 {
                  tunnel: [w577 w578] -> w557
                  tunnel: w546 -> [w576 w579]
                  tunnel: w545 -> [w575 _]
                  frame 0 {
                    n234 = Build Array(w575, w576) -> (w577:dbl[][])
                  }
                  frame 1, Default {
                    n235 = Build Array(w579) -> (w578:dbl[][])
                  }
                }
                n236 = case shown="False" "Save Motion" {
                  tunnel: w557 -> [_ w582]
                  tunnel: path "C:/Users/jketterling/Desktop/test.txt" ("file path (dialog if empty)") -> [_ w581]
                  frame False {
                  }
                  frame True {
                    n237 = call-poly <vilib>:"Write Delimited Spreadsheet.vi"("file path (dialog if empty)"=w581, "2D data"=w582, "append to file? (new file:F)"=TRUE) -> ()  [unwired: 11 in, 2 out]
                  }
                }
              }
              event "SaveSpectrogram": Value Change {
                n238 = event-data() -> ()  [unwired: 1 in, 6 out]
                n239 = local read "Doppler Signal"() -> (w595:dbl[][])
                n240 = property on="Doppler Signal" class="IntGraph (strict)" props=["YScale", "Multiplier", "YScale", "Offset", "XScale", "Multiplier", "YScale", "Maximum", "YScale", "Minimum"]() -> ("YScale.Multiplier"=w601:dbl, "YScale.Offset"=w605:dbl, "XScale.Multiplier"=w608:dbl, "YScale.Maximum"=w604:dbl)  [unwired: 2 in, 3 out]
                n241 = To Single Precision Float(number=w595) -> (single precision float=w596:sgl[][])
                n242 = expression code="10**(x/20)"(w596) -> (w594:sgl[][])
                n243 = Transpose 2D Array(2D array=w594) -> (transposed array=w603:sgl[][])
                n244 = Array Size(array=w594) -> (size(s)=w611:i32[])
                n245 = Reciprocal(x=w608) -> (1/x=w607:dbl)
                n246 = Index Array(array=w611) -> (element #1=w610:i32, element #2=w609:i32)  [unwired: 2 in]
                n247 = expression code="x*1000"(w607) -> (w602:dbl)
                n248 = expression code="x*10000"(w601) -> (w600:dbl)
                n249 = Bundle By Name(cluster=T1 {"header info"={"Header"="", "Head length"=0}, "A/D info"={"# rf points per line"=0, "# lines per scan"=0, "sample rate MHz"=0, "# A/D bits"=0, "# bytes per A/D"=0, "TGC Flag"=0, "A/D Type"=""}, "Tranducer Info"={"bandwidth"=0.0, "center freq"=0.0, "start freq"=0.0, "ID"=0}, "Scan Info"={"delay"=0.0, "pivot distance"=0.0, "sector scan angle"=0.0, "operator"="", "Scan Mode"="", "location"=""}, "Time/Date Info"={"date"="", "time"=""}, "RF Info"={"RF file name"="", "RF file att"="", "RF cal file name"="", "RF cal file att"=""}, "Patient Info"={"ID"="", "extended ID"="", "age"=0, "sex"="", "previously\nscanned"="", "PSA"=0.0, "LOS"=0, "Ethnicty 2"=0, "Race"=0}, "Tissue Type"={"organ"=0, "disease type"=0, "disease location"=0, "IQ_pts"=0, "RcvBuffer"=0, "RcvFrame"=0, "IQBuff"=0, "IQFrame"=0, "IQPage"=0}, "Votage scaling"={"Digitizer (dB)"=0.0, "Gain (dB)"=0.0, "Atten (dB)"=0.0}, "Comment"="", "Misc Info"={"avg num"=0, "c speed"=0, "Div By or SF zones"=0, "XMIT CHS"=0, "RCV CHS"=0, "Xmit angle"=0.0}, "Therapy Parameters"={"Theraputic Freq (MHz)"=0.0, "Time on (s)"=0.0, "Therapy amplitude (mV)"=0.0, "Lines Before"=0, "Lines After"=0}, "Scan Settings"={"Energy (uJ or V)"=0, "Damp (Ohm) or Fc"=0, "HP Filt (KHz)"=0, "LP Filt (MHz)"=0, "Gain (db)"=0, "prf (kHz)"=0.0, "Distance between\nscan lines (um)"=0, "Distance between\nscan planes (um)"=0, "Scan line gap (um)"=0.0, "Scan plane gap (um)"=0.0}, "Compression Parameters"={"F1 (MHz)"=0.0, "F2 (MHz)"=0.0, "% taper"=0.0, "duration"=0.0}, "Patient Info Xtra"={"First Name"="", "Last Name"="", "Notes"=""}, "ROI Box"=[]} ("Header In"), "A/D info.# rf points per line"=w610, "A/D info.# lines per scan"=w609, "A/D info.sample rate MHz"=w602, "Compression Parameters.F1 (MHz)"=w601, "Compression Parameters.F2 (MHz)"=w605, "Compression Parameters.% taper"=w604, "Scan Settings.Distance between\nscan lines (um)"=w600, "Misc Info.c speed"=i16 1000) -> (w612:T1)
                n250 = Strip Path(path=w597) -> (stripped path=w593:path, name=w592:string)
                n251 = Concatenate Strings("Spec" ("string"), w592) -> (w591:string)
                n252 = call "File Dialog"("start path"=w593, "default name"=w591) -> ("selected path"=w598:path)  [unwired: 10 in, 3 out]
                n253 = call "SaveDataSGLFast.vi"("Header In"=w612, "Save?"=TRUE, "Data Array"=w603, "File Name and Path"=w598) -> ()  [unwired: 7 in, 1 out]
              }
              event "Save M-mode": Value Change {
                # "Artificial Sampling rate"
                n254 = event-data() -> ()  [unwired: 1 in, 6 out]
                n255 = property on="Row Cropped data" class="IntGraph (strict)"("Active Cursor"=0 ("Cursor.Cursor Index")) -> ("Cursor.Cursor X"=w636:dbl, "Cursor.Cursor Y"=w635:dbl)  [unwired: 2 in, 2 out]
                n256 = Round Toward -Infinity(1:w636) -> (0:w633:dbl)
                n257 = Round Toward -Infinity(1:w635) -> (0:w632:dbl)
                n258 = Unbundle By Name(w621) -> ("Scan Settings.Distance between\nscan lines (um)"=w619:u16)
                n259 = Index Array(array=w624, index (dim 1)=w633) -> (element=w627:cdb[][])  [unwired: 2 in]
                n260 = Index Array(array=w624, index (dim 2)=w632) -> ()  [unwired: 2 in, 1 out]
                n261 = local read "Slow time\nsampling"() -> (w623:sgl)
                n262 = Array Size(array=w627) -> (size(s)=w626:i32[])
                n263 = expression code="1E6/x"(w623) -> (w622:sgl)
                n264 = Strip Path(path=w641) -> (stripped path=w640:path, name=w639:string)
                n265 = Reciprocal(x=w619) -> (1/x=w618:dbl)
                n266 = Index Array(array=w626) -> (element=w625:i32)  [unwired: 1 in]
                n267 = expression code="X*1000"(w618) -> (w617:dbl)
                n268 = Bundle By Name(cluster=w621, "A/D info.# lines per scan"=w625, "A/D info.sample rate MHz"=w617, "Scan Settings.Distance between\nscan lines (um)"=w622, "Misc Info.c speed"=i16 2000) -> (w644:T1)
                n269 = Concatenate Strings("MMode" ("string"), w639) -> (w631:string)
                n270 = Search and Replace String(input string=w631, search string="txt", replace string="eye" ("replace string (\"\")")) -> (result string=w628:string)  [unwired: 5 in, 3 out]
                n271 = call "File Dialog2"("start path"=w640, "default name"=w628) -> ("selected path"=w642:path)  [unwired: 10 in, 3 out]
                n272 = call "SaveDataSGLFast.vi"("Header In"=w644, "Save?"=TRUE, "Data Array"=w627, "File Name and Path"=w642) -> ()  [unwired: 7 in, 1 out]
              }
              event "Save Vels": Value Change {
                w658 = "file name\nnote\ntime (ms)\nvel cursor\nvel lagone\nMax Vel\nBPM\npixel x\npixel y\nfilter tap\nwindow length\nwindow incrent\nfilter start\nfilter cutoff\nFFT length\nslow time (HZ)\nRF AVG"
                w654 = path "F:/DopplerVels.txt" ("file path (dialog if empty)")
                n273 = event-data() -> ()  [unwired: 1 in, 1 out]
                n274 = property on="Doppler Signal" class="IntGraph (strict)"("Active Cursor"=u32 2) -> ("YScale.Maximum"=w647:dbl, "Cursor.Cursor Position"=w684:T14, "XScale.Multiplier"=w678:dbl)  [unwired: 2 in, 2 out]
                n275 = property on="Row Cropped data" class="IntGraph (strict)"("Active Cursor"=u32 0) -> ("Cursor.Cursor Position"=w670:T14)  [unwired: 2 in, 2 out]
                n276 = Unbundle By Name(w684) -> ("Cursor X"=w680:dbl, "Cursor Y"=w649:dbl)
                n277 = Unbundle By Name(w670) -> ("Cursor X"=w669:dbl, "Cursor Y"=w668:dbl)
                n278 = Compound Arithmetic op=ADD(w647, w647, w649) -> (w648:dbl)
                n279 = Divide(x=w680, y=w678) -> (x/y=w679:dbl)
                n280 = Unbundle By Name(w667) -> ("Dopp Filter Order"=w666:i32, "Window length"=w665:i32, "Window Increment"=w664:i32, "Start f"=w663:dbl, "lDoppler cutouff"=w662:dbl, "FFT Length"=w661:i32, "SlowTime (Hz)"=w660:dbl)
                n281 = local read "Velocity"() -> (w683:dbl[])
                n282 = local read "BPM"() -> (w681:i32)
                n283 = local read "RF Average Window"() -> (w646:i32)
                n284 = Select(t=w648, s="Alias Correct", f=w649) -> (s? t:f=w650:dbl)
                n285 = Index Array(array=w683, index=w679) -> (element=w682:dbl)
                n286 = Strip Path(path=w672) -> (name=w676:string)  [unwired: 1 out]
                n287 = Build Array(w680, w650, w682, w647, w681, w669, w668, w666, w665, w664, w663, w662, w661, w660, w646) -> (w674:dbl[])
                n288 = Number To Fractional String(number=w674, precision (6)=i16 2) -> (F-format string=w677:string[])  [unwired: 2 in]
                n289 = Spreadsheet String To Array(format string="%s", spreadsheet string=w658, array type (2D Dbl)=w658) -> (array=w656:string[][])  [unwired: 1 in]
                n290 = Index Array(array=w656, index (col)=0 ("disabled index (col)")) -> (element=w653:string[])  [unwired: 1 in]
                n291 = Build Array (concatenate)(w676, "Note", w677) -> (w652:string[])
                n292 = call <vilib>:"Check if File or Folder Exists.vi"("path"=w654) -> ("file or folder exists?"=w655:bool)  [unwired: 8 in, 2 out]
                n293 = stacked-sequence {
                  tunnel: w652 -> [_ w697]
                  tunnel: w655 -> [w691 _]
                  tunnel: w654 -> [w690 w696]
                  tunnel: w653 -> [w689 _]
                  frame #0 {
                    n294 = case shown="False" w691 {
                      tunnel: w690 -> [w693 _]
                      tunnel: w689 -> [w692 _]
                      frame False {
                        n295 = call-poly <vilib>:"Write Delimited Spreadsheet.vi"("file path (dialog if empty)"=w693, "1D data"=w692, "append to file? (new file:F)"=TRUE, "transpose? (no:F)"=FALSE) -> ()  [unwired: 10 in, 2 out]
                      }
                      frame True {
                      }
                    }
                  }
                  frame #1 {
                    n296 = call-poly <vilib>:"Write Delimited Spreadsheet.vi"("file path (dialog if empty)"=w696, "1D data"=w697, "append to file? (new file:F)"=TRUE, "transpose? (no:F)"=FALSE) -> ()  [unwired: 10 in, 2 out]
                  }
                }
              }
              event "Doppler Signal": Cursor Move; "Cycles": Value Change {
                n297 = event-data() -> ()  [unwired: 1 in, 4 out]
                n298 = property on="Doppler Signal" class="IntGraph (strict)"("Active Cursor"=u32 0, "Active Cursor"=u32 1, "Active Cursor"=u32 2) -> ("Cursor.Cursor X"=w729:dbl, "Cursor.Cursor X"=w728:dbl, "Cursor.Cursor X"=w700:dbl, "XScale.Multiplier"=w707:dbl)  [unwired: 2 in, 2 out]
                n299 = Unbundle By Name(w706) -> ("Window Increment"=w703:i32)
                n300 = local read "Velocity"() -> (w704:dbl[])
                n301 = Subtract(x=w729, y=w728) -> (x-y=w727:dbl)
                n302 = call-poly <vilib>:"Quick Scale.vi"("X"=w704) -> ("Y[i]=X[i]/Max|X|"=w717:dbl[])  [unwired: 2 out]
                n303 = Negate(x=w717) -> (-x=w716:dbl[])
                n304 = Unbundle By Name(w706) -> ("SlowTime (Hz)"=w722:dbl, "Window Increment"=w721:i32)
                n305 = Build Array(w717, w716) -> (w715:dbl[][])
                n306 = Divide(x=w700, y=w707) -> (x/y=w701:dbl)
                n307 = expression code="60*1000/abs(x)"(w727) -> (w725:dbl)
                n308 = Multiply(x=w701, y=w703) -> (x*y=w702:dbl)
                n309 = Reciprocal(x=w721) -> (1/x=w720:dbl)
                n310 = for {
                  tunnel: "width" -> [w749]
                  tunnel: "threshold" -> [w748]
                  tunnel: w722 -> [w742]
                  tunnel: w720 -> [w740]
                  tunnel: [w739] -> w713 mode=indexing
                  tunnel: w715 -> [w738] mode=indexing
                  tunnel: [w737] -> w714 mode=indexing
                  n311 = call <vilib>:"Peak Detector.vi"("width"=w749, "threshold"=w748, "X"=w738) -> ("Locations"=w747:dbl[], "# found"=w737:i32)  [unwired: 4 in, 3 out]
                  n312 = Decrement(x=w737) -> (x-1=w741:i32)
                  n313 = Index Array(array=w747, index #2=w741) -> (element #1=w745:dbl, element #2=w744:dbl)  [unwired: 1 in]
                  n314 = Subtract(x=w745, y=w744) -> (x-y=w746:dbl)
                  n315 = expression code="60/abs(x)"(w746) -> (w743:dbl)
                  n316 = Compound Arithmetic op=MULTIPLY(w741, w743, w742, w740) -> (w739:dbl)
                }
                "# found" <- w714
                "BPM auto" <- w713
                n317 = property on="image to display" class="DigNum (strict)"("Val(Sgnl)"=w702) -> ()  [unwired: 2 in, 2 out]
                n318 = Multiply(x=w725, y="Cycles") -> (x*y=w711:dbl)
                n319 = expression code="x/60"(w711) -> (w710:dbl)
                n320 = Index Array(array=w704, index=w701) -> (element=→"LagOne":dbl)
                n321 = case shown="False" "Freeze BPM" {
                  tunnel: w711 -> [w736 _]
                  tunnel: w710 -> [w735 _]
                  frame False {
                    "BPM" <- w736
                    "BPS" <- w735
                  }
                  frame True {
                  }
                }
                n322 = Build Array (concatenate)(w714, w713) -> (w712:dbl[])
                n323 = case shown="True" w718 {
                  tunnel: w719 -> [_ w761]
                  tunnel: w712 -> [_ w759]
                  frame False {
                  }
                  frame True {
                    n324 = Strip Path(path=w761) -> (stripped path=w762:path, name=w764:string)
                    n325 = Strip Path(path=w762) -> (stripped path=w753:path)  [unwired: 1 out]
                    n326 = Match Pattern(string=w764, regular expression="IQSum" ("search string")) -> (before substring=w758:string)  [unwired: 1 in, 3 out]
                    n327 = Strip Path(path=w753) -> (stripped path=w752:path, name=w750:string)
                    n328 = Strip Path(path=w752) -> (stripped path=w751:path)  [unwired: 1 out]
                    n329 = Number To Decimal String(number=w759) -> (decimal integer string=w754:string[])  [unwired: 1 in]
                    n330 = Build Array (concatenate)(w750, w758, w754) -> (w757:string[])
                    n331 = Build Path(base path=w751, name or relative path="BPM_Summary.Txt" ("string")) -> (appended path=w755:path)
                    n332 = call-poly <vilib>:"Write Delimited Spreadsheet.vi"("file path (dialog if empty)"=w755, "1D data"=w757, "append to file? (new file:F)"=TRUE) -> ()  [unwired: 11 in, 2 out]
                  }
                }
              }
              event "Total Power": Cursor Move {
                w765 = 2 ("left rank")
                n333 = event-data() -> ("CursLoc"=w770:cluster{"X":dbl, "Y":dbl})  [unwired: 1 in, 1 out]
                n334 = Unbundle By Name(w770) -> ("X"=w768:dbl)
                n335 = local read "Dop Spec"() -> (w769:dbl[][])
                n336 = Index Array(array=w769, index (row)=w768) -> (element=w767:dbl[])  [unwired: 1 in]
                n337 = call <vilib>:"Median Filter.vi"("right rank"=w765, "left rank"=w765, "X"=w767) -> ("Filtered X"=→"Spectrum":dbl[])  [unwired: 7 in, 1 out]
              }
              event "image to display", "Log RF?": Value Change {
                n338 = event-data() -> ()  [unwired: 1 in, 6 out]
                n339 = local read "image to display"() -> (w775:i32)
                n340 = local read "HIgh pass Filtered X"() -> (w782:sgl[][][])
                n341 = local read "Cross Correlate"() -> (w787:sgl[][][])
                n342 = Index Array(array=w782, index (dim 0)=w775) -> (element=w783:sgl[][])  [unwired: 2 in]
                n343 = Index Array(array=w788, index (dim 0)=w775) -> (element=w786:cdb[][])  [unwired: 2 in]
                n344 = Absolute Value(x=w783) -> (abs(x)=w777:sgl[][])
                "Raw High pass filtered" <- w777
                n345 = Index Array(array=w787, index (dim 0)=w775) -> (element=w780:sgl[][])  [unwired: 2 in]
                "Cross Correlate" <- w780
                n346 = Absolute Value(x=w786) -> (abs(x)=w785:dbl[][])
                n347 = expression code="20*log(x)"(w777) -> (w779:sgl[][])
                "High pass Filtered log" <- w779
                n348 = case shown="True" "Log RF?" {
                  tunnel: w785 -> [w790 w794]
                  tunnel: [w790 w792] -> w774
                  frame False {
                  }
                  frame True {
                    n349 = expression code="20*log(x)"(w794) -> (w793:dbl[][])
                    n350 = local read "max value"() -> (w791:sgl)
                    n351 = Array Max & Min(array=w793) -> ()  [unwired: 4 out]
                    n352 = Subtract(x=w793, y=w791) -> (x-y=w792:dbl[][])
                  }
                }
                "Row Cropped data" <- w774
                "Row Cropped data save" <- w774
                n353 = Array Max & Min(array=w779) -> (max value=w784:sgl)  [unwired: 3 out]
                n354 = Subtract(x=w779, y=w784) -> ()  [unwired: 1 out]
                n355 = call-poly <vilib>:"Plot Helper.vi"("z matrix"=w780) -> ("3D Plot lvclass Array out"=→"3D Surface":refnum<class "3D Plot Datatype.lvclass">[])  [unwired: 5 in, 5 out]
              }
              event "Calc Spec Peaks": Value Change {
                (unwired) 0 ("index")
                n356 = event-data() -> ()  [unwired: 1 in, 1 out]
                n357 = local read "ms between frames"() -> (w810:u32)
                n358 = local read "RF Average Window"() -> (w797:i32)
                n359 = property on="ms between frames" class="DigNum (strict)"("Val(Sgnl)"=w810) -> ()  [unwired: 2 in, 2 out]
                n360 = Array Subset(array=path[] [], length=4000) -> (w799:path[])  [unwired: 1 in]
                n361 = case shown="False" "Queue processing" {
                  tunnel: [w834 w998] -> w809
                  tunnel: w808 -> [w833 w988]
                  tunnel: w806 -> [w811 w984]
                  tunnel: w796 -> [w816 w987]
                  tunnel: w799 -> [w819 _]
                  tunnel: w805 -> [w828 w989]
                  tunnel: w798 -> [w825 w986]
                  tunnel: w804 -> [w812 w991]
                  tunnel: w803 -> [_ _]
                  tunnel: [w824 w996] -> w801
                  tunnel: w800 -> [w813 w992]
                  tunnel: w797 -> [_ w983]
                  frame True {
                    # "Build up set of data"
                    # "This loop is limited by read time of files. Local files will process faster than network"
                    n362 = Array Size(array=w819) -> (size(s)=w826:i32)
                    n363 = Obtain Queue(max queue size (-1, unlimited)=200, name (unnamed)="Dopp", element data type=csg[][] [] ("subarray")) -> (queue out=w830:refnum<queue>)  [unwired: 2 in, 2 out]
                    n364 = Array Size(array=w819) -> (size(s)=w818:i32)
                    n365 = for {
                      tunnel: w830 -> [w982]
                      tunnel: w811 -> [w981] mode=indexing
                      n366 = Enqueue Element(queue=w982, element=w981) -> ()  [unwired: 2 in, 3 out]
                    }
                    n367 = Obtain Queue(max queue size (-1, unlimited)=3, name (unnamed)="Saves", element data type=T6 {"subarray"=[], "Slow Time Pt"=0, "Line#"=0}) -> (queue out=w815:refnum<queue>)  [unwired: 2 in, 2 out]
                    n368 = while {
                      tunnel: [w858] -> w834 mode=concatenating
                      tunnel: w833 -> [w868]
                      tunnel: w830 -> [w856]
                      shift-right: [w871] -> _
                      shift-left: _ -> [w869]
                      tunnel: w816 -> [w850]
                      tunnel: w828 -> [w867]
                      shift-right: [w857] -> _
                      shift-left: FALSE ("timed out?") -> [w852]
                      tunnel: w826 -> [w863]
                      tunnel: w825 -> [w862]
                      tunnel: w812 -> [w861]
                      tunnel: [w859] -> w824 mode=concatenating
                      tunnel: [w856] -> w823
                      shift-right: [w855] -> _
                      shift-left: 0 ("max queue size (-1, unlimited)") -> [w854]
                      tunnel: w815 -> [w853]
                      tunnel: w813 -> [w851]
                      i -> [w870]
                      stop <- w852 stop-if-true
                      n369 = case shown="1, Default" w870 {
                        tunnel: [_ w912] -> w864
                        tunnel: w868 -> [_ w911]
                        tunnel: w856 -> [w894 w909]
                        tunnel: [w893 w908] -> w871
                        tunnel: w869 -> [_ w910]
                        tunnel: [FALSE ("timed out?") w907] -> w857
                        tunnel: w850 -> [w892 w906]
                        tunnel: [_ w905] -> w865
                        tunnel: w863 -> [w885 w902]
                        tunnel: w862 -> [_ w904]
                        tunnel: [_ w903] -> w860
                        tunnel: [_ w900] -> w855
                        tunnel: w854 -> [_ w901]
                        tunnel: w853 -> [_ w899]
                        tunnel: w852 -> [_ w898]
                        frame 0 {
                          # "Generate initial set of window length slow time"
                          n370 = Unbundle By Name(w892) -> ("Window Increment"=w890:i32, "Window length"=w888:i32)
                          n371 = Multiply(x=8, y=w890) -> (x*y=w889:i32)
                          n372 = Add(x=w889, y=w888) -> (x+y=w884:i32)
                          n373 = Max & Min(x=w885, y=w884) -> (min(x,y)=w883:i32)  [unwired: 1 out]
                          n374 = for {
                            N: w883 -> [_]
                            tunnel: w894 -> [w897]
                            tunnel: [w896] -> w893 mode=indexing
                            tunnel: 1000 ("x") -> [w895]
                            n375 = Dequeue Element(queue=w897, timeout in ms (-1)=w895) -> (element=w896:csg[][])  [unwired: 1 in, 3 out]
                          }
                        }
                        frame 1, Default {
                          n376 = stacked-sequence {
                            seq-local: [w916 _ _] -> [_ w950 w956]
                            tunnel: [w925 _ _] -> w912
                            tunnel: w911 -> [w918 _ _]
                            tunnel: w910 -> [w917 _ w959]
                            tunnel: w909 -> [_ _ w960]
                            tunnel: [_ _ w958] -> w908
                            tunnel: [_ _ w955] -> w907
                            tunnel: w906 -> [w921 _ w957]
                            tunnel: [_ w950 _] -> w905
                            tunnel: w904 -> [w920 _ _]
                            tunnel: [w919 _ _] -> w903
                            tunnel: w902 -> [_ _ _]
                            tunnel: [_ w952 _] -> w900
                            tunnel: w901 -> [w915 w951 _]
                            tunnel: w899 -> [w913 _ w953]
                            tunnel: w898 -> [_ _ w954]
                            frame #0 {
                              n377 = Array Size(array=w917) -> (size(s)=w924:i32[])
                              n378 = Index Array(array=w924, index=1) -> (element=w914:i32)
                              n379 = Index Array(array=w924, index=2) -> ()  [unwired: 1 out]
                              n380 = for {
                                N: w914 -> [_]
                                tunnel: [w939] -> w925 mode=indexing
                                tunnel: w917 -> [w938]
                                tunnel: w918 -> [w934]
                                tunnel: w921 -> [w931]
                                tunnel: [w937] -> w916
                                tunnel: w920 -> [w936]
                                tunnel: [w933] -> w919 mode=indexing
                                tunnel: w915 -> [w929]
                                tunnel: w913 -> [w926]
                                i -> [w928]
                                n381 = Index Array(array=w938, index (dim 1)=w928) -> (element=w932:csg[][])  [unwired: 2 in]
                                n382 = Transpose 2D Array(2D array=w932) -> (transposed array=w935:csg[][])
                                n383 = for {
                                tunnel: [w941] -> w939 mode=indexing
                                tunnel: w934 -> [w940]
                                tunnel: w931 -> [w946]
                                tunnel: w935 -> [w942] mode=indexing
                                workers-P: _ -> [_]
                                tunnel: [w949] -> w937
                                tunnel: w936 -> [w945]
                                tunnel: [w948] -> w933 mode=indexing
                                tunnel: [w943] -> w930 mode=indexing
                                # "process for slow time dopper"
                                n384 = call "HighPassFilterST.vi"("Doppler Params"=w946, "slow time"=w942) -> ("Filtered X"=w947:csg[])  [unwired: 7 in, 2 out]
                                n385 = call "Doppler_Spectra.vi"("Thresholds"=w945, "slow time"=w947, "Doppler Params"=w946, "Header In"=w940) -> ("Mean Power"=w948:sgl[], "phase (old Fd AC)"=w941:sgl[])  [unwired: 2 in, 8 out]
                                n386 = call "Doppler_Spectra.vi"("Thresholds"=w945, "slow time"=w942, "Doppler Params"=w946, "Header In"=w940) -> ("Mag Dop Spec"=w944:dbl[][])  [unwired: 2 in, 9 out]
                                n387 = To Byte Integer(number=w944) -> (8bit integer=w943:i8[][])
                                n388 = Array Size(array=w941) -> (size(s)=w949:i32)
                                }
                                n389 = Bundle(w930, "max queue size (-1, unlimited)"=w929, w928) -> (w927:T15)  [unwired: 1 in]
                                n390 = Enqueue Element(queue=w926, element=w927) -> ()  [unwired: 2 in, 3 out]
                              }
                            }
                            frame #1 {
                              n391 = Add(x=w950, y=w951) -> (x+y=w952:i32)
                            }
                            frame #2 {
                              n392 = case shown="False" w954 {
                                tunnel: w960 -> [w971 _]
                                tunnel: w959 -> [w969 w976]
                                tunnel: [w966 w976] -> w958
                                tunnel: w957 -> [w965 _]
                                tunnel: w956 -> [w964 _]
                                tunnel: [w961 _] -> w955
                                tunnel: w953 -> [_ w977]
                                frame False {
                                # "Rotate to"
                                n393 = Unbundle By Name(w965) -> ("Window Increment"=w963:i32)
                                n394 = Multiply(x=w964, y=w963) -> (x*y=w962:i32)
                                n395 = Delete From Array(array=w969, length=w962, index (dim 0)=0 ("index (page)")) -> (array with subset deleted=w968:csg[][][])  [unwired: 2 in, 1 out]
                                n396 = for {
                                N: w962 -> [_]
                                tunnel: w971 -> [w975]
                                tunnel: [w974] -> w967 mode=indexing
                                tunnel: [w972] -> w961
                                stop <- w972 stop-if-true
                                n397 = Dequeue Element(queue=w975, timeout in ms (-1)=1000) -> (element=w974:csg[][], timed out?=w972:bool)  [unwired: 1 in, 2 out]
                                }
                                n398 = Build Array (concatenate)(w968, w967) -> (w966:csg[][][])
                                }
                                frame True {
                                w979 = -1
                                n399 = Bundle(i8[][][] [], w979, w979) -> (w978:cluster{i8[][][], i32, i32})  [unwired: 1 in]
                                n400 = Enqueue Element(queue=w977, element=w978) -> ()  [unwired: 2 in, 3 out]
                                }
                              }
                            }
                          }
                        }
                      }
                      n401 = Unbundle By Name(w850) -> ("FFT Length"=w849:i32)
                      n402 = for {
                        N: w865 -> [_]
                        tunnel: w868 -> [w882]
                        tunnel: w867 -> [w881]
                        tunnel: [w872] -> w866
                        tunnel: w864 -> [w880]
                        tunnel: [w872] -> w858 mode=indexing
                        tunnel: w861 -> [w878]
                        tunnel: w860 -> [w877]
                        tunnel: [w875] -> w859 mode=indexing
                        tunnel: w851 -> [w874]
                        tunnel: w849 -> [w873]
                        i -> [w876]
                        n403 = Index Array(array=w877, index (dim 2)=w876) -> (element=w875:sgl[][])  [unwired: 2 in]
                        n404 = Index Array(array=w880, index (dim 2)=w876) -> (element=w879:sgl[][])  [unwired: 2 in]
                        n405 = call "DopplerScale.vi"("FFT Length"=w873, "Header In"=w882, "Index(F)/Fd"=w878, "PRF1/2"=w874, "Angle"=w881, "Velocity index in"=w879) -> ("Velocity Out"=w872:dbl[][])  [unwired: 2 in, 3 out]
                      }
                      n406 = local write "Peak V"(w866) -> ()
                    }
                    n407 = while {
                      tunnel: w815 -> [w841]
                      tunnel: w818 -> [w842]
                      tunnel: w816 -> [w840]
                      tunnel: [w839] -> w814
                      stop <- w836 stop-if-true
                      n408 = Dequeue Element(queue=w841) -> (queue out=w839:refnum<queue>, element=w838:T6)  [unwired: 2 in, 2 out]
                      n409 = Unbundle(w838) -> ("Slow Time Pt"=w835:i32)  [unwired: 2 out]
                      n410 = Equal?(x=-1, y=w835) -> (x = y?=w836:bool)
                      n411 = case shown="0, Default" w835 {
                        tunnel: w842 -> [w848 _]
                        tunnel: w838 -> [w847 _]
                        tunnel: w840 -> [w843 _]
                        frame 0, Default {
                          n412 = Unbundle(w847) -> ("subarray"=w846:i8[][][], "Slow Time Pt"=w845:i32, "Line#"=w844:i32)
                          n413 = call "WriteSpectrograms.vi"("Array"=w846, "Doppler Params"=w843, "row #"=w844, "Slow Time Pt Mark"=w845, "Total length"=w848) -> ()  [unwired: 7 in]
                        }
                        frame -1 {
                        }
                      }
                    }
                    n414 = Release Queue(queue=w823) -> ()  [unwired: 2 in, 3 out]
                    n415 = Release Queue(queue=w814) -> ()  [unwired: 2 in, 3 out]
                  }
                  frame False {
                    n416 = Array Size(array=w984) -> (size(s)=w994:i32[])
                    n417 = Index Array(array=w994, index=2) -> ()  [unwired: 1 out]
                    n418 = Index Array(array=w994, index=1) -> (element=w993:i32)
                    "Sets" <- w993
                    n419 = Unbundle By Name(w987) -> ("FFT Length"=w990:i32)
                    n420 = for {
                      N: w993 -> [_]
                      tunnel: [w1010] -> w1000 mode=indexing
                      tunnel: w984 -> [w1017]
                      tunnel: w988 -> [w1015]
                      tunnel: w987 -> [w1021]
                      tunnel: w986 -> [w1019]
                      tunnel: [w1018] -> w997 mode=indexing
                      tunnel: w992 -> [w1014]
                      tunnel: w991 -> [w1013]
                      tunnel: w990 -> [w1012]
                      tunnel: w989 -> [w1011]
                      tunnel: w983 -> [w1008]
                      i -> [w1020]
                      n421 = case shown="0, Default" w1008 {
                        selector: w1008 -> [w1022 _]
                        tunnel: w1020 -> [w1023 w1029]
                        tunnel: [w1024 w1026] -> w1009
                        tunnel: w1017 -> [w1025 w1028]
                        frame 0, Default {
                          n422 = call "SloweTimeAverage.vi"("index"=w1023, "Filtered Out"=w1025, "Average"=w1022) -> ("Slow Average"=w1024:csg[][])  [unwired: 8 in]
                        }
                        frame 1 {
                          n423 = Index Array(array=w1028, index (dim 1)=w1029) -> (element=w1027:cdb[][])  [unwired: 2 in]
                          n424 = Transpose 2D Array(2D array=w1027) -> (transposed array=w1026:cdb[][])
                        }
                      }
                      n425 = for {
                        tunnel: [w1032] -> w1016 mode=indexing
                        tunnel: w1009 -> [w1033] mode=indexing
                        tunnel: w1015 -> [w1036]
                        tunnel: w1021 -> [w1037]
                        workers-P: _ -> [_]
                        tunnel: w1019 -> [w1031]
                        tunnel: [w1034] -> w1018 mode=indexing
                        n426 = call "HighPassFilterST.vi"("init/cont (init:F)"=FALSE, "Doppler Params"=w1037, "slow time"=w1033) -> ("Filtered X"=w1030:csg[])  [unwired: 6 in, 2 out]
                        n427 = call "Doppler_Spectra.vi"("Thresholds"=w1031, "slow time"=w1030, "Doppler Params"=w1037, "Header In"=w1036) -> ("Mean Power"=w1034:sgl[], "phase (old Fd AC)"=w1032:sgl[])  [unwired: 2 in, 8 out]
                      }
                      n428 = call "DopplerScale.vi"("FFT Length"=w1012, "Header In"=w1015, "Index(F)/Fd"=w1013, "PRF1/2"=w1014, "Angle"=w1011, "Velocity index in"=w1016) -> ("Velocity Out"=w1010:dbl[][])  [unwired: 2 in, 3 out]
                      "Current" <- w1020
                    }
                    n429 = Array Size(array=w1000) -> (size(s)=w1002:i32[])
                    n430 = Index Array(array=w1002, index=2) -> (element=w999:i32)
                    n431 = for {
                      N: w999 -> [_]
                      tunnel: w1000 -> [w1007]
                      tunnel: [w1006] -> w998 mode=indexing
                      tunnel: w997 -> [w1005]
                      tunnel: [w1003] -> w996 mode=indexing
                      i -> [w1004]
                      n432 = Index Array(array=w1005, index (dim 2)=w1004) -> (element=w1003:sgl[][])  [unwired: 2 in]
                      n433 = Index Array(array=w1007, index (dim 2)=w1004) -> (element=w1006:dbl[][])  [unwired: 2 in]
                    }
                  }
                }
              }
              event "Overlay": Cursor Move; "Spectrogram average": Value Change {
                # "Take an avergag of all slow time estimates in window marked by cursors"
                n434 = event-data() -> ()  [unwired: 1 in, 2 out]
                n435 = Unbundle By Name(w1038) -> ("FFT Length"=w1041:i32)
                n436 = Array Size(array=w1064) -> (size(s)=w1078:i32[])
                n437 = Index Array(array=w1078, index=0) -> (element=w1075:i32)
                n438 = local read "Smoothed Data"() -> (w1061:dbl[][][])
                n439 = property on="Overlay" class="IntGraph (strict)"("Active Cursor"=u32 0, "Active Cursor"=u32 1) -> ("Cursor.Cursor X"=w1060:dbl, "Cursor.Cursor Y"=w1059:dbl, "Cursor.Cursor X"=w1081:dbl, "Cursor.Cursor Y"=w1082:dbl)  [unwired: 2 in, 2 out]
                n440 = local read "Queue processing"() -> (w1055:bool)
                n441 = Subtract(x=w1081, y=w1060) -> (x-y=w1070:dbl)
                n442 = Subtract(x=w1082, y=w1059) -> (x-y=w1071:dbl)
                n443 = To Quad Integer(1:w1059) -> (0:w1076:i64)
                n444 = Round To Nearest(number=w1070) -> ()  [unwired: 1 out]
                n445 = Round To Nearest(number=w1071) -> ()  [unwired: 1 out]
                n446 = Index Array(array=w1061, index (dim 1)=w1060, index (dim 2)=w1059) -> (element=→"Slow Time V values at Red cursor":dbl[])  [unwired: 1 in]
                n447 = for {
                  N: "Spectrogram average" -> [_]
                  tunnel: w1060 -> [w1108]
                  tunnel: w1041 -> [w1112]
                  tunnel: w1075 -> [w1111]
                  tunnel: w1076 -> [w1110]
                  tunnel: "Spectrogram average" -> [w1109]
                  tunnel: [w1097] -> w1074 mode=concatenating
                  tunnel: w1055 -> [w1106]
                  tunnel: w1058 -> [w1105]
                  tunnel: w1038 -> [w1104]
                  tunnel: w1057 -> [w1103]
                  tunnel: w1048 -> [w1102]
                  shift-right: [w1100] -> w1052
                  shift-left: _ -> [w1101]
                  tunnel: [w1098] -> w1050 mode=concatenating
                  i -> [w1099]
                  n448 = Add(x=w1099, y=w1108) -> (x+y=w1107:dbl)
                  n449 = for {
                    N: w1109 -> [_]
                    tunnel: w1107 -> [w1128]
                    tunnel: w1112 -> [w1127]
                    tunnel: w1111 -> [w1126]
                    tunnel: w1110 -> [w1118]
                    tunnel: [w1125] -> w1097 mode=indexing
                    tunnel: w1106 -> [w1124]
                    tunnel: w1105 -> [w1123]
                    tunnel: w1104 -> [w1122]
                    tunnel: w1103 -> [w1121]
                    tunnel: w1102 -> [w1120]
                    shift-right: [w1116] -> w1100
                    shift-left: w1101 -> [w1115]
                    tunnel: w1099 -> [w1114]
                    tunnel: [w1113] -> w1098 mode=indexing
                    i -> [w1119]
                    n450 = Add(x=w1118, y=w1119) -> (x+y=w1117:i64)
                    n451 = case shown="False" w1124 {
                      tunnel: w1128 -> [w1132 w1168]
                      tunnel: w1127 -> [_ w1155]
                      tunnel: w1126 -> [_ w1154]
                      tunnel: [_ w1149] -> w1125
                      tunnel: w1123 -> [w1141 _]
                      tunnel: w1122 -> [w1140 _]
                      tunnel: w1121 -> [w1139 _]
                      tunnel: w1120 -> [w1138 _]
                      tunnel: w1117 -> [w1131 w1148]
                      tunnel: [w1135 _] -> w1116
                      tunnel: w1115 -> [w1136 _]
                      tunnel: w1114 -> [w1134 _]
                      tunnel: [w1133 _] -> w1113
                      frame False {
                        (unwired) sgl 0.0
                        n452 = Index Array(array=w1141, index (dim 1)=w1132, index (dim 2)=w1131) -> (element=w1129:cdb[])  [unwired: 1 in]
                        n453 = call "RemoveJump.vi"("frame size"=500, "Input"=w1129) -> ()  [unwired: 9 in, 1 out]
                        n454 = call "HighPassFilterST.vi"("init/cont (init:F)"=FALSE, "Doppler Params"=w1140, "slow time"=w1129) -> ("Filtered X"=w1143:csg[])  [unwired: 6 in, 2 out]
                        n455 = call "Doppler_Spectra.vi"("Thresholds"=w1139, "slow time"=w1143, "Doppler Params"=w1140, "Header In"=w1138) -> ("phase (old Fd AC)"=w1133:sgl[], "Mag Dop Spec"=w1137:dbl[][])  [unwired: 2 in, 8 out]
                        n456 = case shown="0" w1134 {
                          tunnel: w1137 -> [w1144 w1147]
                          tunnel: w1136 -> [_ w1146]
                          tunnel: [w1144 w1145] -> w1135
                          frame 0 {
                          }
                          frame 1, Default {
                            n457 = Add(x=w1146, y=w1147) -> (x+y=w1145:dbl[][])
                          }
                        }
                      }
                      frame True {
                        (unwired) T16."little-endian" ("byte order (0:big-endian, network order)")
                        n458 = call "NumberFileName.vi"("String"=".dat", "Digits"=i16 3 ("d"), "File number"=w1168, "file name"="test") -> ("Numbered File"=w1165:string)
                        n459 = Build Path(base path=path "F:/", name or relative path=w1165) -> (appended path=w1164:path)
                        n460 = Compound Arithmetic op=MULTIPLY(w1155, 1 ("x"), w1148, w1154) -> (w1156:i64)
                        n461 = Open/Create/Replace File(file path (use dialog)=w1164) -> (refnum out=w1163:refnum<file>, error out=w1157:errorcluster)  [unwired: 5 in, 1 out]
                        n462 = Set File Position(offset (in bytes) (0)=w1156, refnum=w1163, from (0:start)=enum16{"start", "end", "current"}."start", error in=w1157) -> (refnum out=w1162:refnum<file>, error out=w1158:errorcluster)
                        n463 = Multiply(x=w1155, y=w1154) -> (x*y=w1153:i32)
                        n464 = Read from Binary File(5:i8 0, 8:w1158, 10:w1153, 11:w1162) -> (0:w1159:errorcluster, 2:w1150:i8[], 3:w1160:refnum<file>)  [unwired: 2 in, 1 out]
                        n465 = To Word Integer(number=w1150) -> (16bit integer=w1149:i16[])
                        n466 = Close File(refnum=w1160, error in=w1159) -> ()  [unwired: 2 out]
                      }
                    }
                  }
                }
                n467 = Multiply(x="Spectrogram average", y="Spectrogram average") -> (x*y=w1056:i32)
                n468 = Transpose 2D Array(2D array=w1050) -> (transposed array=w1051:sgl[][])
                n469 = for {
                  tunnel: w1051 -> [w1088] mode=indexing
                  tunnel: [w1085] -> w1039 mode=indexing
                  n470 = Not Equal To 0?(x=w1088) -> (x != 0?=w1087:bool[])
                  n471 = Add Array Elements(numeric array=w1088) -> (sum=w1086:sgl)
                  n472 = Boolean To (0,1)(Boolean=w1087) -> (0, 1=w1084:i16[])
                  n473 = Add Array Elements(numeric array=w1084) -> (sum=w1083:i16)
                  n474 = Divide(x=w1086, y=w1083) -> (x/y=w1085:sgl)
                }
                n475 = Transpose 2D Array(2D array=w1074) -> (transposed array=w1073:i16[][])
                n476 = Divide(x=w1052, y=w1056) -> (x/y=w1054:dbl[][])
                n477 = for {
                  tunnel: w1073 -> [w1096] mode=indexing
                  tunnel: [w1095] -> w1072 mode=indexing
                  n478 = Add Array Elements(numeric array=w1096) -> (sum=w1095:i16)
                }
                n479 = Build Array(w1039) -> (w1049:sgl[][])
                n480 = for {
                  N: w1041 -> [_]
                  tunnel: [w1089] -> w1067 mode=indexing
                  i -> [w1089]
                }
                n481 = call "DopplerScale.vi"("FFT Length"=w1041, "Header In"=w1048, "Index(F)/Fd"=w1042, "PRF1/2"=w1043, "Velocity index in"=w1049) -> ("output cluster"=w1044:T10, "Velocity Out"=w1047:dbl[][])  [unwired: 3 in, 2 out]
                n482 = Divide(x=w1072, y=w1056) -> (x/y=w1069:dbl[])
                n483 = Index Array(array=w1047) -> (element=w1046:dbl[])  [unwired: 2 in]
                n484 = Reshape Array(w1069, w1075, w1041) -> (w1053:dbl[][])
                n485 = Select(t=w1053, s=w1055, f=w1054) -> (s? t:f=w1045:dbl[][])
                n486 = for {
                  tunnel: w1045 -> [w1091] mode=indexing
                  tunnel: w1067 -> [w1092]
                  tunnel: [w1093] -> w1066 mode=indexing
                  tunnel: "dB width pt" -> [w1090]
                  n487 = call "BeamWidthCalc.vi"("dB width pt"=w1090, "y values"=w1091, "x values"=w1092) -> ("Output variables"=w1094:T17)  [unwired: 6 in, 2 out]
                  n488 = Unbundle By Name(w1094) -> ("bandwidth"=w1093:sgl)
                }
                "bandwidths" <- w1066
                n489 = call "OverlayVelocity.vi"("output cluster"=w1044, "Velocity Out"=w1046, "Mag Dop Spec"=w1045) -> ("Array"=→"Spectrogram at marker":sgl[][])  [unwired: 8 in]
              }
              event "animate", "ms between frames", "AVG Thresh": Value Change {
                # "Build up set of data"
                n490 = event-data() -> ()  [unwired: 1 in, 2 out]
                n491 = property on="Doppler Params" class="Clust (strict)"("Val(Sgnl)"=w1171) -> ()  [unwired: 2 in, 2 out]
                n492 = Unbundle By Name(w1171) -> ("FFT Length"=w1180:i32)
                n493 = call "DopplerScale.vi"("FFT Length"=w1180, "Header In"=w1183, "Index(F)/Fd"=w1181, "PRF1/2"=w1182, "Angle"=w1179) -> ("output cluster"=w1178:T10)  [unwired: 3 in, 3 out]
                n494 = Array Max & Min(array=w1172) -> (max value=w1173:sgl)  [unwired: 3 out]
                n495 = local read "image to display"() -> (w1195:i32)
                n496 = property on="image to display" class="DigNum (strict)"("Val(Sgnl)"=w1195) -> ()  [unwired: 2 in, 2 out]
                n497 = local read "Z Scale"() -> (w1185:dbl)
                n498 = for {
                  tunnel: w1177 -> [w1233] mode=indexing
                  tunnel: "ms between frames" -> [w1258]
                  tunnel: w1183 -> [w1251]
                  tunnel: w1179 -> [w1254]
                  tunnel: [w1247] -> w1188 mode=indexing
                  tunnel: "length" -> [w1253]
                  tunnel: "index" -> [w1252]
                  tunnel: w1171 -> [w1250]
                  tunnel: w1185 -> [w1249]
                  tunnel: [w1242] -> w1184 mode=indexing
                  tunnel: w1178 -> [w1241]
                  tunnel: w1177 -> [w1238]
                  tunnel: [w1231] -> w1176 mode=indexing
                  tunnel: [w1229] -> w1175 mode=indexing
                  tunnel: w1174 -> [w1228]
                  tunnel: w1173 -> [w1225]
                  tunnel: w1172 -> [w1222] mode=indexing
                  i -> [w1232]
                  w1234 = TRUE ("Override min fill?")
                  n499 = Wait (ms)(milliseconds to wait=w1258) -> ()  [unwired: 1 out]
                  n500 = Divide(x=w1222, y=w1225) -> (x/y=w1224:sgl[][])
                  n501 = expression code="20*log(x)"(w1224) -> (→"Mean Power":sgl[][])
                  n502 = Unbundle By Name(w1250) -> ("Window Increment"=w1237:i32)
                  n503 = case shown="1, Default" w1254 {
                    tunnel: w1233 -> [w1259 w1263]
                    tunnel: w1251 -> [_ w1262]
                    tunnel: w1254 -> [_ w1261]
                    tunnel: [w1259 w1260] -> w1247
                    frame 0 {
                    }
                    frame 1, Default {
                      n504 = call "RotateArray.vi"("Peak V in"=w1263, "Header In"=w1262, "Angle"=w1261) -> ("Peak V out"=w1260:dbl[][])  [unwired: 7 in, 1 out]
                    }
                  }
                  "Peak V" <- w1247
                  n505 = Unbundle By Name(w1241) -> ("X Scale Mult"=w1244:dbl)
                  n506 = Multiply(x=w1237, y=w1232) -> (x*y=w1227:i32)
                  n507 = Index Array(array=w1228, index (dim 0)=w1227) -> (element=w1226:cdb[][])  [unwired: 2 in]
                  n508 = Array Subset(array=w1238, index (dim 0)=w1232, length (dim 0)="ST AV depth") -> (w1236:dbl[][][])  [unwired: 4 in]
                  n509 = Multiply(x=w1244, y=w1237) -> (x*y=w1243:dbl)
                  n510 = call "SmoothImage.vi"("sector array in"=w1226, "Override min fill?"=w1234, "Av size"="Med Size") -> ("Smoothed Sector w/Ave"=w1239:cdb[][])  [unwired: 1 in, 3 out]
                  n511 = Array Subset(array=w1247, index (row)=w1252, length (row)=w1253) -> (w1256:dbl[][])  [unwired: 2 in]
                  n512 = call "SmoothImage.vi"("sector array in"=w1247, "Override min fill?"=w1234, "Av size"="Med Size") -> ("Smoothed Sector w/Ave"=w1229:cdb[][])  [unwired: 1 in, 3 out]
                  n513 = Absolute Value(x=w1239) -> (abs(x)=w1240:dbl[][])
                  n514 = call "SmoothImage3D.vi"("sector array in"=w1236, "Override min fill?"=w1234, "Av size"="Med Size") -> ("Smoothed Sector w/Ave"=w1231:cdb[][])  [unwired: 1 in, 3 out]
                  n515 = Multiply(x=w1232, y=w1243) -> (x*y=w1245:dbl)
                  n516 = Transpose 2D Array(2D array=w1256) -> (transposed array=w1257:dbl[][])
                  n517 = expression code="20*log(x)"(w1240) -> ()  [unwired: 1 out]
                  n518 = for {
                    tunnel: w1257 -> [w1264] mode=indexing
                    tunnel: [w1265] -> w1255 mode=indexing
                    n519 = call-poly <vilib>:"Mean.vi"("X"=w1264) -> ("mean"=w1265:dbl)  [unwired: 1 out]
                  }
                  "Avergae V Profile (Tube)" <- w1255
                  n520 = property on="Spectrogram at marker" class="IntGraph (strict)"("Active Cursor"=u32 1, "Cursor.Cursor X"=w1245, "XScale.Multiplier"=w1243) -> ()  [unwired: 2 in, 2 out]
                  n521 = call "SplitOverlay.vi"("dB Max"="dB Max", "Raw data"=w1226, "Doppler Data"=w1229, "Z Scale"=w1249) -> ("Overlay"=w1242:i16[][])  [unwired: 7 in]
                  "Overlay" <- w1242
                }
                "Overlay 3D" <- w1184
                "Smoothed Data" <- w1176
                "AVG Vel" <- w1175
                n522 = for {
                  N: 1 -> [_]
                  tunnel: w1188 -> [w1202] mode=indexing
                  tunnel: w1188 -> [w1201]
                  tunnel: [w1200] -> w1186
                  tunnel: "AVG Thresh" -> [w1199]
                  n523 = for {
                    tunnel: w1202 -> [w1207] mode=indexing
                    tunnel: w1201 -> [w1206]
                    tunnel: [w1204] -> w1200 mode=indexing
                    tunnel: w1199 -> [w1203]
                    i -> [w1205]
                    n524 = for {
                      tunnel: w1207 -> [_] mode=indexing
                      tunnel: w1206 -> [w1218]
                      tunnel: w1205 -> [w1220]
                      tunnel: [w1219] -> w1204 mode=indexing
                      tunnel: w1203 -> [w1209]
                      i -> [w1221]
                      n525 = Index Array(array=w1218, index (dim 1)=w1220, index (dim 2)=w1221) -> (element=w1208:dbl[])  [unwired: 1 in]
                      n526 = call <vilib>:"Std Deviation and Variance.vi"("X"=w1208) -> ("mean"=w1214:dbl, "standard deviation"=w1213:dbl)  [unwired: 1 in, 1 out]
                      n527 = Absolute Value(x=w1214) -> (abs(x)=w1212:dbl)
                      n528 = Divide(x=w1213, y=w1212) -> (x/y=w1210:dbl)
                      n529 = Greater?(x=w1210, y=w1209) -> (0:w1211:bool)
                      n530 = Multiply(x=0, y=w1208) -> (x*y=w1215:dbl[])
                      n531 = Select(t=w1215, s=w1211, f=w1208) -> (s? t:f=w1216:dbl[])
                      n532 = call-poly <vilib>:"Mean.vi"("X"=w1216) -> ("mean"=w1219:dbl)  [unwired: 1 out]
                    }
                  }
                }
                "AVG of all windows" <- w1186
                n533 = Array Subset(array=w1186, index (row)="index", length (row)="length") -> (w1191:dbl[][])  [unwired: 2 in]
                n534 = Transpose 2D Array(2D array=w1191) -> (transposed array=w1193:dbl[][])
                n535 = for {
                  tunnel: w1193 -> [w1197] mode=indexing
                  tunnel: [w1198] -> w1192 mode=indexing
                  n536 = call-poly <vilib>:"Mean.vi"("X"=w1197) -> ("mean"=w1198:dbl)  [unwired: 1 out]
                }
                "Avergae V Profile All" <- w1192
              }
              event "Save Single SpGram": Value Change {
                n537 = event-data() -> ()  [unwired: 1 in, 2 out]
                n538 = invoke on="Spectrogram at marker" class="IntGraph (strict)" method="Get Image"("image depth"=24 ("Image Depth"), "bg color"=u32 0 ("Background Color")) -> ("image data"=w1267:T11)  [unwired: 4 in, 5 out]
                n539 = call <vilib>:"Unflatten Pixmap.vi"("image data"=w1267) -> ("24-bit pixmap"=w1266:u32[][])  [unwired: 10 out]
                n540 = call <vilib>:"Flatten Pixmap.vi"("24-bit pixmap"=w1266) -> ("image data"=w1268:T11)  [unwired: 5 in, 5 out]
                n541 = call <vilib>:"Write JPEG File.vi"("image data"=w1268) -> ()  [unwired: 9 in, 2 out]
              }
              event "Spectrogram at marker": Cursor Release {
                n542 = event-data() -> ("CursLoc"=w1291:cluster{"X":dbl, "Y":dbl})  [unwired: 1 in]
                n543 = property on="Spectrogram at marker" class="IntGraph (strict)"() -> ("XScale.Multiplier"=w1289:dbl)  [unwired: 2 in, 2 out]
                n544 = Unbundle By Name(w1291) -> ("X"=w1290:dbl)
                n545 = Divide(x=w1290, y=w1289) -> (x/y=w1285:dbl)
                n546 = Unbundle By Name(w1276) -> ("Window Increment"=w1286:i32)
                n547 = local read "Spectrogram at marker"() -> (w1288:sgl[][])
                n548 = Multiply(x=w1285, y=w1286) -> (x*y=w1274:dbl)
                n549 = local read "Overlay 3D"() -> (w1293:i16[][][])
                n550 = Index Array(array=w1288, index (row)=w1285) -> (element=→"Dop Spectrum":sgl[])  [unwired: 1 in]
                n551 = Index Array(array=w1293, index (dim 0)=w1285) -> (element=w1292:i16[][])  [unwired: 2 in]
                n552 = local write "Overlay"(w1292) -> ()
                n553 = Index Array(array=w1275, index (dim 0)=w1274) -> (element=w1281:cdb[][])  [unwired: 2 in]
                n554 = call "SmoothImage.vi"("sector array in"=w1281, "Override min fill?"=TRUE, "Av size"=3) -> ("Smoothed Sector w/Ave"=w1282:cdb[][])  [unwired: 1 in, 3 out]
                n555 = Absolute Value(x=w1282) -> (abs(x)=w1283:dbl[][])
                n556 = expression code="20*log(x)"(w1283) -> (w1280:dbl[][])
                n557 = Array Max & Min(array=w1280) -> (max value=w1284:dbl)  [unwired: 3 out]
                n558 = Subtract(x=w1280, y=w1284) -> (x-y=→"Raw uncropped image":dbl[][])
              }
              event "Z Scale", "Scale Type": Value Change {
                n559 = event-data() -> ()  [unwired: 1 in, 6 out]
                n560 = case shown="\"Max/Min\", Default" "Scale Type" {
                  tunnel: "Z Scale" -> [w1306 w1308 w1310]
                  tunnel: [w1305 w1307 w1309] -> w1301
                  tunnel: [w1305 w1307 w1309] -> w1300
                  tunnel: [w1306 w1308 w1311] -> w1298
                  tunnel: [w1306 w1308 w1311] -> w1297
                  frame "Max/Min", Default {
                    n561 = Negate(x=w1306) -> (-x=w1305:dbl)
                  }
                  frame "Max/Zero" {
                    w1307 = 0.0
                  }
                  frame "Min/Zero" {
                    w1311 = 0.0 ("Z Scale")
                    n562 = Negate(x=w1310) -> (-x=w1309:dbl)
                  }
                }
                n563 = property on="Peak V" class="IntGraph (strict)"("ZScale.Maximum"=w1298, "ZScale.Minimum"=w1301) -> ()  [unwired: 2 in, 2 out]
                n564 = property on="AVG of all windows" class="IntGraph (strict)"("ZScale.Maximum"=w1297, "ZScale.Minimum"=w1300) -> ()  [unwired: 2 in, 2 out]
              }
              event "CFiltered data": Value Change {
                n565 = event-data() -> ()  [unwired: 1 in, 1 out]
                n566 = Array Size(array=w1326) -> (size(s)=w1324:i32[])
                n567 = Index Array(array=w1324, index=1) -> (element=w1314:i32)
                n568 = for {
                  N: w1314 -> [_]
                  tunnel: w1326 -> [w1336]
                  tunnel: [w1338] -> w1321 mode=indexing
                  tunnel: w1312 -> [w1337]
                  i -> [w1333]
                  n569 = Index Array(array=w1336, index (dim 1)=w1333) -> (element=w1335:cdb[][])  [unwired: 2 in]
                  n570 = Transpose 2D Array(2D array=w1335) -> (transposed array=w1334:cdb[][])
                  n571 = for {
                    tunnel: [w1343] -> w1338 mode=indexing
                    tunnel: w1337 -> [w1341]
                    tunnel: w1334 -> [w1340] mode=indexing
                    workers-P: _ -> [_]
                    n572 = call "HighPassFilterST.vi"("init/cont (init:F)"=FALSE, "Doppler Params"=w1341, "slow time"=w1340) -> ("Filtered X"=w1342:csg[])  [unwired: 6 in, 2 out]
                    n573 = Absolute Value(x=w1342) -> (abs(x)=w1343:sgl[])
                  }
                }
                n574 = Unbundle By Name(w1312) -> ("Window Increment"=w1316:i32)
                n575 = Array Size(array=w1321) -> (size(s)=w1323:i32[])
                n576 = Index Array(array=w1323, index=2) -> (element=w1313:i32)
                n577 = Divide(x=w1313, y=w1316) -> (x/y=w1317:dbl)
                n578 = Round Toward -Infinity(1:w1317) -> ()  [unwired: 1 out]
                n579 = for {
                  N: w1313 -> [_]
                  tunnel: w1321 -> [w1332]
                  tunnel: [w1330] -> w1320 mode=indexing
                  tunnel: u32 10 ("ms between frames") -> [w1329]
                  i -> [w1327]
                  n580 = Wait (ms)(milliseconds to wait=w1329) -> ()  [unwired: 1 out]
                  n581 = Index Array(array=w1332, index (dim 2)=w1327) -> (element=w1330:sgl[][])  [unwired: 2 in]
                  n582 = Absolute Value(x=w1330) -> (abs(x)=w1331:sgl[][])
                  n583 = expression code="20*log(x)"(w1331) -> (w1328:sgl[][])
                  n584 = local write "High pass Filtered log"(w1328) -> ()
                }
                "HIgh pass Filtered X" <- w1320
              }
              event "C Corr": Value Change {
                n585 = event-data() -> ()  [unwired: 1 in, 6 out]
                n586 = local read "HIgh pass Filtered X"() -> (w1346:sgl[][][])
                n587 = Index Array(array=w1346, index (dim 0)=118 ("index (page)")) -> (element=w1351:sgl[][])  [unwired: 2 in]
                n588 = Array Subset(array=w1351, index (row)=133 ("index"), length (row)=11 ("length"), index (col)=34 ("index"), length (col)=6 ("length")) -> (w1349:sgl[][])
                n589 = Absolute Value(x=w1349) -> (abs(x)=w1347:sgl[][])
                n590 = Absolute Value(x=w1346) -> (abs(x)=w1348:sgl[][][])
                n591 = for {
                  tunnel: w1348 -> [w1359] mode=indexing
                  tunnel: [w1360] -> w1352 mode=indexing
                  tunnel: w1347 -> [w1358]
                  workers-P: _ -> [_]
                  n592 = call-poly <vilib>:"CrossCorrelation.vi"("Y"=w1359, "X"=w1358) -> ("Rxy"=w1360:dbl[][])  [unwired: 8 in, 1 out]
                }
                "Cross Correlate" <- w1352
              }
              event "AVG of all windows": Cursor Release {
                # "Take an avergag of all slow time estimates in window marked by cursors"
                n593 = event-data() -> ()  [unwired: 1 in, 9 out]
                n594 = property on="AVG of all windows" class="IntGraph (strict)"("Active Cursor"=u32 0, "Active Cursor"=u32 1) -> ("Cursor.Cursor X"=w1366:dbl, "Cursor.Cursor Y"=w1365:dbl, "Cursor.Cursor X"=w1377:dbl, "Cursor.Cursor Y"=w1378:dbl)  [unwired: 2 in, 2 out]
                n595 = Subtract(x=w1378, y=w1365) -> ()  [unwired: 1 out]
                n596 = Subtract(x=w1377, y=w1366) -> ()  [unwired: 1 out]
                n597 = for {
                  tunnel: w1366 -> [w1389]
                  tunnel: u32 3 ("Active Cursor") -> [w1388]
                  tunnel: w1365 -> [w1387]
                  tunnel: u32 3 ("Active Cursor") -> [w1386]
                  tunnel: [w1379] -> w1373 mode=indexing
                  tunnel: w1367 -> [w1385] mode=indexing
                  tunnel: [w1383] -> w1363 mode=indexing
                  tunnel: [w1380] -> _ mode=indexing
                  n598 = Array Subset(array=w1385, index (row)=w1389, length (row)=w1388, index (col)=w1387, length (col)=w1386) -> (w1379:dbl[][])
                  n599 = Array Size(array=w1379) -> (size(s)=w1382:i32[])
                  n600 = Multiply Array Elements(1:w1382) -> (0:w1381:i32)
                  n601 = Reshape Array(w1379, w1381) -> (w1384:dbl[])
                  n602 = call <vilib>:"Std Deviation and Variance.vi"("X"=w1384) -> ("mean"=w1383:dbl, "standard deviation"=w1380:dbl)  [unwired: 1 in, 1 out]
                }
                "Slow time mean" <- w1363
                n603 = Array Size(array=w1373) -> (size(s)=w1372:i32[])
                n604 = Multiply Array Elements(1:w1372) -> (0:w1371:i32)
                n605 = Reshape Array(w1373, w1371) -> (w1370:dbl[])
                n606 = call <vilib>:"Std Deviation and Variance.vi"("X"=w1370) -> ("mean"=→"V mean":dbl, "standard deviation"=→"V SD":dbl)  [unwired: 1 in, 1 out]
              }
              event "Mean Power": Cursor Release {
                n607 = event-data() -> ()  [unwired: 1 in, 9 out]
                n608 = property on="Mean Power" class="IntGraph (strict)"() -> ("Cursor.Cursor X"=w1393:dbl, "Cursor.Cursor Y"=w1392:dbl)  [unwired: 2 in, 2 out]
                n609 = Index Array(array=w1390, index (dim 1)=w1393, index (dim 2)=w1392) -> (element=→"Slow Time V values at Red cursor Mean Power":dbl[])  [unwired: 1 in]
              }
              event "Choose Directory", "# of files": Value Change {
                n610 = event-data() -> ()  [unwired: 1 in, 6 out]
              }
              event "Save Animation": Value Change {
                # "Save sequence as images"
                n611 = event-data() -> ()  [unwired: 1 in, 2 out]
                n612 = local read "Choose Directory"() -> (w1406:path)
                n613 = Strip Path(path=w1406) -> (stripped path=w1402:path, name=w1403:string)
                n614 = Concatenate Strings(w1403, "Doppler" ("String")) -> (w1401:string)
                n615 = Build Path(base path=w1402, name or relative path=w1401) -> (appended path=w1405:path)
                n616 = call <vilib>:"Check if File or Folder Exists.vi"("path"=w1405) -> ("file or folder exists?"=w1400:bool, "dup path"=w1408:path)  [unwired: 8 in, 1 out]
                n617 = case shown="False" w1400 {
                  tunnel: w1408 -> [w1413 w1415]
                  tunnel: [w1414 w1415] -> w1407
                  frame False {
                    n618 = Create Folder(path (use dialog)=w1413) -> (created path=w1414:path)  [unwired: 2 in, 2 out]
                  }
                  frame True {
                  }
                }
                n619 = local read "Overlay 3D"() -> (w1409:i16[][][])
                n620 = for {
                  tunnel: w1409 -> [w1418] mode=indexing
                  tunnel: w1403 -> [w1422]
                  tunnel: w1407 -> [w1419]
                  i -> [w1420]
                  (unwired) u32[] [0, 0, 65793, 131586, 197379, 263172, 328965, 394758, 460551, 526344, 592137, 657930, 723723, 789516, 855309, 921102, 986895, 1052688, 1118481, 1184274, 1250067, 1315860, 1381653, 1447446, 1513239, 1579032, 1644825, 1710618, 1776411, 1842204, 1907997, 1973790, 2039583, 2105376, 2171169, 2236962, 2302755, 2368548, 2434341, 2500134, 2565927, 2631720, 2697513, 2763306, 2829099, 2894892, 2960685, 3026478, 3092271, 3158064, 3223857, 3289650, 3355443, 3421236, 3487029, 3552822, 3618615, 3684408, 3750201, 3815994, 3881787, 3947580, 4013373, 4079166, 4144959, 4210752, 4276545, 4342338, 4408131, 4473924, 4539717, 4605510, 4671303, 4737096, 4802889, 4868682, 4934475, 5000268, 5066061, 5131854, 5197647, 5263440, 5329233, 5395026, 5460819, 5526612, 5592405, 5658198, 5723991, 5789784, 5855577, 5921370, 5987163, 6052956, 6118749, 6184542, 6250335, 6316128, 6381921, 6447714, 6513507, 6579300, 6645093, 6710886, 6776679, 6842472, 6908265, 6974058, 7039851, 7105644, 7171437, 7237230, 7303023, 7368816, 7434609, 7500402, 7566195, 7631988, 7697781, 7763574, 7829367, 7895160, 7960953, 8026746, 8092539, 8158332, 8224125, 8289918, 8355711, 8421504, 8487297, 8553090, 8618883, 8684676, 8750469, 8816262, 8882055, 8947848, 9013641, 9079434, 9145227, 9211020, 9276813, 9342606, 9408399, 9474192, 9539985, 9605778, 9671571, 9737364, 9803157, 9868950, 9934743, 10000536, 10066329, 10132122, 10197915, 10263708, 10329501, 10395294, 10461087, 10526880, 10592673, 10658466, 10724259, 10790052, 10855845, 10921638, 10987431, 11053224, 11119017, 11184810, 11250603, 11316396, 11382189, 11447982, 11513775, 11579568, 11645361, 11711154, 11776947, 11842740, 11908533, 11974326, 12040119, 12105912, 12171705, 12237498, 12303291, 12369084, 12434877, 12500670, 12566463, 12632256, 12698049, 12763842, 12829635, 12895428, 12961221, 13027014, 13092807, 13158600, 13224393, 13290186, 13355979, 13421772, 13487565, 13553358, 13619151, 13684944, 13750737, 13816530, 13882323, 13948116, 14013909, 14079702, 14145495, 14211288, 14277081, 14342874, 14408667, 14474460, 14540253, 14606046, 14671839, 14737632, 14803425, 14869218, 14935011, 15000804, 15066597, 15132390, 15198183, 15263976, 15329769, 15395562, 15461355, 15527148, 15592941, 15658734, 15724527, 15790320, 15856113, 15921906, 15987699, 16053492, 16119285, 16185078, 16250871, 16316664, 16382457, 16448250, 16514043, 16579836, 16645629, 16448250] ("Array 2")
                  n621 = flat-sequence {
                    tunnel: w1418 -> [w1428]
                    tunnel: [24] -> w1417
                    frame #0 {
                      n622 = local write "Overlay"(w1428) -> ()
                    }
                  }
                  n623 = invoke on="Overlay" class="IntGraph (strict)" method="Get Image"("image depth"=w1417) -> ("image data"=w1421:T11)  [unwired: 5 in, 5 out]
                  n624 = call "NumberFileName.vi"("String"=".jpg", "File number"=w1420, "file name"=w1422) -> ("Numbered File"=w1425:string)  [unwired: 1 in]
                  n625 = call <vilib>:"Unflatten Pixmap.vi"("image data"=w1421) -> ("24-bit pixmap"=w1416:u32[][])  [unwired: 10 out]
                  n626 = Build Path(base path=w1419, name or relative path=w1425) -> (appended path=w1426:path)
                  n627 = call <vilib>:"Flatten Pixmap.vi"("24-bit pixmap"=w1416) -> ("image data"=w1424:T11)  [unwired: 5 in, 5 out]
                  n628 = call <vilib>:"Write JPEG File.vi"("image data"=w1424, "path to JPEG file"=w1426) -> ()  [unwired: 8 in, 2 out]
                }
              }
            }
            n629 = Or(x=w212, y="stop") -> (x .or. y?=w213:bool)
          }
        }
      }
      n630 = Or(x=w43, y=w42) -> (x .or. y?=w41:bool)
    }
  }
